vi "ControlProgram6.6_3.vi"() -> ()   [LabVIEW 2016]
uses:
  <vilib>/Utility/miscctls.llb/LVPoint32TypeDef.ctl
  <vilib>/Platform/TimedLoop/XDataNode/timing_clust.ctl
  <vilib>/Platform/TimedLoop/XDataNode/nitl_modes.ctl
  <vilib>/Platform/TimedLoop/XDataNode/wakeup.ctl
  <vilib>/Instr/_visa.llb/Select Event Type.ctl
  <vilib>/vision/Avi1.llb/AviRefnum.ctl
  <vilib>/Utility/error.llb/DialogType.ctl
  <vilib>/DAQmx/write.llb/DAQmx Write (Analog 1D DBL NChan 1Samp).vi
  <vilib>/DAQmx/read.llb/DAQmx Read (Analog 2D DBL NChan NSamp).vi
  <vilib>/Analysis/baseanly.llb/Mean (DBL).vi
  <vilib>/DAQmx/write.llb/DAQmx Write (Digital Bool 1Line 1Point).vi
  <vilib>/DAQmx/create/channels.llb/DAQmx Create Channel (DO-Digital Output).vi
  <vilib>/DAQmx/create/channels.llb/DAQmx Create Channel (AI-Voltage-Basic).vi
  <vilib>/DAQmx/create/channels.llb/DAQmx Create Channel (AO-Voltage-Basic).vi
  <vilib>/DAQmx/configure/timing.llb/DAQmx Timing (Sample Clock).vi
  <vilib>/DAQmx/miscellaneous.llb/DAQmx Fill In Error Info.vi
  <vilib>/Instr/_visa.llb/VISA Configure Serial Port (Instr).vi
  Arnulf--joystick/git(most_up_to_date)/Logitech-joystick/Old Trap/FAST_Global_var.vi
  <vilib>/Utility/inputDevices.llb/mouseAcquire.vi
  <vilib>/Utility/inputDevices.llb/closeMouse.vi
  <vilib>/platform/TimedLoop/XDataNode/XDataNode.xnode
  <vilib>/Platform/TimedLoop/XDataNode/XDNodeRunTimeDep.lvlib
  <resource>/objmgr/daqmx.rc
  <vilib>/Analysis/NI_AALBase.lvlib
panel:
  out "Saving Move":bool
  out "Move time":string
  out "Primary Video Display":T1(plugin-control)
  in  "Save file index":i32
  out "Flush Sample Start Time":u32=2111292881
  out "Sample flush time (s)":dbl=48.0
  in  "Inject Sample":bool
  out "Cal values":T2={"AX alpha"=612.9626061060078, "BX alpha"=549.6584469744151, "AX kappa"=0.3485731373010688, "BX kappa"=0.3853424216291352, "AX offset"=-0.03900484438240665, "BX offset"=-0.11295550662085417, "AY alpha"=582.7562541114835, "BY alpha"=571.1587543790358, "AY kappa"=0.37498408087930674, "BY kappa"=0.36252029651198364, "AY offset"=-0.21125584642206058, "BY offset"=-0.12469077200400738}
  in  "Inject Pump 1":bool
  in  "Inject Pump 2":bool
  in  "Tab Control 2":T3(tab)
  in  "Force FB script":bool
  in  "Got ADig bead":bool
  in  "Move Cap. 2 (ADig Top)":bool
  in  "Dump beads":bool
  in  "Got DNA bead":bool
  in  "Flow on\ncap 2?":bool=TRUE
  in  "Flow on\ncap 1?":bool=TRUE
  in  "Flow on\ndump?":bool=TRUE
  in  "Raster set":i32=1
  in  "Fish After TA?":bool=TRUE
  in  "Delta after tether":dbl=1700.0
  in  "TA Cancel Save?":bool=TRUE
  in  "Min fish\ndelta (nm)":dbl=1425.0 min=0.0 max=5000.0 step=50.0
  in  "Max fish\ndelta (nm)":dbl=1900.0 min=0.0 max=5000.0 step=25.0
  in  "Fish Speed (ms)":i32=5000
  in  "Wait (ms)":i32=1500
  in  "# attempts":dbl=10.0
  in  "Cutoff force (pN)":dbl=4.5
  in  "Raster after\n tether?":bool=TRUE
  out "Tether":bool
  out "Attempt #":i32
  in  "Flow on\nwhile fish?":bool=TRUE
  in  "Flow on\nafter raster?":bool=TRUE
  in  "Offset raster set":i32
  in  "Offset @ Delta (nm)":dbl=1700.0
  in  "Cal @ Delta (nm)":dbl=2500.0
  in  "Cal stage position":i32=3
  out "Cal Final Sampling Rate":dbl=125000.0
  in  "Cal Averaging":i32=1
  in  "Wait before dip (s)":dbl=3.0
  in  "Start dipping after?":bool
  in  "Start trap delta (nm)":dbl=1700.0
  in  "Continous Dip":bool
  out "Dip #":i32
  in  "Dip attempts":dbl=3.0
  in  "Cancel Dip":bool
  out "Return elasped time":i32
  in  "Return duration":dbl=15.0
  in  "Cancel dwell":bool=TRUE
  in  "Pause dwell":bool
  in  "Start/Return position":dbl=3.0
  in  "Dip duration":dbl=15.0
  in  "Dip position":dbl=4.0
  in  "Dip":bool
  out "Dip elasped time":i32
  in  "Stop":bool=TRUE
  in  "?":T4(tab)
  out "FAST X-Y":bool
  out "FAST Z":bool
  in  "Cal time (s)":dbl=5.0
  in  "Save N sets":bool
  in  "N sets":i32=200
  out "Cal sets to save":i32=500
  in  "Reset data stream":bool
  out "Buffer Overflow":bool
  out "Stage moving":bool
  in  "Comment":string
  in  "Raster scan":bool
  out "Saving":bool
  in  "Save cal":bool
  in  "Save Data":bool
  in  "Stop saving":bool
  out "Calibrating":bool
  out "Progress":dbl(slide) scale=0.0..100.0
  in  "Read Cal":bool
  in  "Fish":bool
  in  "Averaging Number":i32=1250
  out "Final Sampling Rate":dbl=100.0
  in  "Trap position (V)":cluster{"X":dbl, "Y":dbl}={"X"=3.9042624789680316, "Y"=0.2}
  in  "Trap delta (nm)":dbl=2500.0 min=0.0 max=5000.0 step=50.0
  in  "Fixed X":dbl=1.1
  in  "Fixed Y":dbl=0.15
  in  "Shutter 1 (B)":bool
  in  "Shutter 2 (A)":bool
  in  "Pulling direction":bool
  out "Raster scanning...":bool
  out "Current file name":path=path "D:/data/160111/160111_006.dat"
  in  "AX alpha":dbl=612.9626061060078 format="%#_3p"
  in  "BX alpha":dbl=549.6584469744151 format="%#_3g"
  in  "AX kappa":dbl=0.3485731373010688 format="%#_3g"
  in  "BX kappa":dbl=0.3853424216291352 format="%#_3g"
  in  "AX offset":dbl=-0.03900484438240665 format="%#_3g"
  in  "BX offset":dbl=-0.11295550662085417 format="%#_3g"
  in  "AY alpha":dbl=582.7562541114835 format="%#_3g"
  in  "BY alpha":dbl=571.1587543790358 format="%#_3g"
  in  "AY kappa":dbl=0.37498408087930674 format="%#_3g"
  in  "BY kappa":dbl=0.36252029651198364 format="%#_3g"
  in  "AY offset":dbl=-0.21125584642206058 format="%#_3g"
  in  "BY offset":dbl=-0.12469077200400738 format="%#_3g"
  out "Buffer status":u8(slide) scale=0.0..100.0
  in  "Target":bool
  in  "Set Current\nPos to (0,0,0)":bool
  in  "dump spot":string="Dump beads spot"
  in  "up flow spot":string="Upper flow spot"
  in  "low flow spot":string="Lower flow spot"
  in  "up cap":string="Upper capillary (ADig beads)"
  in  "bottom cap":string="Lower capillary (DNA beads)"
  in  "Move to Position 5":bool
  in  "Set Position 5":bool
  in  "Saved stage positions":dbl[][](array[numeric])=[[1.0, 0.0, 0.0, 0.0], [2.0, -0.13716, -3.21132, 0.01436], [3.0, 0.45, -0.73974, 0.005], [4.0, 0.45, -2.1978, 0.005], [5.0, 0.45, -2.63158, -0.02256]]
  in  "Set Position 2":bool
  in  "Move to Position 2":bool
  in  "Set Position 1":bool
  in  "Move to Position 1":bool
  in  "Set Position 4":bool
  in  "Move to Position 4":bool
  in  "Set Position 3":bool
  in  "Move to Position 3":bool
  out "Stage error":errorcluster
  in  "Clear Volume":bool
  out "Sample Flush Meter":u8(slide) scale=0.0..100.0
  out "Flushing Sample":bool
  in  "Flush Sample":bool
  in  "Normal \nRate (ul/hr)  3":dbl=100.0
  in  "Normal \nVolume (ul) 3":dbl=250.0
  in  "Normal \nVolume (ul) 2":dbl
  in  "Normal \nRate (ul/hr)":dbl
  in  "Normal \nVolume (ul)":dbl
  in  "Flush\nRate (ul/min)":dbl
  in  "Flush\nVolume (ul)":dbl
  in  "Flush \nRate (ul/min)  2":dbl
  in  "Flush Pump 2":bool
  in  "Flush\nVolume (ul)  2":dbl
  in  "Flush Pump 1":bool
  in  "Normal \nRate (ul/hr)  2":dbl
  in  "Write Wait":i32=1000
  in  "Flush \nRate (ul/min)  3":dbl=100.0
  in  "Flush\nVolume (ul)  3":dbl=80.0
  out "error out":errorcluster
  in  "Use Mouse to Move Trap?":bool
  in  "Pause Mouse/Mirror Connection":bool
  out "Reference Voltage":cluster{dbl, dbl}={0.0, -0.0}
  out "Saved voltage":cluster{dbl, dbl}={5.766666666666665, 1.45}
  out "Real Coordinates":cluster{"Horizontal":i32, "Vertical":i32}={"Horizontal"=897, "Vertical"=-1271}
  out "CoordinatesMousePressed":T5
  in  "Force Feedback 2":bool
  in  "Offset 2":cluster{"Off Y":dbl, "Off X":dbl}={"Off Y"=1.5, "Off X"=0.17}
  in  "Setpoint voltage 2":cluster{"SP Y":dbl, "SP X":dbl}={"SP Y"=0.6, "SP X"=0.0}
  out "Sum error":dbl(knob) scale=-0.2..0.2
  out "Trap sep":waveform(dbl)[](graph)=[{"t0"=timestamp(4.489999999999949 s since 1904-01-01), "dt"=0.002, "Y"=[-1157.7639781743756, -1157.678951177374, -1157.7582331070425, -1157.7490409992681, -1157.8995617642552], "attributes"=variant("NI_ChannelName"=variant(string "T2 X"))}, {"t0"=timestamp(4.489999999999949 s since 1904-01-01), "dt"=0.002, "Y"=[-909.0775466981794, -909.1316439023619, -909.1322956759037, -909.1570630705896, -909.1264297140281], "attributes"=variant("NI_ChannelName"=variant(string "T2 Y"))}]
  in  "Set reading to\nsetpoint 1":bool
  in  "Offset Y (nm)":dbl format="%0.2f"
  in  "Offset X (nm)":dbl format="%0.2f"
  in  "Remove offsets":bool
  in  "Force Feedback 1":bool
  out "Feedback Output \nVoltage 2":cluster{dbl, dbl} {"?" format="%#_4g"; "?" format="%#_4g"}
  in  "Offset 1":cluster{"Off Y":dbl, "Off X":dbl}={"Off Y"=1.5, "Off X"=0.17}
  in  "Setpoint voltage 1":cluster{"SP Y":dbl, "SP X":dbl}={"SP Y"=0.6, "SP X"=0.0}
  in  "Feedback const":T6={"Ki_B_Y"=0.5, "Ki_B_X"=0.0, "Kp Y"=1.0, "Kp X"=0.0}
  out "Mean Trap Pos X 2 (nm)":dbl=-1157.769953044463 format="%0.2f"
  out "Mean Trp Pos Y 2 (nm)":dbl=-909.1249958122125 format="%0.2f"
  out "T2 X RMS (A)":dbl=0.7168002469275427 format="%0.2f"
  out "T2 Y RMS (A)":dbl=0.25997187037503383 format="%0.2f"
  in  "Set reading to\nsetpoint 2":bool
  in  "Scan range (nm)":dbl=425.0
  in  "Scan speed (nm/s)":dbl=100.0 min=0.0 max=100.0
  in  "Step size (nm)":dbl=1.0
  in  "Save scans":bool=TRUE
  in  "# scans":i32=1
  in  "Load param":bool
  in  "Scan Parameters":T7(array[cluster])
  in  "Trap delta\nafter (nm)":dbl=1550.0
  in  "Stop raster":bool
  out "Scan range (V)":dbl=0.47672462142456534
  out "Scan steps (mirror)":u64=425
  out "Scan increment (V)":dbl=0.0011217049915872126
  out "Time per step (ms)":dbl=10.0
  out "Total raster time (s)":dbl=8.5
  out "N sets to be saved":dbl=850.0
  in  "Zoom Factor":sgl=7.0
  in  "Center Point":cluster{"X":i32, "Y":i32}={"X"=335, "Y"=271}
  in  "Intensity Upper":dbl=88.0
  in  "Intensity Lower":dbl=66.0
  out "Window Size":cluster{"Height":i32, "Width":i32}
  in  "Image Index":dbl=1.0 min=1.0
  in  "Save Image":bool
  in  "Averaging":bool
  in  "Reset Averaging":bool
  in  "Save Video":bool
  in  "New Video File":bool
  in  "Video Index":dbl=1.0 min=1.0 step=1.0
  in  "Video Capture Rate (Hz)":dbl=30.0
  in  "Initial Window Size":cluster{"Width":i32, "Height":i32}={"Width"=884, "Height"=619}
  in  "Initial Window Position":cluster{"X Position":i32, "Y Position":i32}={"X Position"=796, "Y Position"=4}
  out "Window Position":cluster{"X Position":i32, "Y Position":i32}={"X Position"=40, "Y Position"=40}
  out "Path Out":path
  in  "Target coordinates":cluster{"X1":dbl, "Y1":dbl, "X2":dbl, "Y2":dbl}={"X1"=328.0, "Y1"=274.0, "X2"=368.0, "Y2"=314.0}
  in  "# Samples/channel (in)":i32=40000 format="%.2f"
  out "Buffer size\n(Samples/channel)":u32=511
  out "DAQ rate\n(Samples/s)":dbl=125000.0 format="%#_6p"
  out "# Samples/channel":i32=1250
  out "# Samples/channel/s":dbl=100.0
  out "AvailSampPerChan":u32=9
  out "Data update period (s/set)":dbl=0.01 format="%#_6p"
  out "AvailSampPerChan 2":u32=110
  in  "PC samp per channel":i32=1000
  in  "Sampling Rate":dbl=125000.0 format="%0.0p"
  in  "DAQ Rate2":dbl=1000000.0 format="%#_6p"
  out "Data period (s)":dbl=8e-06 format="%#_6p"
  in  "Save user params":bool
  in  "User":string(combo)
  in  "Load user params":bool
  in  "Tether break\nforce (pN)":dbl=1.0
  in  "Path":path=path "E:/Data"
  out "Mirror task":refnum<k21>
  in  "Conv X (nm/V)":dbl=891.5
  in  "Conv Y (nm/V)":dbl=505.7
  in  "Min value Y":dbl format="%.1g"
  in  "Max value Y":dbl=10.0 format="%.1f"
  in  "Min value X":dbl format="%0.1f"
  in  "Max value X":dbl=10.0 format="%.1f"
  in  "HWP1":string="Half waveplate 1: differential trap power"
  in  "HWP0":string="Half waveplate 0: total trap power"
  in  "Move 1":bool
  in  "\"Degrees\" 1":dbl
  in  "Move 0":bool
  in  "\"Degrees\" 0":dbl
  in  "Y command":enum16{"Fish", "Dump", "Got ADig", "Got DNA"}(ring)
  in  "B command":enum16{"Got DNA", "Got ADig", "Dump", "Fish"}(ring)
  in  "A command":enum16{"Got ADig", "Dump", "Fish", "Got DNA"}(ring)
  in  "X command":enum16{"Dump", "Fish", "Got ADig", "Got DNA"}(ring)
  out "Logitech":bool
  out "START":bool
  out "BACK":bool
  out "Right stick button":bool
  out "Left Y":i8(slide) scale=-128.0..127.0
  out "Left X":i8(slide) scale=-128.0..127.0
  out "Right Y":i8(slide) scale=-128.0..127.0
  out "Right X":i8(slide) scale=-128.0..127.0
  out "X":bool
  out "Y":bool
  out "A":bool
  out "B":bool
  out "RB":bool
  out "LB":bool
  out "R":bool
  out "L":bool
  out "D":bool
  out "U":bool
  out "Left stick button":bool
  out "FAST Z":bool
  out "FAST X-Y":bool
  in  "XY Speed Definitions":T8={"Slow X velocity input"="0.05", "Slow Y velocity input"="0.05", "Fast1 X velocity input"="0.1", "Fast1 Y velocity input"="0.1", "Fast2 X velocity input"="0.2", "Fast2 Y velocity input"="0.2"}
  in  "Z Speed Definitions":cluster{"Slow Z":string, "Fast Z":string}={"Slow Z"="0.025", "Fast Z"="0.05"}
  in  "Z Wait time":string="120"
  in  "X-Y Wait time":string="125"
  in  "USB port":refnum<visa-resource-name>="USB0::0x046D::0xC21D::CC66247B::RAW"
  out "Deflection":T5
  in  "Sampling Rate":dbl=125000.0 format="%0.2f"
  in  "Averaging Number":i32=12500
  in  "DAQ Rate":dbl=1000000.0
  out "Final Sampling Rate":dbl
  in  "Tab Control":T9(tab)
  in  "Downsamp\nfact":dbl=250.0
  out "Bead sep":waveform(dbl)[](graph)=[{"t0"=timestamp(4.489999999999949 s since 1904-01-01), "dt"=0.002, "Y"=[8093.963535945606, 8103.1617772716045, 8385.72390184118, 8245.733099167523, 8154.925676756515], "attributes"=variant("NI_ChannelName"=variant(string "T2"))}, {"t0"=timestamp(4.489999999999949 s since 1904-01-01), "dt"=0.002, "Y"=[1717.924930434114, 1628.723007842151, 1787.6888378897193, 1598.475730715916, 1776.2517588078954], "attributes"=variant("NI_ChannelName"=variant(string "T1"))}]
  out "Force (pN)":waveform(dbl)[](graph)=[{"t0"=timestamp(4.489999999999949 s since 1904-01-01), "dt"=0.002, "Y"=[2821.5994183803123, 2824.8226375853515, 2923.3663028678166, 2874.5254578927593, 2842.869034836209], "attributes"=variant("NI_ChannelName"=variant(string "T2"))}, {"t0"=timestamp(4.489999999999949 s since 1904-01-01), "dt"=0.002, "Y"=[623.5850847499229, 591.0680427774053, 648.761979867749, 579.944408346982, 644.7436619059413], "attributes"=variant("NI_ChannelName"=variant(string "T1"))}]
  out "Mean force (pN)":dbl=1737.5286029210451 format="%0.2f"
  out "Force noise (pN)":dbl=26.83032703631318 format="%0.2f"
  out "Mean Bead Sep\n(nm)":dbl=4949.257225667222 format="%0.2f"
  out "Bead Sep Noise\n(A)":dbl=757.8078481959694 format="%0.2f"
  out "PSD 2":cluster{dbl[], dbl[]}(graph)
  out "PSD 1":cluster{dbl[], dbl[]}(graph)
  out "PSD 1 Sum":dbl(slide) scale=0.0..10.0
  out "PSD 2 Sum":dbl(slide) scale=0.0..10.0
  in  "Start":bool
  out "All signals 2":waveform(dbl)[](graph)=[{"t0"=timestamp(4.489999999999949 s since 1904-01-01), "dt"=0.002, "Y"=[0.0010396217068286443, 0.0010666908927528754, 0.001103298744846499, 0.0010651440823993424, 0.0010656596859401936], "attributes"=variant("NI_ChannelName"=variant(string "A y"))}, {"t0"=timestamp(4.489999999999949 s since 1904-01-01), "dt"=0.002, "Y"=[0.02000680227246931, 0.020097032918054827, 0.02003412926844257, 0.020136734401221615, 0.020087494249822452], "attributes"=variant("NI_ChannelName"=variant(string "A x"))}, {"t0"=timestamp(4.489999999999949 s since 1904-01-01), "dt"=0.002, "Y"=[-0.0014958587831537804, -0.0015046240440107857, -0.0014930229638311983, -0.001533240041751485, -0.0015262793936602433], "attributes"=variant("NI_ChannelName"=variant(string "B y"))}, {"t0"=timestamp(4.489999999999949 s since 1904-01-01), "dt"=0.002, "Y"=[0.0002901198559372817, 0.0002731049385577592, 0.00026511308349727467, 0.0002517073909711183, 0.0002916666665966012], "attributes"=variant("NI_ChannelName"=variant(string "B x"))}, {"t0"=timestamp(4.489999999999949 s since 1904-01-01), "dt"=0.002, "Y"=[-0.001511556786147372, -0.0015167122027053212, -0.0014612914746018214, -0.0014935128282145193, -0.0015064013696263116], "attributes"=variant("NI_ChannelName"=variant(string "A sum"))}, {"t0"=timestamp(4.489999999999949 s since 1904-01-01), "dt"=0.002, "Y"=[-0.0005242945138364382, -0.0005565158674093218, -0.000501095139248956, -0.0005771375336978897, -0.0005165613890095197], "attributes"=variant("NI_ChannelName"=variant(string "B sum"))}, {"t0"=timestamp(4.489999999999949 s since 1904-01-01), "dt"=0.002, "Y"=[0.0013303666019343777, 0.0014257418088905328, 0.0013368108726387405, 0.0013471217058124534, 0.0011782818123890176], "attributes"=variant("NI_ChannelName"=variant(string "Trap x"))}, {"t0"=timestamp(4.489999999999949 s since 1904-01-01), "dt"=0.002, "Y"=[0.0023382505474007294, 0.002231275652833831, 0.002229986798687363, 0.0021810103409340116, 0.002241586486003531], "attributes"=variant("NI_ChannelName"=variant(string "Trap y"))}]
  out "All signals":waveform(dbl)[](graph)=[{"t0"=timestamp(4.489999999999949 s since 1904-01-01), "dt"=0.002, "Y"=[0.0010396217068286443, 0.0010666908927528754, 0.001103298744846499, 0.0010651440823993424, 0.0010656596859401936], "attributes"=variant("NI_ChannelName"=variant(string "A y"))}, {"t0"=timestamp(4.489999999999949 s since 1904-01-01), "dt"=0.002, "Y"=[0.02000680227246931, 0.020097032918054827, 0.02003412926844257, 0.020136734401221615, 0.020087494249822452], "attributes"=variant("NI_ChannelName"=variant(string "A x"))}, {"t0"=timestamp(4.489999999999949 s since 1904-01-01), "dt"=0.002, "Y"=[-0.0014958587831537804, -0.0015046240440107857, -0.0014930229638311983, -0.001533240041751485, -0.0015262793936602433], "attributes"=variant("NI_ChannelName"=variant(string "B y"))}, {"t0"=timestamp(4.489999999999949 s since 1904-01-01), "dt"=0.002, "Y"=[0.0002901198559372817, 0.0002731049385577592, 0.00026511308349727467, 0.0002517073909711183, 0.0002916666665966012], "attributes"=variant("NI_ChannelName"=variant(string "B x"))}, {"t0"=timestamp(4.489999999999949 s since 1904-01-01), "dt"=0.002, "Y"=[-0.001511556786147372, -0.0015167122027053212, -0.0014612914746018214, -0.0014935128282145193, -0.0015064013696263116], "attributes"=variant("NI_ChannelName"=variant(string "A sum"))}, {"t0"=timestamp(4.489999999999949 s since 1904-01-01), "dt"=0.002, "Y"=[-0.0005242945138364382, -0.0005565158674093218, -0.000501095139248956, -0.0005771375336978897, -0.0005165613890095197], "attributes"=variant("NI_ChannelName"=variant(string "B sum"))}, {"t0"=timestamp(4.489999999999949 s since 1904-01-01), "dt"=0.002, "Y"=[0.0013303666019343777, 0.0014257418088905328, 0.0013368108726387405, 0.0013471217058124534, 0.0011782818123890176], "attributes"=variant("NI_ChannelName"=variant(string "Trap x"))}, {"t0"=timestamp(4.489999999999949 s since 1904-01-01), "dt"=0.002, "Y"=[0.0023382505474007294, 0.002231275652833831, 0.002229986798687363, 0.0021810103409340116, 0.002241586486003531], "attributes"=variant("NI_ChannelName"=variant(string "Trap y"))}]
  out "Chart Freq (Hz)":dbl=500.0
  # "Bead Calibration"
  # "Y"
  # "X"
  # "Pump #1 Controls"
  # "Pump #2 Controls"
  # "Sample Pump Controls"
  # "Retract the pumps manually. Change it back to INFUSE when you're done. Suck it up, don't whine."
  # "Shutter 1 (B)"
  # "Move to Lower Cap"
  # "Inject Sample"
  # "Move to Upper Cap"
  # "Shutter 2 (A)"
  # "Select the Joystick input:"
  # "Overflow happens when >40 commands\nsent in 5 seconds. Then 4 consecutive beeps."
  # "Try increasing wait time to reduce 'following error threshold exceeded' occurances."
  # "Left stick controls Z axis.\nRight on stick: neg Z-dir\nUp on stick: neg Z-dir"
  # "Toggles FAST Z"
  # "Toggles FAST X-Y"
  # "The default Newport max velocity is 0.4"
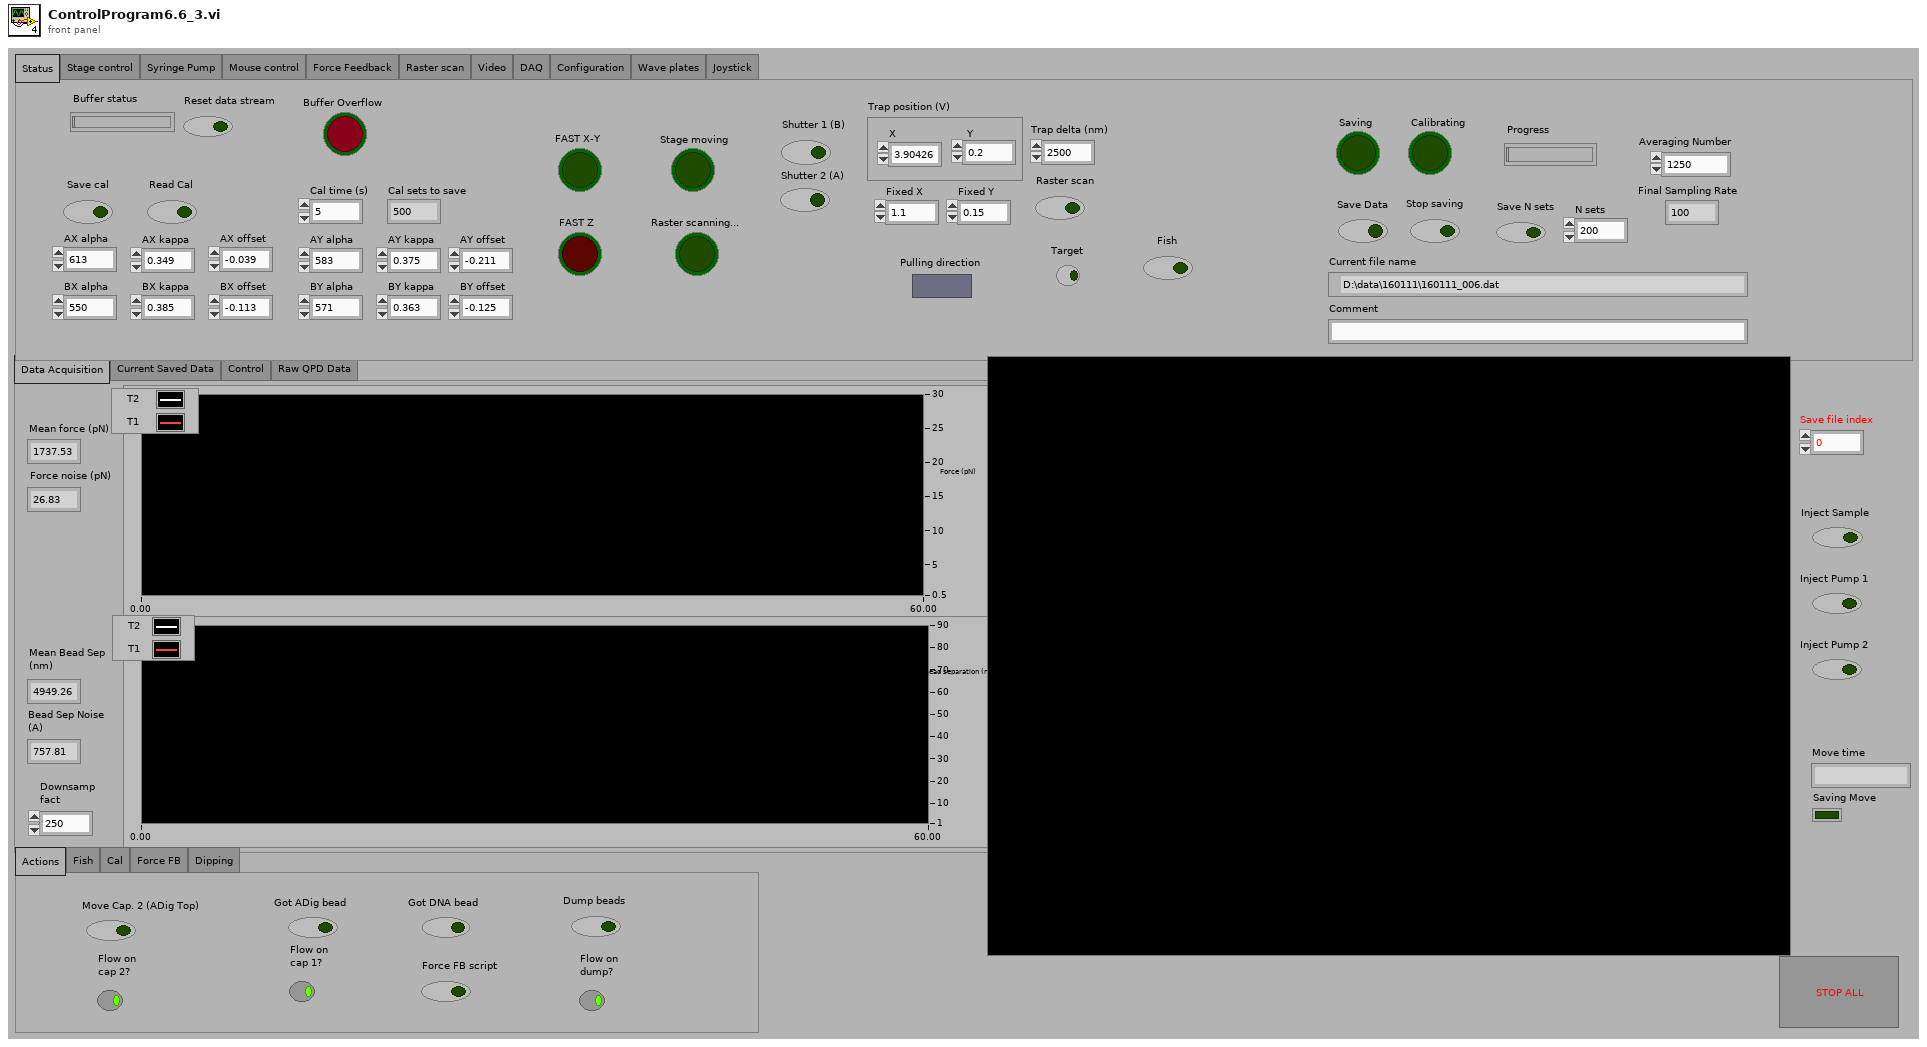
[diagram p1: front panel]
types:
  T1 = typedef "IMAQ Image.ctl" = refnum<image>
  T2 = cluster{"AX alpha":dbl, "BX alpha":dbl, "AX kappa":dbl, "BX kappa":dbl, "AX offset":dbl, "BX offset":dbl, "AY alpha":dbl, "BY alpha":dbl, "AY kappa":dbl, "BY kappa":dbl, "AY offset":dbl, "BY offset":dbl}
  T3 = enum32{"Actions", "Fish", "Cal", "Force FB", "Dipping"}
  T4 = enum32{"Status", "Stage control", "Syringe Pump", "Mouse control", "Force Feedback", "Raster scan", "Video", "DAQ", "Configuration", "Wave plates", "Joystick"}
  T5 = typedef "LVPoint32TypeDef.ctl" = cluster{"Horizontal":i32, "Vertical":i32}
  T6 = cluster{"Ki_B_Y":dbl, "Ki_B_X":dbl, "Kp Y":dbl, "Kp X":dbl}
  T7 = cluster{"Label":string, "Scan range 1":dbl, "Step size 1":dbl, "Scan speed 1":i32, "# scans 2":i32}[]
  T8 = cluster{"Slow X velocity input":string, "Slow Y velocity input":string, "Fast1 X velocity input":string, "Fast1 Y velocity input":string, "Fast2 X velocity input":string, "Fast2 Y velocity input":string}
  T9 = enum32{"Data Acquisition", "Current Saved Data", "Control", "Raw QPD Data"}
  T10 = typedef "Select Event Type.ctl" = u32
  T11 = enum32{"setting", "request", "request control", "info", "statistics", "system settings", "I/O sub system", "HRT control", "camera descriptions", "device specific data", "event sub system settings", "event sub system results", "image memory manager"}
  T12 = typedef "AviRefnum.ctl" = refnum<k1>
  T13 = typedef "XDNodeRunTimeDep.lvlib/timing_clust.ctl" = cluster{"Expected End [f-1]":u64, "Actual End [f-1]":u64, "Finished Late? [f-1]":bool, "Expected End [i-1]":u64, "Actual End [i-1]":u64, "Finished Late? [i-1]":bool, "Expected Start [i]":u64, "Actual Start [i]":u64, "Expected Start [f]":u64, "Actual Start [f]":u64, "Source Name":string, "Structure Name":string, "Period":i64, "Deadline":i64, "Offset":i64, "Start":i64, "Priority":i32, "Timeout":i32, "Mode":T14, "Wakeup Reason":T15, "Error":errorcluster, "Source Type":string, "Secondary Source Type":string, "Global End Time":u64, "Global Start Time":u64, "Frame Duration":u64, "Iteration Duration":u64, "Assigned CPU":i32, "I/O Scan Engine Mode":u32}
  T14 = typedef "XDNodeRunTimeDep.lvlib/nitl_modes.ctl" = enum32{"No Change", "Process missed periods, maintain original phase", "Discard missed periods, maintain original phase", "Process missed periods, ignore original phase", "Discard missed periods, ignore original phase"}
  T15 = typedef "XDNodeRunTimeDep.lvlib/wakeup.ctl" = enum32{"Normal", "Aborted", "Asynchronous wakeup", "Timing source error", "Timed loop error", "Timeout"}
  T16 = typedef "Image Type" = u32
  T17 = typedef "imagedata.ctl" = cluster{"image type":i32, "image depth":i32, "image":u8[], "mask":u8[], "colors":u32[], "Rectangle":cluster{"left":i16, "top":i16, "right":i16, "bottom":i16}}
  T18 = enum16{"open", "replace", "create", "open or create", "replace or create", "replace or create with confirmation"}
  T19 = enum16{"big-endian, network order", "native, host order", "little-endian"}
  T20 = cluster{string, string, string, string, string, string, string, string}
  T21 = cluster{"LB":bool, "RB":bool, "BACK":bool, "Logitech":bool, "START":bool}
  T22 = cluster{"Right X":i8, "Right Y":i8, "Left X":i8, "Left Y":i8}
  T23 = enum32{"Status", "Stage control", "Syringe Pump", "Mouse control", "Force Feedback", "Raster scan", "Video", "DAQ", "Configuration", "Wave plates"}
  T24 = typedef "DialogType.ctl" = u16
  T25 = cluster{"button 1":bool, "button 2":bool, "button 3":bool, "button 4":bool}
  T26 = cluster{"[0]":dbl, "[1]":dbl, "[2]":dbl, "[3]":dbl, "[4]":dbl, "[5]":dbl, "[6]":dbl, "[7]":dbl, "[8]":dbl, "[9]":dbl, "[10]":dbl, "[11]":dbl}
  T27 = cluster{"Label":string, "Scan range 1":dbl, "Step size 1":dbl, "Scan speed 1":i32, "# scans 2":i32}
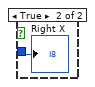
[diagram p5: hidden frame]
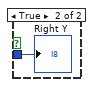
[diagram p6: hidden frame]
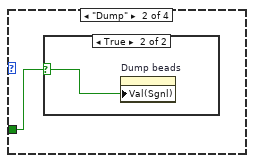
[diagram p10: hidden frame]
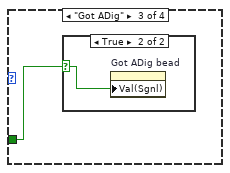
[diagram p12: hidden frame]
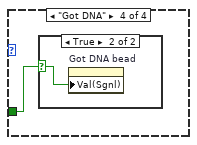
[diagram p14: hidden frame]
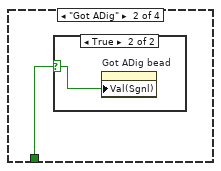
[diagram p17: hidden frame]
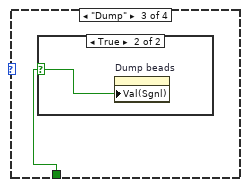
[diagram p19: hidden frame]
diagram:
  w10 = T10 1073684535 items=["Service Request"=1073684491, "Trigger"=3221168138, "Clear"=1073684493, "VXI Signal"=1073684512, "VXI/VME Interrupt"=3221168161, "VXI/VME Sysfail"=1073684509, "VXI/VME Sysreset"=1073684510, "GPIB CIC"=1073684498, "GPIB Talk"=1073684499, "GPIB Listen"=1073684500, "PXI Interrupt"=1073684514, "Serial Break"=1073684515, "Serial TermChar"=1073684516, "Serial CTS"=1073684521, "Serial DSR"=1073684522, "Serial DCD"=1073684524, "Serial RI"=1073684526, "Serial Character"=1073684533, "USB Interrupt"=1073684535, "All Enabled"=1073709055] ("Event Type")
  w49 = 10.0 ("Minimum Value")
  w50 = -10.0 ("Minimum Value")
  w52 = -2.0 ("Minimum Value")
  w53 = 2.0 ("Maximum Value")
  w78 = 10123 items=["Finite Samples"=10178, "Continuous Samples"=10123] ("sample mode")
  w98 = tag "Dev1/port2/line1"  # Shutter 2
  w101 = tag "Dev1/port1/line4"  # Shutter 1
  # "Open the RAW resource"
  # "Enable USB Interrupt Event"
  # "Create channels for movable mirror"
  # "Create channels for detectors"
  n1 = call-poly <vilib>:"DAQmx Create Virtual Channel.vi"("maximum value"=w53, "minimum value"=w52, "physical channels"=tag "Dev1/ai0" ("Physical Channel")) -> ("task out"=w54:refnum<k21>, "error out"=w77:errorcluster)  [unwired: 11 in]
  n2 = call-poly <vilib>:"DAQmx Create Virtual Channel.vi"("task in"=w54, "maximum value"=w53, "minimum value"=w52, "physical channels"=tag "Dev1/ai1", "error in"=w77) -> ("task out"=w75:refnum<k21>, "error out"=w74:errorcluster)  [unwired: 9 in]
  n3 = call-poly <vilib>:"DAQmx Create Virtual Channel.vi"("task in"=w75, "maximum value"=w53, "minimum value"=w52, "physical channels"=tag "Dev1/ai2", "error in"=w74) -> ("task out"=w66:refnum<k21>, "error out"=w65:errorcluster)  [unwired: 9 in]
  n4 = call-poly <vilib>:"DAQmx Create Virtual Channel.vi"("task in"=w66, "maximum value"=w53, "minimum value"=w52, "physical channels"=tag "Dev1/ai3" ("Physical Channel"), "error in"=w65) -> ("task out"=w51:refnum<k21>, "error out"=w71:errorcluster)  [unwired: 9 in]
  n5 = call-poly <vilib>:"DAQmx Create Virtual Channel.vi"("task in"=w51, "maximum value"=w49, "minimum value"=w50, "physical channels"=tag "Dev1/ai4", "error in"=w71) -> ("task out"=w69:refnum<k21>, "error out"=w68:errorcluster)  [unwired: 9 in]
  n6 = call-poly <vilib>:"DAQmx Create Virtual Channel.vi"("task in"=w69, "maximum value"=w49, "minimum value"=w50, "physical channels"=tag "Dev1/ai5", "error in"=w68) -> ("task out"=w64:refnum<k21>, "error out"=w63:errorcluster)  [unwired: 9 in]
  n7 = call-poly <vilib>:"DAQmx Create Virtual Channel.vi"("task in"=w64, "maximum value"=w49, "minimum value"=w50, "physical channels"=tag "Dev1/ai6", "error in"=w63) -> ("task out"=w58:refnum<k21>, "error out"=w56:errorcluster)  [unwired: 9 in]
  n8 = call-poly <vilib>:"DAQmx Create Virtual Channel.vi"("task in"=w58, "maximum value"=w49, "minimum value"=w50, "physical channels"=tag "Dev1/ai7", "error in"=w56) -> ("task out"=w57:refnum<k21>, "error out"=w55:errorcluster)  [unwired: 9 in]
  n9 = call-poly <vilib>:"DAQmx Timing.vi"("task/channels in"=w57, "sample mode"=w78, "samples per channel"="PC samp per channel", "rate"="Sampling Rate", "error in"=w55) -> ("task out"=w61:refnum<k21>, "error out"=w60:errorcluster)  [unwired: 9 in]
  n10 = call-poly <vilib>:"DAQmx Create Virtual Channel.vi"("maximum value"="Max value Y", "minimum value"="Min value Y", "physical channels"=tag "Dev1/ao1" ("Trap X Axis")) -> ("task out"=w46:refnum<k21>, "error out"=w48:errorcluster)  [unwired: 11 in]
  n11 = property class="DAQmx Timing"(reference=w61, error in=w60, "More:AI Convert:Rate"="DAQ Rate2") -> (reference out=w19:refnum<k21>, error out=w18:errorcluster, "SampClk.Rate"=→"DAQ rate\n(Samples/s)":dbl)
  n12 = call-poly <vilib>:"DAQmx Create Virtual Channel.vi"("task in"=w46, "maximum value"="Max value X", "minimum value"="Min value X", "physical channels"=tag "Dev1/ao0" ("Trap Y Axis"), "error in"=w48) -> ("task out"=w37:refnum<k21>, "error out"=w36:errorcluster)  [unwired: 9 in]
  "Mirror task" <- w37
  n13 = property class="DAQmx Buffer"(reference=w19, error in=w18) -> (reference out=w16:refnum<k21>, error out=w15:errorcluster, "Input.OnbrdBufSize"=→"Buffer size\n(Samples/channel)":u32)
  n14 = call <vilib>:"DAQmx Start Task.vi"("task/channels in"=w16, "error in"=w15) -> ("task out"=w38:refnum<k21>)  [unwired: 12 in, 1 out]
  n15 = flat-sequence "Video" {
    tunnel: [w114] -> w13
    tunnel: w13 -> [w155]
    frame #0 {
      n16 = while {
        stop <- w107 continue-if-true
        n17 = call "Close Video Capture.vi"() -> ("error code OUT"=w109:i32)
        n18 = Equal?(x=w109, y=0) -> (x = y?=w107:bool)
      }
      n19 = local write "Stop"(FALSE ("Stop All")) -> ()
    }
    frame #1 {
      n20 = call "DMR_Init.vi"() -> ()  [unwired: 3 out]
    }
    frame #2 {
      # "Setting the destination format to Mono8 makes sure that the image can be displayed in the intensity plot."
      n21 = call "DMR_GetDevice.vi"("search string IN"="DE514724602") -> ("device handle OUT"=w132:i32)  [unwired: 4 in, 2 out]
      n22 = call "DMR_OpenDevice.vi"("device handle IN"=w132) -> ("driver handle OUT"=w115:i32)  [unwired: 4 out]
      n23 = call "DMR_FindList.vi"("flags IN"=u32 0 ("flags"), "list name IN"="" ("String"), "list type IN"=T11."camera descriptions", "driver handle IN"=w115) -> ("list handle OUT"=w118:i32)  [unwired: 2 out]
      n24 = call "DMR_FindList.vi"("flags IN"=u32 0 ("flags"), "list name IN"="Base", "list type IN"=T11."setting", "driver handle IN"=w115) -> ("list handle OUT"=w116:i32)  [unwired: 2 out]
      n25 = call "OBJ_GetHandle.vi"("object name IN"="VideoStandard", "list handle IN"=w118) -> ("object handle OUT"=w112:i32)  [unwired: 3 out]
      n26 = call "OBJ_GetHandle.vi"("object name IN"="PixelFormat", "list handle IN"=w116) -> ("object handle OUT"=w126:i32)  [unwired: 3 out]
      n27 = call "OBJ_SetS.vi"("value index IN"=0, "value IN"="NTSC M", "object handle IN"=w112) -> ()  [unwired: 2 out]
      n28 = call "OBJ_SetS.vi"("value index IN"=0, "value IN"="Mono8" ("value"), "object handle IN"=w126) -> ()  [unwired: 2 out]
      n29 = call "OBJ_GetHandle.vi"("object name IN"="VideoChannel", "list handle IN"=w116) -> ("object handle OUT"=w122:i32)  [unwired: 3 out]
      n30 = while {
        tunnel: [w137] -> w114
        tunnel: w115 -> [w134]
        stop <- w135 continue-if-true
        n31 = call "DMR_ImageRequestSingle.vi"("request control IN"=0, "driver handle IN"=w134) -> ("error code OUT"=w136:i32, "driver handle OUT"=w137:i32)  [unwired: 2 out]
        n32 = Equal To 0?(x=w136) -> (x = 0?=w135:bool)
      }
      n33 = call "OBJ_SetI.vi"("value index IN"=0, "value IN"=0 ("Video channel"), "object handle IN"=w122) -> ()  [unwired: 2 out]
    }
    frame #3 {
      w143 = T16 0 items=["Grayscale (U8)", "Grayscale (I16)", "Grayscale (SGL)", "Complex (CSG)", "RGB (U32)", "HSL (U32)", "RGB (U64)"] ("Image Type")
      w151 = T16 0 items=["Grayscale (U8)", "Grayscale (I16)", "Grayscale (SGL)", "Complex (CSG)", "RGB (U32)", "HSL (U32)", "RGB (U64)"] ("Image Type")
      n34 = for "Create Greyscale map" {
        N: 256 -> [_]
        tunnel: [w157] -> w140 mode=indexing
        workers-P: _ -> [_]
        i -> [w160]
        n35 = To Unsigned Byte Integer(number=w160) -> (unsigned 8bit integer=w156:u8)
        n36 = Join Numbers(hi=w156, lo=w156) -> ((hi.lo)=w159:u16)
        n37 = Join Numbers(hi=w156, lo=w156) -> ((hi.lo)=w158:u16)
        n38 = Join Numbers(hi=w159, lo=w158) -> ((hi.lo)=w157:u32)
      }
      n39 = call "IMAQ Create"("Image Name"="Scaled video", "Image Type"=w143) -> ("New Image"=w142:T1)  [unwired: 2 in, 2 out]
      n40 = call "IMAQ Create"("Image Name"="Main video", "Image Type"=w151) -> ("New Image"=w152:T1)  [unwired: 2 in, 2 out]
      n41 = node-c288(0 ("Processor")) -> (w150:T13)  [unwired: 3 out]
      n42 = Initialize Array(u32 0 ("Window Number (0...15)"), 480 ("dimension size"), 640 ("dimension size")) -> (w145:u32[][])
      n43 = timed-loop {
        tunnel: w155 -> [w177]
        tunnel: [w176] -> w154
        tunnel: w152 -> [w175]
        timing: w150 -> [_]
        timing-out: [_] -> w149
        tunnel: w145 -> [w164]
        tunnel: w142 -> [w162]
        tunnel: w140 -> [w161]
        stop <- w163 stop-if-true
        # "This block performs the \nactual image capture."
        n44 = node-c288() -> ()  [unwired: 2 out]
        n45 = local read "Stop"() -> (w163:bool)
        n46 = Reciprocal(x="Video Capture Rate (Hz)") -> (1/x=w167:dbl)
        n47 = Multiply(x=w167, y=1000.0) -> (x*y=w165:dbl)
        n48 = call "DMR_ImageRequestWaitFor.vi"("queue number IN"=0, "timeout(ms) IN"=500, "driver handle IN"=w177) -> ("error code OUT"=w181:i32, "request number OUT"=w178:i32, "driver handle OUT"=w179:i32)
        n49 = feedback #1(T12 refnum ("Avi Refnum")) -> (w169:T12)
        n50 = case shown="True" "New Video File" {
          tunnel: [T12 refnum ("Avi Refnum") w198] -> w171
          tunnel: [FALSE TRUE] -> w172
          tunnel: w169 -> [_ w194]
          frame False {
          }
          frame True {
            n51 = call "Create new save file.vi"("Ext"=".avi" ("string"), "Index In"="Video Index") -> ("Path Out"=w190:path, "Index Out"=w191:dbl)  [unwired: 1 in]
            "Path Out" <- w190
            n52 = Not Equal?(x=w194, y=T12 refnum ("Avi Refnum")) -> (x != y?=w195:bool)
            n53 = Increment(x=w191) -> (x+1=w200:dbl)
            n54 = case shown="True" w195 {
              tunnel: w194 -> [_ w201]
              frame False {
              }
              frame True {
                n55 = call "IMAQ AVI Close"("Avi Refnum"=w201) -> ()  [unwired: 1 in, 10 out]
              }
            }
            n56 = local write "Video Index"(w200) -> ()
            n57 = call "IMAQ AVI Create"("Frames Per Second"=u32 30, "AVI Path"=w190) -> ("Avi Refnum"=w198:T12)  [unwired: 5 in, 4 out]
          }
        }
        n58 = Equal To 0?(x=w181) -> (x = 0?=w180:bool)
        n59 = Select(t=w171, s=w172, f=w169) -> (s? t:f=w170:T12)
        n60 = feedback-in #1(w170) -> ()
        n61 = case shown="True" w180 {
          tunnel: w179 -> [w202 w229]
          tunnel: w178 -> [_ w228]
          tunnel: [w202 w225] -> w176
          tunnel: w175 -> [_ w206]
          tunnel: w164 -> [_ w213]
          tunnel: w170 -> [_ w211]
          tunnel: w162 -> [_ w207]
          tunnel: w161 -> [_ w208]
          frame False {
          }
          frame True {
            w219 = u32 0 ("X-offset IN")
            n62 = call "DMR_GetImageRequestBufferData.vi"("driver handle IN"=w229, "request number IN"=w228) -> ("width OUT"=w218:i32, "height OUT"=w217:i32, "driver handle OUT"=w224:i32, "request number OUT"=w223:i32, "bytes per pixel OUT"=w220:i32)  [unwired: 13 out]
            n63 = call "DMR_GetImageRequestBufferImageData.vi"("driver handle IN"=w224, "request number IN"=w223, "bytes per pixel IN"=w220, "X-offset IN"=w219, "Y-offset IN"=w219, "height IN"=w217, "width IN"=w218) -> ("driver handle OUT"=w222:u32, "request number OUT"=w221:u32, "image OUT"=w214:u32[][])  [unwired: 10 out]
            n64 = call "DMR_ImageRequestUnlock.vi"("request number IN"=w221, "driver handle IN"=w222) -> ("driver handle OUT"=w227:i32)  [unwired: 1 in, 2 out]
            n65 = case shown="False" "Averaging" {
              tunnel: w214 -> [w270 w275]
              tunnel: [w270 w274] -> w210
              tunnel: w213 -> [_ w272]
              frame False {
              }
              frame True {
                (unwired) 1
                w280 = 1
                n66 = feedback #2(w272) -> (w271:u32[][])
                n67 = Add(x=w275, y=w271) -> (x+y=w276:u32[][])
                n68 = Select(t=w272, s="Reset Averaging", f=w276) -> (s? t:f=w278:u32[][])
                n69 = feedback-in #2(w278) -> ()
                n70 = feedback #3(w280) -> (w273:i32)
                n71 = Divide(x=w276, y=w273) -> (x/y=w277:dbl[][])
                n72 = Increment(x=w273) -> (x+1=w281:i32)
                n73 = To Unsigned Long Integer(number=w277) -> (unsigned 32bit integer=w274:u32[][])
                n74 = Select(t=w280, s="Reset Averaging", f=w281) -> (s? t:f=w279:i32)
                n75 = feedback-in #3(w279) -> ()
              }
            }
            n76 = call "DMR_ImageRequestSingle.vi"("request control IN"=0, "driver handle IN"=w227) -> ("driver handle OUT"=w225:i32)  [unwired: 3 out]
            n77 = disable-structure shown="Disabled" {
              disable-tunnel: w210 -> [w247 _]
              disable-tunnel: w207 -> [w246 _]
              frame Disabled {
                n78 = To Double Precision Float(number=w247) -> (double precision float=w245:dbl[][])
                n79 = In Range and Coerce(upper limit="Intensity Upper", x=w245, lower limit="Intensity Lower") -> (coerced(x)=w244:dbl[][])  [unwired: 1 out]
                n80 = Subtract(x="Intensity Upper", y="Intensity Lower") -> (x-y=w241:dbl)
                n81 = Subtract(x=w244, y="Intensity Lower") -> (x-y=w242:dbl[][])
                n82 = Divide(x=w242, y=w241) -> (x/y=w243:dbl[][])
                n83 = Multiply(x=255.0, y=w243) -> (x*y=w239:dbl[][])
                n84 = To Unsigned Byte Integer(number=w239) -> (unsigned 8bit integer=w248:u8[][])
                n85 = call "IMAQ ArrayToImage"("Image Pixels (U8)"=w248, "Image"=w246) -> ("Image Out"=w235:T1)  [unwired: 4 in, 5 out]
                n86 = First Call?() -> (First Call?: T/F=w236:bool)
                n87 = case shown="True" w236 {
                  tunnel: w235 -> [w249 w260]
                  frame False {
                    n88 = flat-sequence {
                      tunnel: w249 -> [w255]
                      frame #0 {
                        w252 = FALSE ("Get/Set Status? (Set)")
                        w251 = 0 ("Window Number (0...15)")
                        n89 = call "IMAQ WindSize"("Get/Set Status? (Set)"=w252, "Window Number"=w251) -> ("Width & Height out"=→"Window Size":cluster{"Width":i32, "Height":i32})  [unwired: 4 in, 2 out]
                        n90 = call "IMAQ WindMove"("Window Number (0...15)"=w251, "Get/Set Status? (Set)"=w252) -> ("Coordinates (screen)"=→"Window Position":cluster{"X Position":i32, "Y Position":i32})  [unwired: 3 in, 1 out]
                        n91 = call "IMAQ WindDraw"("Resize to Image Size? (Y)"=FALSE, "Window Number (0...15)"=w251, "Image"=w255) -> ()  [unwired: 7 in, 2 out]
                      }
                      frame #1 {
                        n92 = call "IMAQ WindZoom 2"("Center Point"="Center Point", "Zoom to Fit? (False)"=FALSE, "Zoom Factor"="Zoom Factor") -> ()  [unwired: 5 in, 4 out]
                      }
                    }
                  }
                  frame True {
                    n93 = flat-sequence {
                      tunnel: w260 -> [w263]
                      tunnel: [w261] -> w259
                      tunnel: w259 -> [w265]
                      frame #0 {
                        w262 = TRUE ("Resize to Image Size? (Y)")
                        w261 = 0 ("Window Number (0...15)")
                        n94 = call "IMAQ WindNonTearing"("Window Number"=w261, "NonTearing? (True)"=w262) -> ()  [unwired: 8 in, 2 out]
                        n95 = call "IMAQ WindDraw"("Resize to Image Size? (Y)"=w262, "Window Number (0...15)"=w261, "Image"=w263) -> ()  [unwired: 7 in, 2 out]
                      }
                      frame #1 {
                        n96 = call "IMAQ WindSize"("Scrollbars? (N)"=FALSE, "Width & Height"="Initial Window Size", "Window Number"=w265) -> ()  [unwired: 3 in, 3 out]
                        n97 = call "IMAQ WindMove"("Window Number (0...15)"=w265, "Coordinates (screen)"="Initial Window Position") -> ()  [unwired: 3 in, 2 out]
                      }
                    }
                  }
                }
              }
              frame Enabled {
              }
            }
            n98 = To Unsigned Byte Integer(number=w210) -> (unsigned 8bit integer=w209:u8[][])
            n99 = call "IMAQ ArrayToImage"("Image Pixels (U8)"=w209, "Image"=w206) -> ("Image Out"=w204:T1)  [unwired: 4 in, 5 out]
            n100 = case shown="True" "Save Video" {
              tunnel: w211 -> [_ w269]
              tunnel: w204 -> [_ w268]
              frame False {
              }
              frame True {
                n101 = call "IMAQ AVI Write Frame"("Image"=w268, "Avi Refnum"=w269) -> ()  [unwired: 2 in, 8 out]
              }
            }
            n102 = case shown="False" "Save Image" {
              tunnel: w209 -> [_ w284]
              tunnel: w208 -> [_ w283]
              frame False {
              }
              frame True {
                n103 = call <vilib>:"Flatten Pixmap.vi"("colors"=w283, "8-bit pixmap"=w284) -> ("image data"=w290:T17)  [unwired: 4 in, 5 out]
                n104 = call "Create new save file.vi"("Insert"="video_frame_" ("string"), "Ext"=".bmp" ("string"), "Index In"="Image Index") -> ("Path Out"=w286:path, "Index Out"=w291:dbl)
                n105 = Increment(x=w291) -> (x+1=w285:dbl)
                n106 = local write "Image Index"(w285) -> ()
                n107 = call <vilib>:"Write BMP File.vi"("image data"=w290, "path to BMP file"=w286) -> ()  [unwired: 1 in, 9 out]
              }
            }
            n108 = case shown="False" "Target" {
              tunnel: w204 -> [w230 w234]
              tunnel: [w230 w232] -> w203
              frame False {
              }
              frame True {
                n109 = local read "Target coordinates"() -> (w231:cluster{"X1":dbl, "Y1":dbl, "X2":dbl, "Y2":dbl})
                n110 = call "IMAQ Overlay Oval"("Color"=u32 16711680, "Bounding Rectangle"=w231, "Image"=w234) -> ("Image Out"=w232:T1)  [unwired: 7 in, 1 out]
              }
            }
            "Primary Video Display" <- w203
          }
        }
        n111 = node-c288(w165) -> ()  [unwired: 1 out]
      }
      n112 = node-c288(w149) -> ()  [unwired: 1 out]
      n113 = call "DMR_CloseDevice2.vi"("driver handle IN"=w154) -> ()  [unwired: 3 in, 2 out]
    }
    frame #4 {
      n114 = call "DMR_Close.vi"() -> ()  [unwired: 1 out]
    }
  }
  n115 = while {
    tunnel: [w360] -> w84
    tunnel: [w534] -> w85
    tunnel: [w358] -> w83
    tunnel: [w643] -> w80
    tunnel: w38 -> [w345]
    tunnel: w37 -> [w639]
    tunnel: w36 -> [w644]
    stop <- w643 stop-if-true
    w397 = "NI_ChannelName" ("name")
    w301 = "NI_ChannelName" ("name")
    w462 = -1
    # "Negate these value to make Force feedback work in X. 6-14-18 A.T."
    # "BX - AX"
    # "BY - AY"
    # "Scan # counter"
    # "DAQ loop iteration\ncounter (for timing)"
    # "Step counter"
    # "Force feedback"
    # "Raster scan"
    # "Rewire everything"
    # "Invert these because changed\nfrom PSD to QPD"
    # "Trap Y"
    # "Trap X"
    # "Convert to\npN"
    # "Convert to\nnm"
    # "Subtract\noffset"
    # "Normalize by\nsum"
    # "B sum"
    # "BX"
    # "BY"
    # "AX"
    # "AY"
    # "A sum"
    # "Close files when done saving"
    n116 = disable-structure shown="Disabled" {
      frame Disabled {
        n117 = property class="DAQmx Read"() -> ("AvailSampPerChan"=→"AvailSampPerChan 2":u32)  [unwired: 2 in, 2 out]
      }
      frame Enabled {
      }
    }
    n118 = local read "Averaging Number"() -> (w368:i32)
    n119 = local read "Averaging Number"() -> (w370:i32)
    "# Samples/channel" <- w370
    n120 = local read "Sampling Rate"() -> (w642:dbl)
    n121 = call-poly <vilib>:"DAQmx Read.vi"("task/channels in"=w345, "number of samples per channel"=w368, "timeout"=10.0) -> ("task out"=w344:refnum<k21>, "data"=w369:dbl[][], "error out"=w463:errorcluster)  [unwired: 10 in]
    n122 = Unbundle By Name(w463) -> ("status"=w582:bool)
    n123 = Divide(x=w642, y="Cal Averaging") -> (x/y=→"Cal Final Sampling Rate":dbl)
    n124 = Divide(x=w642, y=w370) -> (x/y=→"Final Sampling Rate" →"# Samples/channel/s":dbl)
    n125 = Index Array(array=w369, index (row)=4) -> (element=w459:dbl[])  [unwired: 1 in]
    n126 = disable-structure shown="Disabled" {
      frame Disabled {
        n127 = local read "Buffer size\n(Samples/channel)"() -> (w661:u32)
        n128 = property class="DAQmx Read"() -> ("AvailSampPerChan"=w662:u32)  [unwired: 2 in, 2 out]
        "AvailSampPerChan" <- w662
        n129 = Divide(x=w662, y=w661) -> (x/y=→"Buffer status":dbl)
      }
      frame Enabled {
      }
    }
    n130 = Index Array(array=w369, index (row)=5) -> (element=w458:dbl[])  [unwired: 1 in]
    n131 = Index Array(array=w369, index (row)=0) -> (element=w320:dbl[])  [unwired: 1 in]
    n132 = Index Array(array=w369, index (row)=3) -> (element=w319:dbl[])  [unwired: 1 in]
    n133 = Index Array(array=w369, index (row)=1) -> (element=w318:dbl[])  [unwired: 1 in]
    n134 = Index Array(array=w369, index (row)=2) -> (element=w321:dbl[])  [unwired: 1 in]
    n135 = Index Array(array=w369, index (row)=6) -> (element=w317:dbl[])  [unwired: 1 in]
    n136 = Index Array(array=w369, index (row)=7) -> (element=w316:dbl[])  [unwired: 1 in]
    n137 = case shown="True" w582 {
      frame False {
      }
      frame True {
        n138 = call <vilib>:"Beep.vi"() -> ()  [unwired: 12 in]
        "Buffer Overflow" <- TRUE
      }
    }
    n139 = Divide(x=w321, y=w317) -> (x/y=w315:dbl[])
    n140 = Divide(x=w320, y=w317) -> (x/y=w314:dbl[])
    n141 = Divide(x=w319, y=w316) -> (x/y=w313:dbl[])
    n142 = Divide(x=w318, y=w316) -> (x/y=w312:dbl[])
    n143 = local read "Cal values"() -> (w574:T2)
    n144 = Build Array(w315, w314, w313, w312) -> (w311:dbl[][])
    n145 = Unbundle(w574) -> ("AX alpha"=w562:dbl, "BX alpha"=w558:dbl, "AX kappa"=w554:dbl, "BX kappa"=w550:dbl, "AX offset"=w568:dbl, "BX offset"=w566:dbl, "AY alpha"=w565:dbl, "BY alpha"=w560:dbl, "AY kappa"=w556:dbl, "BY kappa"=w552:dbl, "AY offset"=w572:dbl, "BY offset"=w570:dbl)
    n146 = Multiply(x=w318, y=w462) -> (x*y=w460:dbl[])
    n147 = Multiply(x=w320, y=w462) -> (x*y=w461:dbl[])
    n148 = local write "AX alpha"(w562) -> ()
    n149 = local write "BY offset"(w570) -> ()
    n150 = Build Array(w461, w321, w460, w319, w317, w316, w459, w458) -> (w394:dbl[][])
    n151 = local write "BX alpha"(w558) -> ()
    n152 = case shown="True" "Reset data stream" {
      selector: "Reset data stream" -> [_ w809]
      tunnel: w344 -> [w801 w807]
      tunnel: [w801 w805] -> w534
      tunnel: w463 -> [w800 w804]
      tunnel: [w800 w802] -> _
      frame False {
      }
      frame True {
        n153 = Not(x=w809) -> (.not. x?=w808:bool)
        n154 = call <vilib>:"DAQmx Stop Task.vi"("task/channels in"=w807, "error in"=w804) -> ("task out"=w806:refnum<k21>, "error out"=w803:errorcluster)  [unwired: 12 in]
        n155 = local write "Reset data stream"(w808) -> ()
        n156 = local write "Buffer Overflow"(w808) -> ()
        n157 = call <vilib>:"DAQmx Start Task.vi"("task/channels in"=w806, "error in"=w803) -> ("task out"=w805:refnum<k21>, "error out"=w802:errorcluster)  [unwired: 12 in]
      }
    }
    n158 = call-poly <vilib>:"Mean.vi"("X"=w458) -> ("mean"=w588:dbl)  [unwired: 1 out]
    n159 = local write "AY offset"(w572) -> ()
    n160 = call-poly <vilib>:"Mean.vi"("X"=w459) -> ("mean"=w589:dbl)  [unwired: 1 out]
    n161 = call-poly <vilib>:"Mean.vi"("X"=w321) -> ("mean"=w595:dbl)  [unwired: 1 out]
    n162 = call-poly <vilib>:"Mean.vi"("X"=w319) -> ("mean"=w593:dbl)  [unwired: 1 out]
    n163 = call-poly <vilib>:"Mean.vi"("X"=w317) -> ("mean"=w592:dbl)  [unwired: 1 out]
    n164 = call-poly <vilib>:"Mean.vi"("X"=w316) -> ("mean"=w591:dbl)  [unwired: 1 out]
    n165 = local read "Averaging Number"() -> (w367:i32)
    n166 = local write "BY kappa"(w552) -> ()
    n167 = local write "AX kappa"(w554) -> ()
    n168 = call-poly <vilib>:"Mean.vi"("X"=w460) -> ("mean"=w594:dbl)  [unwired: 1 out]
    n169 = local write "AY kappa"(w556) -> ()
    n170 = call-poly <vilib>:"Mean.vi"("X"=w461) -> ("mean"=w596:dbl)  [unwired: 1 out]
    n171 = local read "DAQ rate\n(Samples/s)"() -> (w373:dbl)
    n172 = Build Array(w589, w588) -> (w587:dbl[])
    n173 = local write "BX kappa"(w550) -> ()
    n174 = local write "BY alpha"(w560) -> ()
    n175 = local write "AX offset"(w568) -> ()
    n176 = local write "BX offset"(w566) -> ()
    n177 = local write "AY alpha"(w565) -> ()
    n178 = Build Array(w596, w595, w594, w593, w592, w591) -> (w585:dbl[])
    n179 = local read "Total raster time (s)"() -> (w341:dbl)
    n180 = Divide(x=w367, y=w373) -> (x/y=w337:dbl)
    "Data update period (s/set)" <- w337
    n181 = Reciprocal(x=w373) -> (1/x=w374:dbl)
    "Data period (s)" <- w374
    n182 = Divide(x=w341, y=w337) -> (x/y=w340:dbl)
    n183 = Divide(x="Cal time (s)", y=w337) -> (x/y=w336:dbl)
    n184 = Divide(x=w596, y=w592) -> (x/y=w626:dbl)
    n185 = Divide(x=w595, y=w592) -> (x/y=w332:dbl)
    n186 = Round Toward -Infinity(1:w340) -> (0:w339:dbl)
    n187 = Divide(x=w594, y=w591) -> (x/y=w633:dbl)
    n188 = Divide(x=w593, y=w591) -> (x/y=w334:dbl)
    n189 = Round Toward -Infinity(1:w336) -> (0:→"Cal sets to save":dbl)
    n190 = local write "N sets to be saved"(w339) -> ()
    n191 = Build Array("Force Feedback 1", "Force Feedback 2") -> (w297:bool[])
    n192 = Boolean Array To Number(Boolean array=w297) -> (number=w296:u32)
    n193 = Negate(x=w332) -> (-x=w331:dbl)
    n194 = Negate(x=w334) -> (-x=w333:dbl)
    n195 = Subtract(x=w626, y="AY offset") -> (x-y=w608:dbl)
    n196 = Subtract(x=w332, y="AX offset") -> (x-y=w609:dbl)
    n197 = Subtract(x=w633, y="BY offset") -> (x-y=w607:dbl)
    n198 = Subtract(x=w334, y="BX offset") -> (x-y=w610:dbl)
    n199 = Subtract(x=w633, y=w626) -> (x-y=w624:dbl)
    n200 = Subtract(x=w333, y=w331) -> (x-y=w625:dbl)
    n201 = feedback #4(0.0) -> (w533:dbl)
    n202 = Multiply(x="Downsamp\nfact", y=w374) -> (x*y=w309:dbl)
    n203 = Multiply(x=w608, y="AY alpha") -> (x*y=w542:dbl)
    n204 = Multiply(x=w609, y="AX alpha") -> (x*y=w540:dbl)
    n205 = Multiply(x=w610, y="BX alpha") -> (x*y=w541:dbl)
    n206 = Multiply(x=w607, y="BY alpha") -> (x*y=w543:dbl)
    n207 = Add(x=w337, y=w533) -> (x+y=w531:dbl)
    n208 = feedback-in #4(w531) -> ()
    n209 = Square(x=w542) -> (x^2=w618:dbl)
    n210 = Square(x=w540) -> (x^2=w619:dbl)
    n211 = Square(x=w543) -> (x^2=w620:dbl)
    n212 = Square(x=w541) -> (x^2=w621:dbl)
    n213 = Bundle(w624, w625) -> (w328:cluster{dbl, dbl})  [unwired: 1 in]
    n214 = case shown="True" "Set reading to\nsetpoint 1" {
      tunnel: w328 -> [_ w798]
      frame False {
      }
      frame True {
        n215 = property on="Setpoint voltage 1" class="Clust (strict)"("Val(Sgnl)"=w798) -> ()  [unwired: 2 in, 2 out]
        n216 = local read "Trap position (V)"() -> (w797:cluster{"X":dbl, "Y":dbl})
        n217 = local write "Set reading to\nsetpoint 1"(FALSE ("Set reading to\nsetpoint")) -> ()
        n218 = Unbundle(w797) -> ("X"=w796:dbl, "Y"=w795:dbl)
        n219 = Bundle("Y"=w795, "X"=w796) -> (w794:cluster{"Y":dbl, "X":dbl})  [unwired: 1 in]
        n220 = property on="Offset 1" class="Clust (strict)"("Val(Sgnl)"=w794) -> ()  [unwired: 2 in, 2 out]
      }
    }
    n221 = Reciprocal(x=w309) -> (1/x=→"Chart Freq (Hz)":dbl)
    n222 = To Time Stamp(1:w531) -> (0:w308:timestamp)
    n223 = Add(x=w618, y=w619) -> (x+y=w622:dbl)
    n224 = Add(x=w620, y=w621) -> (x+y=w632:dbl)
    n225 = Multiply(x=w540, y="AX kappa") -> (x*y=w536:dbl)
    n226 = Bundle("A y", "A x", "B y", "B x", "A sum", "B sum", "Trap x", "Trap y") -> (w522:T20)  [unwired: 1 in]
    n227 = Multiply(x=w541, y="BX kappa") -> (x*y=w537:dbl)
    n228 = Square Root(x=w622) -> (sqrt(x)=w636:dbl)
    n229 = Square Root(x=w632) -> (sqrt(x)=w635:dbl)
    n230 = Multiply(x=w542, y="AY kappa") -> (x*y=w538:dbl)
    n231 = Multiply(x=w543, y="BY kappa") -> (x*y=w539:dbl)
    n232 = Subtract(x=w588, y="Fixed Y") -> (x-y=w623:dbl)
    n233 = Subtract(x=w589, y="Fixed X") -> (x-y=w627:dbl)
    n234 = Cluster To Array(cluster=w522) -> (array=w521:string[])
    n235 = for {
      tunnel: w394 -> [w787] mode=indexing
      tunnel: w309 -> [w786]
      tunnel: "Downsamp\nfact" -> [w792]
      tunnel: [w790] -> w327 mode=indexing
      tunnel: w308 -> [w793]
      tunnel: w521 -> [w789] mode=indexing
      tunnel: w301 -> [w788]
      n236 = call "Downsample 1D array.vi"("Ave N"=w792, "Arrray In"=w787) -> ("Array Out"=w785:dbl[])  [unwired: 9 in]
      n237 = Bundle By Name("Y"=w785, "dt"=w786, "t0"=w793) -> (w791:waveform(dbl))  [unwired: 1 in]
      n238 = Set Waveform Attribute(5:w789, 6:w788, 7:w791) -> (3:w790:waveform(dbl))  [unwired: 1 in, 2 out]
    }
    "All signals" <- w327
    n239 = Square(x=w538) -> (x^2=w611:dbl)
    n240 = Square(x=w536) -> (x^2=w612:dbl)
    n241 = Square(x=w539) -> (x^2=w613:dbl)
    n242 = Square(x=w537) -> (x^2=w614:dbl)
    n243 = Add(x=w611, y=w612) -> (x+y=w615:dbl)
    n244 = Add(x=w613, y=w614) -> (x+y=w616:dbl)
    n245 = Multiply(x=w623, y="Conv Y (nm/V)") -> (x*y=w545:dbl)
    n246 = Multiply(x=w627, y="Conv X (nm/V)") -> (x*y=w546:dbl)
    n247 = feedback #5() -> (w583:cluster{"B_Y":dbl, "B_X":dbl})  [unwired: 1 in]
    n248 = case shown="2" w296 {
      tunnel: [w1139 w1156 w1166] -> w361
      tunnel: [w1138 w1155 w1167] -> w359
      tunnel: w328 -> [_ w1154 w1169]
      tunnel: [cluster{"B_Y":dbl, "B_X":dbl} {"B_Y"=0.0, "B_X"=0.0} ("Sum error past") w1146 w1164] -> w584
      tunnel: w583 -> [_ w1153 w1165]
      tunnel: w639 -> [w1139 w1149 w1157]
      tunnel: w644 -> [w1138 w1148 w1168]
      frame 0, Default {
        # "Force feedback"
      }
      frame 1 {
        n249 = local write "Force Feedback 2"(FALSE) -> ()
        n250 = call "ForceFeedback2.vi"("PSD/Mirror Voltages"=w1154, "Sum error"=w1153, "task/channels in"=w1149, "error in"=w1148, "Desired voltage"="Setpoint voltage 1", "Feedback const"="Feedback const", "offset"="Offset 1") -> ("task out"=w1156:refnum<k21>, "Sum error past"=w1146:cluster{"B_Y":dbl, "B_X":dbl}, "Output Voltage"=→"Feedback Output \nVoltage 2":cluster{dbl, dbl}, "error out"=w1155:errorcluster)  [unwired: 8 in, 1 out]
        n251 = local read "Pulling direction"() -> (w1145:bool)
        n252 = Unbundle(w1146) -> ("B_Y"=w1143:dbl, "B_X"=w1142:dbl)
        n253 = Select(t=w1143, s=w1145, f=w1142) -> (s? t:f=→"Sum error":dbl)
      }
      frame 2 {
        n254 = local write "Force Feedback 1"(FALSE) -> ()
        n255 = local read "Feedback const"() -> (w1158:T6)
        n256 = call "ForceFeedback2.vi"("PSD/Mirror Voltages"=w1169, "Sum error"=w1165, "task/channels in"=w1157, "error in"=w1168, "Desired voltage"="Setpoint voltage 2", "Feedback const"=w1158, "offset"="Offset 2") -> ("task out"=w1166:refnum<k21>, "Sum error past"=w1164:cluster{"B_Y":dbl, "B_X":dbl}, "Output Voltage"=w1159:cluster{dbl, dbl}, "error out"=w1167:errorcluster)  [unwired: 8 in, 1 out]
        n257 = local read "Pulling direction"() -> (w1160:bool)
        n258 = property on="Feedback Output \nVoltage 2" class="Clust (strict)"("Val(Sgnl)"=w1159) -> ()  [unwired: 2 in, 2 out]
        n259 = Unbundle(w1164) -> ("B_Y"=w1163:dbl, "B_X"=w1162:dbl)
        n260 = Select(t=w1163, s=w1160, f=w1162) -> (s? t:f=w1161:dbl)
        n261 = local write "Sum error"(w1161) -> ()
      }
    }
    n262 = feedback-in #5(w584) -> ()
    n263 = Square Root(x=w615) -> (sqrt(x)=w544:dbl)
    n264 = Square Root(x=w616) -> (sqrt(x)=w637:dbl)
    n265 = Add(x=w544, y=w637) -> (x+y=w617:dbl)
    n266 = case shown="True" "Set reading to\nsetpoint 2" {
      tunnel: w328 -> [_ w656]
      frame False {
      }
      frame True {
        n267 = local read "Trap position (V)"() -> (w659:cluster{"X":dbl, "Y":dbl})
        n268 = property on="Setpoint voltage 2" class="Clust (strict)"("Val(Sgnl)"=w656) -> ()  [unwired: 2 in, 2 out]
        n269 = local write "Set reading to\nsetpoint 2"(FALSE) -> ()
        n270 = Unbundle(w659) -> ("X"=w658:dbl, "Y"=w657:dbl)
        n271 = Bundle("Y"=w657, "X"=w658) -> (w655:cluster{"Y":dbl, "X":dbl})  [unwired: 1 in]
        n272 = property on="Offset 2" class="Clust (strict)"("Val(Sgnl)"=w655) -> ()  [unwired: 2 in, 2 out]
      }
    }
    n273 = Build Array(w626, w332, w633, w334, w592, w591, w544, w637, w636, w635, w546, w545) -> ()  [unwired: 1 out]
    n274 = Divide(x=w617, y=2.0) -> (x/y=w581:dbl)
    n275 = Bundle("AX/Asum", "AY/Asum", "BX/Bsum", "BY/Bsum") -> (w303:cluster{string, string, string, string})  [unwired: 1 in]
    n276 = Index Array(array=w327, index=6) -> (element=w399:waveform(dbl))
    n277 = Index Array(array=w327, index=7) -> (element=w401:waveform(dbl))
    n278 = Cluster To Array(cluster=w303) -> (array=w302:string[])
    n279 = for {
      tunnel: w311 -> [w654] mode=indexing
      tunnel: "Downsamp\nfact" -> [w653]
      tunnel: w309 -> [w652]
      tunnel: w308 -> [w650]
      tunnel: w302 -> [w648] mode=indexing
      tunnel: w301 -> [w647]
      tunnel: [w646] -> w300 mode=indexing
      n280 = call "Downsample 1D array.vi"("Ave N"=w653, "Arrray In"=w654) -> ("Array Out"=w651:dbl[])  [unwired: 9 in]
      n281 = Bundle By Name("Y"=w651, "dt"=w652, "t0"=w650) -> (w649:waveform(dbl))  [unwired: 1 in]
      n282 = Set Waveform Attribute(5:w648, 6:w647, 7:w649) -> (3:w646:waveform(dbl))  [unwired: 1 in, 2 out]
    }
    "All signals 2" <- w300
    n283 = local read "Fixed X"() -> (w448:dbl)
    n284 = local read "Fixed Y"() -> (w450:dbl)
    n285 = Unbundle By Name(w399) -> ("Y"=w452:dbl[])
    n286 = Unbundle By Name(w401) -> ("Y"=w451:dbl[])
    n287 = Index Array(array=w327, index=0) -> (element=w406:waveform(dbl))
    n288 = Index Array(array=w327, index=1) -> (element=w518:waveform(dbl))
    n289 = Index Array(array=w327, index=4) -> (element=w512:waveform(dbl))
    n290 = Subtract(x=w452, y=w448) -> (x-y=w449:dbl[])
    n291 = Subtract(x=w451, y=w450) -> (x-y=w446:dbl[])
    n292 = Unbundle By Name(w406) -> ("Y"=w510:dbl[])
    n293 = Unbundle By Name(w518) -> ("Y"=w509:dbl[])
    n294 = Unbundle By Name(w512) -> ("Y"=w508:dbl[])
    n295 = Index Array(array=w327, index=5) -> (element=w511:waveform(dbl))
    n296 = local read "Conv X (nm/V)"() -> (w447:dbl)
    n297 = local read "Conv Y (nm/V)"() -> (w445:dbl)
    n298 = Index Array(array=w327, index=2) -> (element=w322:waveform(dbl))
    n299 = Index Array(array=w327, index=3) -> (element=w515:waveform(dbl))
    n300 = Set Waveform Attribute(5:"T2 X", 6:w397, 7:w399) -> (3:w398:waveform(dbl))  [unwired: 1 in, 2 out]
    n301 = Set Waveform Attribute(5:"T2 Y", 6:w397, 7:w401) -> (3:w400:waveform(dbl))  [unwired: 1 in, 2 out]
    n302 = Unbundle By Name(w511) -> ("Y"=w505:dbl[])
    n303 = Unbundle By Name(w322) -> ("Y"=w507:dbl[])
    n304 = Unbundle By Name(w515) -> ("Y"=w506:dbl[])
    n305 = Divide(x=w510, y=w508) -> (x/y=w326:dbl[])
    n306 = Divide(x=w509, y=w508) -> (x/y=w325:dbl[])
    n307 = local read "AY offset"() -> (w496:dbl)
    n308 = local read "AX offset"() -> (w494:dbl)
    n309 = Multiply(x=w449, y=w447) -> (x*y=w391:dbl[])
    n310 = Multiply(x=w446, y=w445) -> (x*y=w393:dbl[])
    n311 = Divide(x=w506, y=w505) -> (x/y=w323:dbl[])
    n312 = Subtract(x=w325, y=w494) -> (x-y=w497:dbl[])
    n313 = local read "BX offset"() -> (w504:dbl)
    n314 = Subtract(x=w326, y=w496) -> (x-y=w498:dbl[])
    n315 = Divide(x=w507, y=w505) -> (x/y=w324:dbl[])
    n316 = local read "AY alpha"() -> (w495:dbl)
    n317 = local read "AX alpha"() -> (w493:dbl)
    n318 = call-poly <vilib>:"Mean.vi"("X"=w393) -> ("mean"=w428:dbl)  [unwired: 1 out]
    "Mean Trp Pos Y 2 (nm)" <- w428
    n319 = Subtract(x=w324, y=w326) -> (x-y=w418:dbl[])
    n320 = Subtract(x=w323, y=w325) -> (x-y=w417:dbl[])
    n321 = local read "BY offset"() -> (w501:dbl)
    n322 = Subtract(x=w391, y="Offset X (nm)") -> (x-y=w390:dbl[])
    n323 = Subtract(x=w393, y="Offset Y (nm)") -> (x-y=w392:dbl[])
    n324 = Subtract(x=w324, y=w501) -> (x-y=w503:dbl[])
    n325 = Subtract(x=w323, y=w504) -> (x-y=w502:dbl[])
    n326 = Subtract(x=w428, y=w393) -> (x-y=w427:dbl[])
    n327 = call-poly <vilib>:"Mean.vi"("X"=w391) -> ("mean"=w432:dbl)  [unwired: 1 out]
    "Mean Trap Pos X 2 (nm)" <- w432
    n328 = Build Array(w418, w417) -> (w415:dbl[][])
    n329 = Index Array(array=w415, index (row)=0) -> (element=w413:dbl[])  [unwired: 1 in]
    n330 = Index Array(array=w415, index (row)=1) -> (element=w412:dbl[])  [unwired: 1 in]
    n331 = call-poly <vilib>:"Mean.vi"("X"=w413) -> ("mean"=w411:dbl)  [unwired: 1 out]
    n332 = call-poly <vilib>:"Mean.vi"("X"=w412) -> ("mean"=w410:dbl)  [unwired: 1 out]
    n333 = Bundle("mean"=w411, "mean"=w410) -> ()  [unwired: 1 in, 1 out]
    n334 = local read "BX alpha"() -> (w499:dbl)
    n335 = Multiply(x=w498, y=w495) -> (x*y=w486:dbl[])
    n336 = Multiply(x=w497, y=w493) -> (x*y=w485:dbl[])
    n337 = Square(x=w427) -> (x^2=w426:dbl[])
    n338 = Subtract(x=w432, y=w391) -> (x-y=w431:dbl[])
    n339 = Bundle By Name(cluster=w400, "Y"=w392) -> (w443:waveform(dbl))
    n340 = Bundle By Name(cluster=w398, "Y"=w390) -> (w444:waveform(dbl))
    n341 = local read "BY alpha"() -> (w500:dbl)
    n342 = local read "Raster scanning..."() -> (w343:bool)
    n343 = local read "Saving"() -> (w547:bool)
    n344 = local read "Tether"() -> (w548:bool)
    n345 = Square(x=w431) -> (x^2=w430:dbl[])
    n346 = call-poly <vilib>:"Mean.vi"("X"=w426) -> ("mean"=w425:dbl)  [unwired: 1 out]
    n347 = Square(x=w486) -> (x^2=w492:dbl[])
    n348 = Multiply(x=w503, y=w500) -> (x*y=w484:dbl[])
    n349 = Square(x=w485) -> (x^2=w491:dbl[])
    n350 = Multiply(x=w502, y=w499) -> (x*y=w483:dbl[])
    n351 = Less?(x=w581, y="Tether break\nforce (pN)") -> (x < y?=w579:bool)
    n352 = call-poly <vilib>:"Mean.vi"("X"=w430) -> ("mean"=w429:dbl)  [unwired: 1 out]
    n353 = Build Array(w444, w443) -> (w362:waveform(dbl)[])
    "Trap sep" <- w362
    n354 = Square Root(x=w425) -> (sqrt(x)=w424:dbl)
    n355 = Square(x=w484) -> (x^2=w490:dbl[])
    n356 = Square(x=w483) -> (x^2=w489:dbl[])
    n357 = Add(x=w492, y=w491) -> (x+y=w488:dbl[])
    n358 = Square Root(x=w429) -> (sqrt(x)=w422:dbl)
    n359 = Compound Arithmetic op=AND(w547, w548, w579) -> (w578:bool)
    n360 = Multiply(x=w424, y=10) -> (x*y=→"T2 Y RMS (A)":dbl)
    n361 = Square Root(x=w488) -> (sqrt(x)=w386:dbl[])
    n362 = Add(x=w490, y=w489) -> (x+y=w487:dbl[])
    n363 = Set Waveform Attribute(5:"T2", 6:"NI_ChannelName" ("name"), 7:w406) -> (3:w405:waveform(dbl))  [unwired: 1 in, 2 out]
    n364 = Set Waveform Attribute(5:"T1", 6:"NI_ChannelName" ("name"), 7:w322) -> (3:w403:waveform(dbl))  [unwired: 1 in, 2 out]
    n365 = case shown="True" w578 {
      selector: w578 -> [_ w816]
      tunnel: w343 -> [w810 w812]
      tunnel: [w810 w812] -> w342
      frame False {
      }
      frame True {
        n366 = call <vilib>:"Beep.vi"() -> ()  [unwired: 12 in]
        n367 = Not(x=w816) -> (.not. x?=w811:bool)
        n368 = And(x=w812, y="Fish After TA?") -> (x .and. y?=w814:bool)
        n369 = local write "Force Feedback 1"(w811) -> ()
        n370 = local write "Tether"(w811) -> ()
        n371 = case shown="True" w814 {
          selector: w814 -> [_ w817]
          frame False {
          }
          frame True {
            n372 = property on="Fish" class="Bool (strict)"("Val(Sgnl)"=w817) -> ()  [unwired: 2 in, 2 out]
          }
        }
        n373 = local write "Force Feedback 2"(w811) -> ()
        n374 = property on="Stop saving" class="Bool (strict)"("Val(Sgnl)"="TA Cancel Save?") -> ()  [unwired: 2 in, 2 out]
      }
    }
    n375 = Square Root(x=w487) -> (sqrt(x)=w385:dbl[])
    n376 = Multiply(x=w422, y=10) -> (x*y=→"T2 X RMS (A)":dbl)
    n377 = Bundle By Name(cluster=w405, "Y"=w386) -> (w409:waveform(dbl))
    n378 = Bundle By Name(cluster=w403, "Y"=w385) -> (w465:waveform(dbl))
    n379 = Add(x=w386, y=w385) -> (x+y=w384:dbl[])
    n380 = case shown="True" "Remove offsets" {
      selector: "Remove offsets" -> [_ w783]
      frame False {
      }
      frame True {
        n381 = local read "Mean Trp Pos Y 2 (nm)"() -> (w781:dbl)
        n382 = Not(x=w783) -> (.not. x?=w784:bool)
        n383 = local read "Mean Trap Pos X 2 (nm)"() -> (w782:dbl)
        n384 = local write "Remove offsets"(w784) -> ()
        n385 = local write "Offset Y (nm)"(w781) -> ()
        n386 = local write "Offset X (nm)"(w782) -> ()
      }
    }
    n387 = Build Array(w409, w465) -> (→"Bead sep":waveform(dbl)[])
    n388 = local read "AY kappa"() -> (w482:dbl)
    n389 = local read "AX kappa"() -> (w481:dbl)
    n390 = Divide(x=w384, y=2) -> (x/y=w382:dbl[])
    n391 = local read "BX kappa"() -> (w479:dbl)
    n392 = local read "BY kappa"() -> (w480:dbl)
    n393 = call-poly <vilib>:"Mean.vi"("X"=w382) -> ("mean"=w381:dbl)  [unwired: 1 out]
    "Mean Bead Sep\n(nm)" <- w381
    n394 = local read "Calibrating"() -> (w638:bool)
    n395 = Multiply(x=w486, y=w482) -> (x*y=w475:dbl[])
    n396 = Multiply(x=w485, y=w481) -> (x*y=w476:dbl[])
    n397 = Square(x=w475) -> (x^2=w474:dbl[])
    n398 = Square(x=w476) -> (x^2=w473:dbl[])
    n399 = Subtract(x=w382, y=w381) -> (x-y=w380:dbl[])
    n400 = Multiply(x=w484, y=w480) -> (x*y=w477:dbl[])
    n401 = Multiply(x=w483, y=w479) -> (x*y=w478:dbl[])
    n402 = Or(x=w342, y="Raster scan") -> (x .or. y?=w357:bool)
    n403 = Add(x=w474, y=w473) -> (x+y=w470:dbl[])
    n404 = Square(x=w380) -> (x^2=w379:dbl[])
    n405 = Square Root(x=w470) -> (sqrt(x)=w442:dbl[])
    n406 = Square(x=w477) -> (x^2=w472:dbl[])
    n407 = Square(x=w478) -> (x^2=w471:dbl[])
    n408 = call-poly <vilib>:"Mean.vi"("X"=w379) -> ("mean"=w378:dbl)  [unwired: 1 out]
    n409 = Add(x=w472, y=w471) -> (x+y=w469:dbl[])
    n410 = Bundle By Name(cluster=w405, "Y"=w442) -> (w468:waveform(dbl))
    n411 = local read "Saving"() -> (w577:bool)
    n412 = Or(x=w638, y=w577) -> ()  [unwired: 1 out]
    n413 = Square Root(x=w378) -> (sqrt(x)=w377:dbl)
    n414 = Square Root(x=w469) -> (sqrt(x)=w441:dbl[])
    n415 = Multiply(x=10, y=w377) -> (x*y=→"Bead Sep Noise\n(A)":dbl)
    n416 = Bundle By Name(cluster=w403, "Y"=w441) -> (w467:waveform(dbl))
    n417 = Add(x=w442, y=w441) -> (x+y=w440:dbl[])
    n418 = Build Array(w468, w467) -> (→"Force (pN)":waveform(dbl)[])
    n419 = Divide(x=w440, y=2) -> (x/y=w437:dbl[])
    n420 = call-poly <vilib>:"Mean.vi"("X"=w437) -> ("mean"=w438:dbl)  [unwired: 1 out]
    "Mean force (pN)" <- w438
    n421 = Subtract(x=w438, y=w437) -> (x-y=w436:dbl[])
    n422 = Square(x=w436) -> (x^2=w435:dbl[])
    n423 = call-poly <vilib>:"Mean.vi"("X"=w435) -> ("mean"=w434:dbl)  [unwired: 1 out]
    n424 = flat-sequence {
      tunnel: w638 -> [w860]
      tunnel: w577 -> [_]
      tunnel: w638 -> [_]
      tunnel: w577 -> [_]
      tunnel: w394 -> [w847]
      tunnel: [w847] -> w598
      tunnel: w463 -> [w846]
      tunnel: [w846] -> w597
      tunnel: w585 -> [w845]
      tunnel: [w845] -> w590
      tunnel: w587 -> [w844]
      tunnel: [w844] -> w586
      tunnel: [w841] -> w576
      tunnel: [w838] -> w575
      tunnel: [w835] -> w457
      tunnel: [w834] -> w456
      tunnel: [w831] -> w455
      tunnel: w364 -> [w828]
      tunnel: ["Save Data"] -> w363
      tunnel: [w821] -> w330
      tunnel: w598 -> [w1036]
      tunnel: w597 -> [w1035]
      tunnel: w590 -> [_]
      tunnel: w586 -> [_]
      tunnel: w576 -> [w1034]
      tunnel: w575 -> [w1033]
      tunnel: w457 -> [w1032]
      tunnel: w456 -> [w1031]
      tunnel: w455 -> [w1030]
      tunnel: w363 -> [w1029]
      tunnel: w362 -> [w1028]
      tunnel: w330 -> [w1026]
      frame #0 {
        w827 = 0.0
        # "1: old trap\n0: fleezers"
        # "Create files if saving data"
        n425 = local read "Save N sets"() -> (w830:bool)
        n426 = local read "Fixed X"() -> (w826:dbl)
        n427 = local read "Trap position (V)"() -> (w855:cluster{"X":dbl, "Y":dbl})
        n428 = local read "Fixed Y"() -> (w825:dbl)
        n429 = local read "Sampling Rate"() -> (w858:dbl)
        n430 = Or(x=w830, y="Save Data") -> (x .or. y?=w829:bool)
        n431 = Build Array(w829, "Save cal", w828) -> (w849:bool[])
        n432 = Compound Arithmetic op=OR("Save Data", "Save cal", w828) -> (w851:bool)
        n433 = Boolean Array To Number(Boolean array=w849) -> (number=w848:u32)
        n434 = Unbundle(w855) -> ("X"=w824:dbl, "Y"=w823:dbl)
        n435 = Build Array(w824, w823, w826, w825, w827, w827) -> (w854:dbl[])
        n436 = feedback #6(refnum<k0> refnum) -> (w820:refnum<file>)
        n437 = feedback #7(0) -> (w852:i32)
        n438 = feedback #8(refnum<k0> refnum) -> (w842:refnum<file>)
        n439 = feedback #9() -> (w836:dbl)  [unwired: 1 in]
        n440 = feedback #10(FALSE) -> (w832:bool)
        n441 = feedback #11(refnum<k0> refnum) -> (w839:refnum<file>)
        n442 = case shown="True" w851 {
          tunnel: w860 -> [_ _]
          tunnel: 9 -> [_ w906]
          tunnel: w858 -> [_ w905]
          tunnel: 6 -> [_ w904]
          tunnel: 5 -> [_ w903]
          tunnel: w854 -> [_ w902]
          tunnel: [w866 1] -> w835
          tunnel: w852 -> [w867 _]
          tunnel: w848 -> [_ w878]
          tunnel: [w865 w877] -> w841
          tunnel: w842 -> [w865 _]
          tunnel: [w864 w876] -> w838
          tunnel: w839 -> [w864 _]
          tunnel: 1.0 -> [_ w875]
          tunnel: [w863 w874] -> w834
          tunnel: w836 -> [w863 _]
          tunnel: [w862 w873] -> w831
          tunnel: w832 -> [w862 _]
          tunnel: [w861 w868] -> w821
          tunnel: w820 -> [w861 _]
          frame False {
            n443 = Increment(x=w867) -> (x+1=w866:i32)
          }
          frame True {
            w879 = FALSE ("Save Data")
            w884 = FALSE
            w885 = T19."big-endian, network order" ("byte order (0:big-endian, network order)")
            n444 = local write "Save cal"(w879) -> ()
            n445 = local write "Save Data"(w879) -> ()
            n446 = case shown="4" w878 {
              tunnel: w906 -> [w975 w993 w1024]
              tunnel: w905 -> [w954 w992 w1000]
              tunnel: w904 -> [w974 w990 w1020]
              tunnel: w903 -> [w973 w989 w1019]
              tunnel: w902 -> [w972 w986 w1016]
              tunnel: [w971 w985 w1005] -> w899
              tunnel: [w952 w976 w995] -> w873
              tunnel: ["Averaging Number" 200 w1003] -> _
              tunnel: w875 -> [w959 w978 w1002]
              tunnel: [w955 w977 w996] -> w874
              tunnel: [w952 w976 w994] -> w870
              frame 1, Default {
                w952 = TRUE
                w960 = 0.0
                # "Save N number/length of data. e.g. N =200 \nwill give only 200 long data points"
                # "Time trace"
                n447 = Boolean To (0,1)(Boolean=w952) -> (0, 1=w965:i16)
                n448 = local read "Averaging Number"() -> (w970:i32)
                n449 = Increment(x=w965) -> (x+1=w964:i16)
                n450 = Divide(x=w954, y=w970) -> (x/y=w969:dbl)
                n451 = To Double Precision Float(number=w964) -> (double precision float=w963:dbl)
                n452 = Reciprocal(x=w969) -> (1/x=w968:dbl)
                n453 = Reciprocal(x=w954) -> (1/x=w953:dbl)
                n454 = Build Array(w975, w953, w968, w974, w973, 0 ("f")) -> (w967:dbl[])
                n455 = Select(t="N sets", s="Save N sets", f=2147483647) -> (s? t:f=w955:i32)
                n456 = Build Array(w963, w959, w960, w960, w960) -> (w966:dbl[])
                n457 = Build Array (concatenate)(w967, w972, w966) -> (w971:dbl[])
              }
              frame 2 {
                w976 = FALSE
                w981 = 0.0
                # "Calibration file"
                n458 = Reciprocal(x=w992) -> (1/x=w991:dbl)
                n459 = Boolean To (0,1)(Boolean=w976) -> (0, 1=w984:i16)
                n460 = To Double Precision Float(number=w984) -> (double precision float=w983:dbl)
                n461 = Build Array(w993, w991, w991, w990, w989, 1) -> (w987:dbl[])
                n462 = Build Array(w983, w978, w981, w981, w981) -> (w982:dbl[])
                n463 = Build Array (concatenate)(w987, w986, w982) -> (w985:dbl[])
                n464 = local read "Cal sets to save"() -> (w977:i32)
                "Calibrating" <- TRUE ("Calibrating")
              }
              frame 4 {
                w1012 = 0.0
                w995 = TRUE
                # "Not using ncycles"
                # "FX curve"
                n465 = local read "Averaging Number"() -> (w1023:i32)
                n466 = Boolean To (0,1)(Boolean=w995) -> (0, 1=w1015:i16)
                n467 = Increment(x=w1015) -> (x+1=w1014:i16)
                n468 = local write "Raster scan"(FALSE ("Raster scan")) -> ()
                n469 = To Double Precision Float(number=w1014) -> (double precision float=w1013:dbl)
                n470 = Divide(x=w1000, y=w1023) -> (x/y=w1022:dbl)
                n471 = Reciprocal(x=w1022) -> (1/x=w1021:dbl)
                n472 = Build Array(w1013, w1002, w1012, w1012, w1012) -> (w1011:dbl[])
                n473 = Reciprocal(x=w1000) -> (1/x=w999:dbl)
                n474 = Build Array(w1024, w999, w1021, w1020, w1019, 2) -> (w1017:dbl[])
                n475 = local read "Scan range (V)"() -> (w997:dbl)
                n476 = local read "Pulling direction"() -> (w1009:bool)
                n477 = local read "N sets to be saved"() -> (w996:dbl)
                n478 = local read "Scan steps (mirror)"() -> (w998:u64)
                n479 = Not(x=w995) -> (.not. x?=w994:bool)
                n480 = local read "# scans"() -> (w1007:i32)
                n481 = Not(x=w1009) -> (.not. x?=w1008:bool)
                n482 = local read "Averaging Number"() -> (w1003:i32)
                n483 = Boolean To (0,1)(Boolean=w1008) -> (0, 1=w1010:i16)
                n484 = Build Array(w1010, w997, w998, 0, w1007) -> (w1006:dbl[])
                n485 = Build Array (concatenate)(w1017, w1016, w1011, w1006) -> (w1005:dbl[])
              }
            }
            n486 = call "CreateSaveFile.vi"("Index In"="Save file index", "Ext"=".dat", "Insert"="", "Directory"="Path") -> ("Index Out"=w872:i32, "Path Out"=w869:path)  [unwired: 6 in]
            "Current file name" <- w869
            n487 = case shown="True" w870 {
              tunnel: w869 -> [_ w912]
              tunnel: [refnum<k0> refnum w908] -> w868
              frame False {
              }
              frame True {
                # "SY 190201 \nAdding functionality to get time points of start and stop moves. \nWehn timetrace save data starts save time point"
                n488 = Path To String(path=w912) -> (string=w916:string)
                n489 = Get Date/Time In Seconds() -> (seconds since 1Jan1904=w926:timestamp)
                n490 = String Length(string=w916) -> (length=w913:i32)
                n491 = Subtract(x=w913, y=4) -> (x-y=w915:i32)
                n492 = Format Date/Time String(time format string (%c)="%H:%M:%S%3u", seconds (now)=w926, UTC format=TRUE) -> (date/time string=w909:string)
                n493 = String Subset(string=w916, length (rest)=w915) -> (substring=w917:string)  [unwired: 1 in]
                n494 = Concatenate Strings(w917, "_stagetime.txt" ("string")) -> (w919:string)
                n495 = String To Path(string=w919) -> (path=w920:path)
                n496 = Open/Create/Replace File(file path (use dialog)=w920, operation (0:open)=T18."create", access (0:read/write)=enum16{"read/write", "read-only", "write-only"}."write-only") -> (refnum out=w924:refnum<file>, error out=w923:errorcluster)  [unwired: 3 in, 1 out]
                n497 = Deny Access(4:w923, 7:w924) -> (3:w925:refnum<file>)  [unwired: 1 in, 1 out]
                n498 = Concatenate Strings(w909, "\r\n") -> (w910:string)
                n499 = Write to Text File(file (use dialog)=w925, text=w910) -> (refnum out=w908:refnum<file>)  [unwired: 2 in, 2 out]
                n500 = local write "Move time"(w909) -> ()
              }
            }
            n501 = Open/Create/Replace File(file path (use dialog)=w869, operation (0:open)=T18."create", access (0:read/write)=enum16{"read/write", "read-only", "write-only"}."write-only") -> (refnum out=w892:refnum<file>, error out=w893:errorcluster)  [unwired: 3 in, 1 out]
            n502 = local write "Save file index"(w872) -> ()
            n503 = Array Size(array=w899) -> (size(s)=w901:i32)
            n504 = case shown="True" w873 {
              tunnel: w869 -> [_ w951]
              tunnel: [refnum<k0> refnum w930] -> w876
              frame False {
              }
              frame True {
                w937 = 0.0
                n505 = Path To String(path=w951) -> (string=w947:string)
                n506 = Build Array(w937, w937, w937, w937, w937, w937, w937, w937) -> (w934:dbl[])
                n507 = String Length(string=w947) -> (length=w950:i32)
                n508 = Array Size(array=w934) -> (size(s)=w936:i32)
                n509 = Subtract(x=w950, y=4) -> (x-y=w948:i32)
                n510 = To Double Precision Float(number=w936) -> (double precision float=w935:dbl)
                n511 = String Subset(string=w947, length (rest)=w948) -> (substring=w946:string)  [unwired: 1 in]
                n512 = Build Array (concatenate)(w935, w934) -> (w933:dbl[])
                n513 = Concatenate Strings(w946, "_pos.dat" ("string")) -> (w944:string)
                n514 = String To Path(string=w944) -> (path=w943:path)
                n515 = Open/Create/Replace File(file path (use dialog)=w943, operation (0:open)=T18."create", access (0:read/write)=enum16{"read/write", "read-only", "write-only"}."write-only") -> (refnum out=w939:refnum<file>, error out=w940:errorcluster)  [unwired: 3 in, 1 out]
                n516 = Deny Access(4:w940, 7:w939) -> (3:w938:refnum<file>)  [unwired: 1 in, 1 out]
                n517 = Write to Binary File(file (use dialog)=w938, data=w933, 5:FALSE ("prepend array or string size? (T)"), 9:T19."big-endian, network order" ("byte order (0:big-endian, network order)")) -> (refnum out=w930:refnum<file>)  [unwired: 2 in, 2 out]
              }
            }
            n518 = Deny Access(4:w893, 7:w892) -> (0:w883:errorcluster, 3:w891:refnum<file>)  [unwired: 1 in]
            n519 = String Length(string="Comment") -> (length=w898:i32)
            n520 = To Double Precision Float(number=w901) -> (double precision float=w900:dbl)
            n521 = To Double Precision Float(number=w898) -> (double precision float=w897:dbl)
            n522 = Build Array (concatenate)(w900, w899, w897) -> (w888:dbl[])
            n523 = Write to Binary File(file (use dialog)=w891, data=w888, error in=w883, 5:w884, 9:w885) -> (refnum out=w887:refnum<file>, error out=w882:errorcluster)  [unwired: 1 in, 1 out]
            n524 = Write to Binary File(file (use dialog)=w887, data="Comment", error in=w882, 5:w884, 9:w885) -> (refnum out=w877:refnum<file>)  [unwired: 1 in, 2 out]
            "Saving" <- TRUE
          }
        }
        n525 = feedback-in #6(w821) -> ()
        n526 = feedback-in #7(w835) -> ()
        n527 = feedback-in #8(w841) -> ()
        n528 = feedback-in #9(w834) -> ()
        n529 = feedback-in #10(w831) -> ()
        n530 = feedback-in #11(w838) -> ()
      }
      frame #1 {
        n531 = local read "Raster scan"() -> (w1025:bool)
        n532 = local read "Saving"() -> (w1027:bool)
        n533 = case shown="True" w1027 {
          tunnel: w1036 -> [_ w1058]
          tunnel: w1035 -> [_ w1057]
          tunnel: w1034 -> [_ w1056]
          tunnel: w1033 -> [_ w1055]
          tunnel: w1032 -> [_ w1046]
          tunnel: w1031 -> [_ w1047]
          tunnel: w1030 -> [_ w1050]
          tunnel: w1029 -> [_ w1042]
          tunnel: w1028 -> [_ w1041]
          tunnel: w1026 -> [_ w1039]
          tunnel: w1025 -> [_ w1037]
          frame False {
            (unwired) FALSE ("Calibrating")
          }
          frame True {
            n534 = local read "Calibrating"() -> (w1038:bool)
            n535 = local read "Stop"() -> (w1053:bool)
            n536 = Less Or Equal?(x=w1046, y=w1047) -> (x <= y?=w1054:bool)
            n537 = Divide(x=w1046, y=w1047) -> (x/y=w1045:dbl)
            n538 = Or(x=w1053, y="Stop saving") -> (x .or. y?=w1040:bool)
            n539 = Multiply(x=100.0, y=w1045) -> (x*y=w1044:dbl)
            n540 = Not(x=w1040) -> (.not. x?=w1052:bool)
            n541 = And(x=w1054, y=w1052) -> (x .and. y?=w1051:bool)
            n542 = case shown="False" w1051 {
              selector: w1051 -> [w1064 _]
              tunnel: w1056 -> [w1070 w1088]
              tunnel: w1057 -> [_ w1087]
              tunnel: w1058 -> [_ w1086]
              tunnel: w1055 -> [w1069 w1085]
              tunnel: w1050 -> [w1065 _]
              tunnel: [0.0 ("Progress") w1084] -> w1049
              tunnel: w1044 -> [_ w1084]
              tunnel: w1042 -> [_ _]
              tunnel: w1041 -> [_ w1083]
              tunnel: w1039 -> [w1067 w1082]
              tunnel: w1038 -> [w1063 _]
              tunnel: w1037 -> [w1059 _]
              frame False {
                w1066 = FALSE
                n543 = Close File(refnum=w1070) -> ()  [unwired: 1 in, 2 out]
                n544 = case shown="True" w1065 {
                  tunnel: w1069 -> [_ w1077]
                  frame False {
                  }
                  frame True {
                    n545 = Close File(refnum=w1077) -> ()  [unwired: 1 in, 2 out]
                  }
                }
                n546 = Not(x=w1064) -> (.not. x?=w1062:bool)
                n547 = Not(x=w1063) -> (.not. x?=w1061:bool)
                n548 = call <vilib>:"Beep.vi"() -> ()  [unwired: 12 in]
                n549 = Compound Arithmetic op=AND(w1062, w1061, w1059) -> (w1060:bool)
                n550 = case shown="True" w1060 {
                  tunnel: w1067 -> [_ w1072]
                  frame False {
                  }
                  frame True {
                    n551 = Get Date/Time In Seconds() -> (seconds since 1Jan1904=w1076:timestamp)
                    n552 = Format Date/Time String(time format string (%c)="%H:%M:%S%3u", seconds (now)=w1076, UTC format=TRUE) -> (date/time string=w1071:string)
                    n553 = Write to Text File(file (use dialog)=w1072, text=w1071) -> (refnum out=w1073:refnum<file>)  [unwired: 2 in, 2 out]
                    n554 = Close File(refnum=w1073) -> ()  [unwired: 1 in, 2 out]
                    n555 = local write "Move time"(w1071) -> ()
                  }
                }
                n556 = local write "Saving"(w1066) -> ()
                n557 = local write "Stop saving"(w1066) -> ()
                n558 = local write "Saving Move"(w1066) -> ()
                n559 = local write "Calibrating"(w1066) -> ()
              }
              frame True {
                n560 = local read "Calibrating"() -> (w1081:bool)
                n561 = Not(x=w1081) -> (.not. x?=w1079:bool)
                n562 = And(x=w1079, y=TRUE) -> (x .and. y?=w1078:bool)
                n563 = local write "Saving Move"(w1078) -> ()
                n564 = case shown="True" w1081 {
                  tunnel: w1088 -> [w1117 w1137]
                  tunnel: w1087 -> [_ w1136]
                  tunnel: w1086 -> [w1104 w1130]
                  tunnel: w1085 -> [w1103 _]
                  tunnel: w1083 -> [w1095 _]
                  tunnel: w1082 -> [w1090 _]
                  frame False {
                    n565 = event shown="[0] \"Move time\": Value Change" {
                      selector: _ -> [_ _]
                      dyn-events: _ -> [_ _]
                      timeout: 1 -> [_ _]
                      tunnel: w1090 -> [w1121 _]
                      event "Move time": Value Change {
                        n566 = event-data() -> ("NewVal"=w1120:string)  [unwired: 1 in, 5 out]
                        n567 = Concatenate Strings(w1120, "\r\n") -> (w1118:string)
                        n568 = Write to Text File(file (use dialog)=w1121, text=w1118) -> ()  [unwired: 2 in, 3 out]
                      }
                      event Timeout {
                        n569 = event-data() -> ()  [unwired: 1 in, 3 out]
                      }
                    }
                    n570 = local read "Averaging Number"() -> (w1111:i32)
                    n571 = Array Subset(array=w1104, index (row)=0 ("index"), length (row)=6 ("length")) -> (w1100:dbl[][])  [unwired: 2 in]
                    n572 = Array Subset(array=w1104, index (row)=6 ("index"), length (row)=2 ("length")) -> (w1099:dbl[][])  [unwired: 2 in]
                    n573 = Array Size(array=w1099) -> (size(s)=w1110:i32[])
                    n574 = Array Size(array=w1100) -> (size(s)=w1107:i32[])
                    n575 = Index Array(array=w1095, index=0) -> (element=w1092:waveform(dbl))
                    n576 = Index Array(array=w1095, index=1) -> (element=w1091:waveform(dbl))
                    n577 = for {
                      tunnel: w1100 -> [w1125] mode=indexing
                      tunnel: w1111 -> [w1127]
                      tunnel: [w1126] -> w1098 mode=indexing
                      n578 = call "Downsample 1D array.vi"("Ave N"=w1127, "Arrray In"=w1125) -> ("Array Out"=w1126:dbl[])  [unwired: 9 in]
                    }
                    n579 = Unbundle By Name(w1092) -> ()  [unwired: 1 out]
                    n580 = Unbundle By Name(w1091) -> ()  [unwired: 1 out]
                    n581 = Multiply Array Elements(1:w1107) -> (0:w1106:i32)
                    n582 = for {
                      tunnel: w1099 -> [w1124] mode=indexing
                      tunnel: w1111 -> [w1123]
                      tunnel: [w1122] -> w1102 mode=indexing
                      n583 = call "Downsample 1D array.vi"("Ave N"=w1123, "Arrray In"=w1124) -> ("Array Out"=w1122:dbl[])  [unwired: 9 in]
                    }
                    n584 = Multiply Array Elements(1:w1110) -> (0:w1109:i32)
                    n585 = Divide(x=w1106, y=w1111) -> (x/y=w1112:dbl)
                    n586 = Divide(x=w1109, y=w1111) -> (x/y=w1108:dbl)
                    n587 = Transpose 2D Array(2D array=w1098) -> (transposed array=w1097:dbl[][])
                    n588 = Transpose 2D Array(2D array=w1102) -> (transposed array=w1096:dbl[][])
                    n589 = Reshape Array(w1097, w1112) -> (w1101:dbl[])
                    n590 = Reshape Array(w1096, w1108) -> (w1105:dbl[])
                    n591 = call <vilib>:"Write File+ [SGL].vi"("1D array"=w1105, "refnum"=w1103) -> ()  [unwired: 7 in, 3 out]
                    n592 = call <vilib>:"Write File+ [SGL].vi"("1D array"=w1101, "refnum"=w1117) -> ()  [unwired: 7 in, 3 out]
                  }
                  frame True {
                    n593 = Array Subset(array=w1130, index (row)=0 ("index"), length (row)=6 ("length")) -> (w1128:dbl[][])  [unwired: 2 in]
                    n594 = Transpose 2D Array(2D array=w1128) -> (transposed array=w1134:dbl[][])
                    n595 = Array Size(array=w1128) -> (size(s)=w1129:i32[])
                    n596 = Multiply Array Elements(1:w1129) -> (0:w1135:i32)
                    n597 = Reshape Array(w1134, w1135) -> (w1133:dbl[])
                    n598 = call <vilib>:"Write File+ [SGL].vi"("1D array"=w1133, "error in (no error)"=w1136, "refnum"=w1137) -> ()  [unwired: 6 in, 3 out]
                  }
                }
              }
            }
            "Progress" <- w1049
          }
        }
      }
    }
    n599 = Square Root(x=w434) -> (sqrt(x)=→"Force noise (pN)":dbl)
    n600 = local read "Flushing Sample"() -> (w366:bool)
    n601 = case shown="True" w366 {
      frame False {
      }
      frame True {
        n602 = local read "Flush Sample Start Time"() -> (w777:u32)
        n603 = local read "Sample flush time (s)"() -> (w770:dbl)
        n604 = Tick Count (ms)() -> (millisecond timer value=w778:u32)
        n605 = Subtract(x=w778, y=w777) -> (x-y=w768:u32)
        n606 = Multiply(x=u32 1000, y=w770) -> (x*y=w769:dbl)
        n607 = Divide(x=w768, y=w769) -> (x/y=w773:dbl)
        n608 = Greater?(x=w768, y=w769) -> (0:w776:bool)
        n609 = Not(x=w776) -> (.not. x?=w775:bool)
        n610 = Boolean To (0,1)(Boolean=w775) -> (0, 1=w774:i16)
        n611 = Compound Arithmetic op=MULTIPLY(w774, w773, 100.0 ("value")) -> (→"Sample Flush Meter":dbl)
        n612 = case shown="True" w776 {
          frame False {
          }
          frame True {
            w780 = FALSE ("Inject Sample")
            n613 = property on="Clear Volume" class="Bool (strict)"("Val(Sgnl)"=TRUE ("Value (Signaling)")) -> ()  [unwired: 2 in, 2 out]
            n614 = local write "Inject Sample"(w780) -> ()
            n615 = local write "Flushing Sample"(w780) -> ()
          }
        }
      }
    }
    n616 = feedback #12(0) -> (w350:i32)
    n617 = feedback #13(0) -> (w347:i32)
    n618 = feedback #14(0) -> (w352:i32)
    n619 = case shown="True" w357 {
      tunnel: w361 -> [w670 w727]
      tunnel: [w670 w711] -> w360
      tunnel: w359 -> [w669 w726]
      tunnel: [w669 w710] -> w358
      tunnel: "Raster scan" -> [w668 w704]
      tunnel: [w668 w703] -> w355
      tunnel: [0 w702] -> w353
      tunnel: w352 -> [_ w696]
      tunnel: w350 -> [_ w684]
      tunnel: [0 w687] -> w349
      tunnel: w347 -> [_ w693]
      tunnel: [0 w692] -> w346
      frame False {
      }
      frame True {
        # "Reset step counter"
        # "Current position"
        # "Initial values"
        n620 = local read "Conv Y (nm/V)"() -> (w679:dbl)
        n621 = local read "Conv X (nm/V)"() -> (w680:dbl)
        n622 = local read "Trap delta (nm)"() -> (w678:dbl)
        n623 = disable-structure shown="Disabled" {
          frame Disabled {
            n624 = local write "Raster scan"(FALSE ("Raster scan")) -> ()
            n625 = property on="Reset data stream" class="Bool (strict)"("Val(Sgnl)"=TRUE) -> ()  [unwired: 2 in, 2 out]
          }
          frame Enabled {
          }
        }
        n626 = local read "Data update period (s/set)"() -> (w701:dbl)
        n627 = local read "Time per step (ms)"() -> (w698:dbl)
        n628 = Select(t=w679, s="Pulling direction", f=w680) -> (s? t:f=w677:dbl)
        n629 = Divide(x=w678, y=w677) -> (x/y=w676:dbl)
        n630 = local read "Fixed X"() -> (w720:dbl)
        n631 = local read "Fixed Y"() -> (w721:dbl)
        n632 = local read "Fixed X"() -> (w682:dbl)
        n633 = local read "Fixed Y"() -> (w681:dbl)
        n634 = local read "Trap position (V)"() -> (w683:cluster{"X":dbl, "Y":dbl})
        n635 = Select(t=w681, s="Pulling direction", f=w682) -> (s? t:f=w675:dbl)
        n636 = local read "Scan steps (mirror)"() -> (w709:u64)
        n637 = Unbundle(w683) -> ("X"=w673:dbl, "Y"=w674:dbl)
        n638 = Multiply(x=w701, y=1000.0) -> (x*y=w699:dbl)
        n639 = local read "Stop raster"() -> (w716:bool)
        n640 = local read "Stop saving"() -> (w717:bool)
        n641 = Select(t=w720, s="Pulling direction", f=w721) -> (s? t:f=w728:dbl)
        n642 = Add(x=w676, y=w675) -> ()  [unwired: 1 out]
        n643 = Divide(x=w698, y=w699) -> (x/y=w697:dbl)
        n644 = Quotient & Remainder(x=w696, y=w697) -> (x-y*floor(x/y)=w695:dbl)  [unwired: 1 out]
        n645 = Not(x=w716) -> (.not. x?=w715:bool)
        n646 = Select(t=w674, s="Pulling direction", f=w673) -> (s? t:f=w671:dbl)
        n647 = Not(x=w717) -> (.not. x?=w714:bool)
        n648 = Multiply(x=u64 2, y=w709) -> (x*y=w705:u64)
        n649 = Equal To 0?(x=w695) -> (x = 0?=w694:bool)
        n650 = Less?(x=w684, y=w705) -> (x < y?=w706:bool)
        n651 = Compound Arithmetic op=AND(w706, w715, w714, w694) -> (w707:bool)
        n652 = Not(x=w706) -> (.not. x?=w690:bool)
        n653 = feedback #15() -> (w712:dbl)  [unwired: 1 in]
        n654 = case shown="True" w707 {
          tunnel: w728 -> [_ w763]
          tunnel: w671 -> [_ w745]
          tunnel: w727 -> [w740 w762]
          tunnel: w726 -> [w739 w761]
          tunnel: [w740 w760] -> w711
          tunnel: [w739 w759] -> w710
          tunnel: [w736 w748] -> w713
          tunnel: w684 -> [w737 w743]
          tunnel: w712 -> [w736 w742]
          tunnel: w704 -> [w738 w747]
          tunnel: [w738 w747] -> w703
          tunnel: [w737 w746] -> w688
          frame False {
          }
          frame True {
            # "Go forward or backward?"
            n655 = local read "Scan increment (V)"() -> (w741:dbl)
            n656 = local read "Scan steps (mirror)"() -> (w752:u64)
            n657 = Multiply(x=w741, y=w743) -> (x*y=w744:dbl)
            n658 = Less?(x=w743, y=w752) -> (x < y?=w751:bool)
            n659 = Add(x=w745, y=w744) -> (x+y=w754:dbl)
            n660 = Subtract(x=w742, y=w741) -> (x-y=w753:dbl)
            n661 = Select(t=w754, s=w751, f=w753) -> (s? t:f=w748:dbl)
            n662 = local read "Pulling direction"() -> (w750:bool)
            n663 = Build Array(w748, w763) -> (w757:dbl[])
            n664 = Build Array(w763, w748) -> (w756:dbl[])
            n665 = Select(t=w757, s=w750, f=w756) -> (s? t:f=w755:dbl[])
            n666 = call-poly <vilib>:"DAQmx Write.vi"("task/channels in"=w762, "auto start"=TRUE, "data"=w755, "error in"=w761) -> ("task out"=w760:refnum<k21>, "error out"=w759:errorcluster)  [unwired: 9 in, 1 out]
            n667 = Increment(x=w743) -> (x+1=w746:i32)
            "Raster scanning..." <- TRUE ("Raster scanning...")
          }
        }
        n668 = feedback-in #15(w713) -> ()
        n669 = case shown="True" w690 {
          tunnel: w693 -> [w733 w735]
          tunnel: [w733 w734] -> w692
          frame False {
          }
          frame True {
            n670 = Increment(x=w735) -> (x+1=w734:i32)
          }
        }
        n671 = local read "# scans"() -> (w691:i32)
        n672 = local read "Stop saving"() -> (w719:bool)
        n673 = Greater Or Equal?(x=w692, y=w691) -> (x >= y?=w685:bool)
        n674 = Not(x=w685) -> (.not. x?=w686:bool)
        n675 = And(x=w690, y=w686) -> (x .and. y?=w689:bool)
        n676 = Compound Arithmetic op=OR(w685, "Stop raster", w719) -> (w722:bool)
        n677 = case shown="True" w722 {
          frame False {
          }
          frame True {
            n678 = flat-sequence {
              frame #0 {
                n679 = Wait (ms)(milliseconds to wait=u32 300) -> ()  [unwired: 1 out]
              }
              frame #1 {
                n680 = property on="Trap delta (nm)" class="DigNum (strict)"("Val(Sgnl)"="Trap delta\nafter (nm)") -> ()  [unwired: 2 in, 2 out]
              }
            }
          }
        }
        n681 = And(x="Flow on\nafter raster?", y=w722) -> (x .and. y?=w723:bool)
        n682 = case shown="True" w723 {
          frame False {
          }
          frame True {
            n683 = property on="Inject Sample" class="Bool (strict)"("Val(Sgnl)"=TRUE ("Value (Signaling)")) -> ()  [unwired: 2 in, 2 out]
          }
        }
        n684 = case shown="True" w689 {
          tunnel: w688 -> [w731 _]
          tunnel: [w731 0] -> w687
          frame False {
          }
          frame True {
          }
        }
        n685 = Not(x=w722) -> (.not. x?=w725:bool)
        n686 = local write "Raster scanning..."(w725) -> ()
        n687 = Increment(x=w696) -> (x+1=w702:i32)
      }
    }
    n688 = And(x="Save scans", y=w355) -> (x .and. y?=w364:bool)
    n689 = feedback-in #12(w349) -> ()
    n690 = feedback-in #13(w346) -> ()
    n691 = feedback-in #14(w353) -> ()
    n692 = local read "Stop"() -> (w643:bool)
  }
  n693 = local write "Progress"(u8 0 ("Progress")) -> ()
  n694 = local write "Calibrating"(FALSE ("Calibrating")) -> ()
  n695 = VISA Open(VISA resource name="USB port") -> (VISA resource name=w12:refnum<visa-resource-name>, error out=w11:errorcluster)  [unwired: 1 in, 3 out]
  n696 = VISA Enable Event(8:w11, 10:w10, 11:w12) -> (0:w7:errorcluster, 3:w8:refnum<visa-resource-name>)  [unwired: 1 out]
  n697 = call-poly "VISA Configure Serial Port"("VISA resource name"=refnum<visa-resource-name> "COM5", "baud rate (9600)"=u32 19200) -> ("VISA resource name out"=w2:refnum<visa-resource-name>, "error out"=w28:errorcluster)  [unwired: 12 in]
  n698 = while {
    tunnel: w2 -> [w1219]
    shift-right: [w1215] -> w4
    shift-left: w8 -> [w1218]
    shift-right: [w1216] -> w3
    shift-left: w7 -> [w1217]
    stop <- w1214 stop-if-true
    n699 = global read "FAST_Global_var.vi" "FAST L"() -> (→"FAST Z" →"FAST Z":bool)
    n700 = global read "FAST_Global_var.vi" "FAST R"() -> (→"FAST X-Y" →"FAST X-Y":bool)
    n701 = call "LogitechSubVi.vi"("USB port"=w1218, "VISA resource name in 2 (for the Newport)"=w1219, "error in (no error)"=w1217, "X-Y Wait time"="X-Y Wait time", "Z Wait time"="Z Wait time", "XY Speed Definitions"="XY Speed Definitions", "Z Speed Definitions"="Z Speed Definitions") -> ("Right stick button"=→"Right stick button":bool, "Left stick button"=→"Left stick button":bool, "USB port out"=w1215:refnum<visa-resource-name>, "error out"=w1216:errorcluster, "A B X Y"=w1208:cluster{"A":bool, "B":bool, "X":bool, "Y":bool}, "LB RB"=w1207:T21, "U D L R"=w1213:cluster{"U":bool, "D":bool, "L":bool, "R":bool}, "Sticks"=w1206:T22)  [unwired: 5 in]
    n702 = Unbundle By Name(w1207) -> ("LB"=w1201:bool, "RB"=w1200:bool, "BACK"=w1174:bool, "Logitech"=w1173:bool, "START"=w1175:bool)
    "RB" <- w1200
    "LB" <- w1201
    "BACK" <- w1174
    "START" <- w1175
    "Logitech" <- w1173
    n703 = case shown="True" w1175 {
      selector: w1175 -> [_ w1223]
      frame False {
      }
      frame True {
        n704 = property on="Move to Position 2" class="Bool (strict)"("Val(Sgnl)"=w1223) -> ()  [unwired: 2 in, 2 out]
      }
    }
    n705 = case shown="True" w1173 {
      frame False {
      }
      frame True {
        n706 = local read "Inject Sample"() -> (w1220:bool)
        n707 = Not(x=w1220) -> (.not. x?=w1221:bool)
        n708 = property on="Inject Sample" class="Bool (strict)"("Val(Sgnl)"=w1221) -> ()  [unwired: 2 in, 2 out]
      }
    }
    n709 = case shown="True" w1201 {
      frame False {
      }
      frame True {
        n710 = local read "Shutter 1 (B)"() -> (w1267:bool)
        n711 = Not(x=w1267) -> (.not. x?=w1266:bool)
        n712 = property on="Shutter 1 (B)" class="Bool (strict)"("Val(Sgnl)"=w1266) -> ()  [unwired: 2 in, 2 out]
      }
    }
    n713 = case shown="True" w1174 {
      selector: w1174 -> [_ w1222]
      frame False {
      }
      frame True {
        n714 = property on="Move to Position 1" class="Bool (strict)"("Val(Sgnl)"=w1222) -> ()  [unwired: 2 in, 2 out]
      }
    }
    n715 = Unbundle By Name(w1213) -> ("U"=→"U":bool, "D"=→"D":bool, "L"=→"L":bool, "R"=→"R":bool)
    n716 = Unbundle By Name(w1208) -> ("A"=w1196:bool, "B"=w1194:bool, "X"=w1199:bool, "Y"=w1192:bool)
    "A" <- w1196
    "B" <- w1194
    "X" <- w1199
    "Y" <- w1192
    n717 = case shown="\"Got ADig\", Default" "A command" {
      tunnel: w1196 -> [w1246 w1248 w1250 w1253]
      frame "Got ADig", Default {
        n718 = case shown="True" w1246 {
          selector: w1246 -> [_ w1247]
          frame False {
          }
          frame True {
            n719 = property on="Got ADig bead" class="Bool (strict)"("Val(Sgnl)"=w1247) -> ()  [unwired: 2 in, 2 out]
          }
        }
      }
      frame "Dump" {
        n720 = case shown="True" w1248 {
          selector: w1248 -> [_ w1249]
          frame False {
          }
          frame True {
            n721 = property on="Dump beads" class="Bool (strict)"("Val(Sgnl)"=w1249) -> ()  [unwired: 2 in, 2 out]
          }
        }
      }
      frame "Fish" {
        n722 = case shown="True" w1250 {
          frame False {
          }
          frame True {
            n723 = local read "Fish"() -> (w1251:bool)
            n724 = Not(x=w1251) -> (.not. x?=w1252:bool)
            n725 = property on="Fish" class="Bool (strict)"("Val(Sgnl)"=w1252) -> ()  [unwired: 2 in, 2 out]
          }
        }
      }
      frame "Got DNA" {
        n726 = case shown="True" w1253 {
          selector: w1253 -> [_ w1254]
          frame False {
          }
          frame True {
            n727 = property on="Got DNA bead" class="Bool (strict)"("Val(Sgnl)"=w1254) -> ()  [unwired: 2 in, 2 out]
          }
        }
      }
    }
    n728 = case shown="True" w1200 {
      frame False {
      }
      frame True {
        n729 = local read "Shutter 2 (A)"() -> (w1265:bool)
        n730 = Not(x=w1265) -> (.not. x?=w1264:bool)
        n731 = property on="Shutter 2 (A)" class="Bool (strict)"("Val(Sgnl)"=w1264) -> ()  [unwired: 2 in, 2 out]
      }
    }
    n732 = Unbundle By Name(w1206) -> ("Right X"=w1178:i8, "Right Y"=w1180:i8, "Left X"=w1182:i8, "Left Y"=w1187:i8)
    n733 = Not Equal?(x=w1187, y=i8 0) -> (x != y?=w1188:bool)
    n734 = case shown="True" w1188 {
      tunnel: w1187 -> [_ w1227]
      frame False {
      }
      frame True {
        "Left Y" <- w1227
      }
    }
    n735 = case shown="\"Got DNA\", Default" "B command" {
      tunnel: w1194 -> [w1237 w1239 w1241 w1243]
      frame "Got DNA", Default {
        n736 = case shown="True" w1237 {
          selector: w1237 -> [_ w1238]
          frame False {
          }
          frame True {
            n737 = property on="Got DNA bead" class="Bool (strict)"("Val(Sgnl)"=w1238) -> ()  [unwired: 2 in, 2 out]
          }
        }
      }
      frame "Got ADig" {
        n738 = case shown="True" w1239 {
          selector: w1239 -> [_ w1240]
          frame False {
          }
          frame True {
            n739 = property on="Got ADig bead" class="Bool (strict)"("Val(Sgnl)"=w1240) -> ()  [unwired: 2 in, 2 out]
          }
        }
      }
      frame "Dump" {
        n740 = case shown="True" w1241 {
          selector: w1241 -> [_ w1242]
          frame False {
          }
          frame True {
            n741 = property on="Dump beads" class="Bool (strict)"("Val(Sgnl)"=w1242) -> ()  [unwired: 2 in, 2 out]
          }
        }
      }
      frame "Fish" {
        n742 = case shown="True" w1243 {
          frame False {
          }
          frame True {
            n743 = local read "Fish"() -> (w1244:bool)
            n744 = Not(x=w1244) -> (.not. x?=w1245:bool)
            n745 = property on="Fish" class="Bool (strict)"("Val(Sgnl)"=w1245) -> ()  [unwired: 2 in, 2 out]
          }
        }
      }
    }
    n746 = Not Equal?(x=w1178, y=i8 0) -> (x != y?=w1179:bool)
    n747 = Not Equal?(x=w1180, y=i8 0) -> (x != y?=w1181:bool)
    n748 = Not Equal?(x=w1182, y=i8 0) -> (x != y?=w1183:bool)
    n749 = case shown="True" w1183 {
      tunnel: w1182 -> [_ w1226]
      frame False {
      }
      frame True {
        "Left X" <- w1226
      }
    }
    n750 = case shown="False" w1179 {
      tunnel: w1178 -> [_ w1224]
      frame False {
      }
      frame True {
        "Right X" <- w1224
      }
    }
    n751 = case shown="False" w1181 {
      tunnel: w1180 -> [_ w1225]
      frame False {
      }
      frame True {
        "Right Y" <- w1225
      }
    }
    n752 = case shown="\"Dump\", Default" "X command" {
      tunnel: w1199 -> [w1255 w1257 w1260 w1262]
      frame "Dump", Default {
        n753 = case shown="True" w1255 {
          selector: w1255 -> [_ w1256]
          frame False {
          }
          frame True {
            n754 = property on="Dump beads" class="Bool (strict)"("Val(Sgnl)"=w1256) -> ()  [unwired: 2 in, 2 out]
          }
        }
      }
      frame "Fish" {
        n755 = case shown="True" w1257 {
          frame False {
          }
          frame True {
            n756 = local read "Fish"() -> (w1259:bool)
            n757 = Not(x=w1259) -> (.not. x?=w1258:bool)
            n758 = property on="Fish" class="Bool (strict)"("Val(Sgnl)"=w1258) -> ()  [unwired: 2 in, 2 out]
          }
        }
      }
      frame "Got ADig" {
        n759 = case shown="True" w1260 {
          selector: w1260 -> [_ w1261]
          frame False {
          }
          frame True {
            n760 = property on="Got ADig bead" class="Bool (strict)"("Val(Sgnl)"=w1261) -> ()  [unwired: 2 in, 2 out]
          }
        }
      }
      frame "Got DNA" {
        n761 = case shown="True" w1262 {
          selector: w1262 -> [_ w1263]
          frame False {
          }
          frame True {
            n762 = property on="Got DNA bead" class="Bool (strict)"("Val(Sgnl)"=w1263) -> ()  [unwired: 2 in, 2 out]
          }
        }
      }
    }
    n763 = case shown="\"Fish\", Default" "Y command" {
      tunnel: w1192 -> [w1228 w1231 w1233 w1235]
      frame "Fish", Default {
        n764 = case shown="True" w1228 {
          frame False {
          }
          frame True {
            n765 = local read "Fish"() -> (w1229:bool)
            n766 = Not(x=w1229) -> (.not. x?=w1230:bool)
            n767 = property on="Fish" class="Bool (strict)"("Val(Sgnl)"=w1230) -> ()  [unwired: 2 in, 2 out]
          }
        }
      }
      frame "Dump" {
        n768 = case shown="True" w1231 {
          selector: w1231 -> [_ w1232]
          frame False {
          }
          frame True {
            n769 = property on="Dump beads" class="Bool (strict)"("Val(Sgnl)"=w1232) -> ()  [unwired: 2 in, 2 out]
          }
        }
      }
      frame "Got ADig" {
        n770 = case shown="True" w1233 {
          selector: w1233 -> [_ w1234]
          frame False {
          }
          frame True {
            n771 = property on="Got ADig bead" class="Bool (strict)"("Val(Sgnl)"=w1234) -> ()  [unwired: 2 in, 2 out]
          }
        }
      }
      frame "Got DNA" {
        n772 = case shown="True" w1235 {
          selector: w1235 -> [_ w1236]
          frame False {
          }
          frame True {
            n773 = property on="Got DNA bead" class="Bool (strict)"("Val(Sgnl)"=w1236) -> ()  [unwired: 2 in, 2 out]
          }
        }
      }
    }
    n774 = local read "Stop"() -> (w1214:bool)
  }
  n775 = VISA Close(VISA resource name=w4, error in (no error)=w3) -> (error out=w5:errorcluster)
  n776 = call <vilib>:"Simple Error Handler.vi"("error in (no error)"=w5) -> ()  [unwired: 1 in, 8 out]
  n777 = node-c288(i64 100 ("Period"), 2 ("Processor")) -> (w30:T13)  [unwired: 2 in]
  n778 = timed-loop {
    timing: w30 -> [_]
    timing-out: [_] -> w29
    tunnel: w2 -> [w1268]
    tunnel: w28 -> [w1270]
    tunnel: [w1268] -> w27
    stop <- w1269 stop-if-true
    n779 = node-c288() -> ()  [unwired: 1 in, 1 out]
    n780 = event shown="[8] \"Continous Dip\": Value Change" {
      selector: _ -> [_ _ _ _ _ _ _ _ _ _ _ _ _ _ _]
      dyn-events: _ -> [_ _ _ _ _ _ _ _ _ _ _ _ _ _ _]
      timeout: _ -> [_ _ _ _ _ _ _ _ _ _ _ _ _ _ _]
      tunnel: w1268 -> [w1277 w1328 w1348 w1366 w1383 w1403 w1442 w1455 w1511 _ _ _ _ _ _]
      tunnel: w1270 -> [w1276 w1327 w1347 w1365 w1382 w1402 w1441 w1454 w1509 _ _ _ _ _ _]
      tunnel: [_ _ _ _ _ _ _ _ _ _ _ _ _ _ w1671] -> w1269
      event "Got DNA bead": Value Change {
        n781 = event-data() -> ()  [unwired: 1 in, 5 out]
        n782 = flat-sequence {
          tunnel: w1277 -> [w1282]
          tunnel: w1276 -> [w1280]
          tunnel: ["Cal @ Delta (nm)"] -> w1272
          tunnel: [w1296] -> w1275
          tunnel: w1272 -> [w1295]
          tunnel: w1275 -> [w1317]
          tunnel: [w1317] -> w1274
          tunnel: w1274 -> [w1319]
          tunnel: [w1319] -> w1273
          tunnel: w1273 -> [w1321]
          frame #0 {
            n783 = local read "Saved stage positions"() -> (w1283:dbl[][])
            n784 = disable-structure shown="Disabled" {
              frame Disabled {
                n785 = property on="Inject Pump 2" class="Bool (strict)"("Val(Sgnl)"=FALSE ("Inject Pump 2")) -> ()  [unwired: 2 in, 2 out]
              }
              frame Enabled {
              }
            }
            n786 = property on="Inject Sample" class="Bool (strict)"("Val(Sgnl)"=TRUE ("Value (Signaling)")) -> ()  [unwired: 2 in, 2 out]
            n787 = local write "Stage moving"(TRUE ("Stage moving")) -> ()
            n788 = property on="Trap delta (nm)" class="DigNum (strict)"("Val(Sgnl)"="Cal @ Delta (nm)") -> ()  [unwired: 2 in, 2 out]
            n789 = call "move to saved stage position.vi"("error in"=w1280, "Stage VISA resource name in"=w1282, "Position"="Cal stage position", "Saved Stage Positions"=w1283) -> ()  [unwired: 2 out]
          }
          frame #1 {
            n790 = local write "Stage moving"(FALSE ("Stage moving")) -> ()
            n791 = property on="Inject Sample" class="Bool (strict)"("Val(Sgnl)"=FALSE ("Value (Signaling)")) -> ()  [unwired: 2 in, 2 out]
            n792 = call <vilib>:"Beep.vi"() -> ()  [unwired: 12 in]
          }
          frame #2 {
            # "increased from 1000 to 5000 v6.4. \nMar.7,2018."
            n793 = Wait (ms)(milliseconds to wait=u32 5000) -> ()  [unwired: 1 out]
          }
          frame #3 {
            n794 = property on="Save cal" class="Bool (strict)"("Val(Sgnl)"=TRUE ("Value (Signaling)")) -> ()  [unwired: 2 in, 2 out]
          }
          frame #4 {
            n795 = Wait (ms)(milliseconds to wait=u32 2000) -> ()  [unwired: 1 out]
          }
          frame #5 {
            n796 = while {
              stop <- w1292 stop-if-true
              n797 = local read "Saving"() -> (w1293:bool)
              n798 = Not(x=w1293) -> (.not. x?=w1292:bool)
              n799 = Wait (ms)(milliseconds to wait=u32 100) -> ()  [unwired: 1 out]
            }
          }
          frame #6 {
            n800 = Wait (ms)(milliseconds to wait=u32 2000) -> ()  [unwired: 1 out]
          }
          frame #7 {
            n801 = stacked-sequence {
              tunnel: [_ _ _ _ _ _ w1311 _] -> w1296
              tunnel: w1295 -> [_ _ _ _ _ _ _ w1316]
              frame #0 {
                n802 = property on="Trap delta (nm)" class="DigNum (strict)"("Val(Sgnl)"="Offset @ Delta (nm)") -> ()  [unwired: 2 in, 2 out]
                n803 = Replace Array Subset(array=i32[] [0], new element="Offset raster set", index=0) -> (w1300:i32[])
                n804 = property on="Scan Parameters" class="Arr (strict)"("Index Values"=w1300) -> ()  [unwired: 2 in, 2 out]
              }
              frame #1 {
                n805 = Wait (ms)(milliseconds to wait=u32 200) -> ()  [unwired: 1 out]
              }
              frame #2 {
                n806 = property on="Load param" class="Bool (strict)"("Val(Sgnl)"=TRUE ("Load param")) -> ()  [unwired: 2 in, 2 out]
              }
              frame #3 {
                n807 = Wait (ms)(milliseconds to wait=u32 200) -> ()  [unwired: 1 out]
              }
              frame #4 {
                # "Only continue if there is no buffer\noverflow error"
                n808 = local read "Buffer Overflow"() -> (w1306:bool)
                n809 = Not(x=w1306) -> (.not. x?=w1305:bool)
                n810 = case shown="True" w1305 {
                  frame False {
                  }
                  frame True {
                    n811 = property on="Raster scan" class="Bool (strict)"("Val(Sgnl)"=TRUE ("Value (Signaling)")) -> ()  [unwired: 2 in, 2 out]
                  }
                }
              }
              frame #5 {
                n812 = local read "Buffer Overflow"() -> (w1309:bool)
                n813 = Not(x=w1309) -> (.not. x?=w1308:bool)
                n814 = case shown="True" w1308 {
                  frame False {
                  }
                  frame True {
                    n815 = Wait (ms)(milliseconds to wait=u32 2000) -> ()  [unwired: 1 out]
                  }
                }
              }
              frame #6 {
                n816 = local read "Buffer Overflow"() -> (w1312:bool)
                n817 = Not(x=w1312) -> (.not. x?=w1311:bool)
                n818 = case shown="True" w1311 {
                  frame False {
                  }
                  frame True {
                    n819 = while {
                      stop <- w1314 stop-if-true
                      n820 = local read "Saving"() -> (w1315:bool)
                      n821 = Not(x=w1315) -> (.not. x?=w1314:bool)
                      n822 = Wait (ms)(milliseconds to wait=u32 100) -> ()  [unwired: 1 out]
                    }
                  }
                }
              }
              frame #7 {
                n823 = property on="Trap delta (nm)" class="DigNum (strict)"("Val(Sgnl)"=w1316) -> ()  [unwired: 2 in, 2 out]
              }
            }
          }
          frame #8 {
            n824 = case shown="True" w1317 {
              frame False {
              }
              frame True {
                n825 = property on="Read Cal" class="Bool (strict)"("Val(Sgnl)"=TRUE ("Value (Signaling)")) -> ()  [unwired: 2 in, 2 out]
              }
            }
          }
          frame #9 {
            n826 = case shown="True" w1319 {
              frame False {
              }
              frame True {
                n827 = Wait (ms)(milliseconds to wait=u32 1000) -> ()  [unwired: 1 out]
              }
            }
          }
          frame #10 {
            n828 = case shown="True" w1321 {
              frame False {
              }
              frame True {
                n829 = property on="Fish" class="Bool (strict)"("Val(Sgnl)"=TRUE ("Value (Signaling)")) -> ()  [unwired: 2 in, 2 out]
                n830 = case shown="True" "Flow on\nwhile fish?" {
                  frame False {
                  }
                  frame True {
                    n831 = property on="Inject Sample" class="Bool (strict)"("Val(Sgnl)"=TRUE ("Value (Signaling)")) -> ()  [unwired: 2 in, 2 out]
                  }
                }
              }
            }
          }
        }
        n832 = local write "Got DNA bead"(FALSE) -> ()
      }
      event "Dump beads": Value Change {
        n833 = event-data() -> ()  [unwired: 1 in, 5 out]
        n834 = flat-sequence {
          tunnel: w1327 -> [w1331]
          tunnel: w1328 -> [w1332]
          tunnel: [w1332] -> w1326
          tunnel: [w1331] -> w1325
          tunnel: w1326 -> [w1335]
          tunnel: w1325 -> [w1334]
          frame #0 {
            w1329 = FALSE ("Fish")
            n835 = local read "Saving"() -> (w1330:bool)
            n836 = local write "Force Feedback 2"(w1329) -> ()
            n837 = local write "Pause dwell"(w1329) -> ()
            n838 = local write "Force Feedback 1"(w1329) -> ()
            n839 = local write "Dump beads"(w1329) -> ()
            n840 = property on="Stop saving" class="Bool (strict)"("Val(Sgnl)"=w1330) -> ()  [unwired: 2 in, 2 out]
            n841 = local write "Fish"(w1329) -> ()
          }
          frame #1 {
            n842 = local read "Saved stage positions"() -> (w1337:dbl[][])
            n843 = case shown="True" "Flow on\ndump?" {
              frame False {
              }
              frame True {
                n844 = property on="Inject Sample" class="Bool (strict)"("Val(Sgnl)"=TRUE ("Value (Signaling)")) -> ()  [unwired: 2 in, 2 out]
              }
            }
            n845 = local write "Stage moving"(TRUE ("Stage moving")) -> ()
            n846 = call "move to saved stage position.vi"("error in"=w1334, "Stage VISA resource name in"=w1335, "Position"=5, "Saved Stage Positions"=w1337) -> ()  [unwired: 2 out]
          }
          frame #2 {
            n847 = local read "Shutter 1 (B)"() -> (w1342:bool)
            n848 = local read "Shutter 2 (A)"() -> (w1341:bool)
            n849 = call <vilib>:"Beep.vi"() -> ()  [unwired: 12 in]
            n850 = case shown="True" w1342 {
              frame False {
              }
              frame True {
                n851 = property on="Shutter 1 (B)" class="Bool (strict)"("Val(Sgnl)"=FALSE ("Value (Signaling)")) -> ()  [unwired: 2 in, 2 out]
              }
            }
            n852 = case shown="True" w1341 {
              frame False {
              }
              frame True {
                n853 = property on="Shutter 2 (A)" class="Bool (strict)"("Val(Sgnl)"=FALSE) -> ()  [unwired: 2 in, 2 out]
              }
            }
            n854 = local write "Stage moving"(FALSE ("Stage moving")) -> ()
            n855 = local write "Tether"(FALSE ("Tether")) -> ()
          }
          frame #3 {
            n856 = property on="Move Cap. 2 (ADig Top)" class="Bool (strict)"("Val(Sgnl)"=TRUE ("Value (Signaling)")) -> ()  [unwired: 2 in, 2 out]
          }
        }
      }
      event "Move Cap. 2 (ADig Top)": Value Change {
        n857 = event-data() -> ()  [unwired: 1 in, 5 out]
        n858 = flat-sequence {
          tunnel: w1348 -> [w1352]
          tunnel: w1347 -> [w1351]
          frame #0 {
            n859 = local read "Saved stage positions"() -> (w1350:dbl[][])
            n860 = case shown="True" "Flow on\ncap 2?" {
              frame False {
              }
              frame True {
                n861 = property on="Inject Sample" class="Bool (strict)"("Val(Sgnl)"=TRUE ("Value (Signaling)")) -> ()  [unwired: 2 in, 2 out]
              }
            }
            n862 = local write "Move Cap. 2 (ADig Top)"(FALSE ("Move Cap. 2 (ADig Top)")) -> ()
            n863 = local write "Stage moving"(TRUE ("Stage moving")) -> ()
            n864 = call "move to saved stage position.vi"("error in"=w1351, "Stage VISA resource name in"=w1352, "Position"=2, "Saved Stage Positions"=w1350) -> ()  [unwired: 2 out]
          }
          frame #1 {
            # "Make sure you don't reverse\nwhich is ON and OFF"
            n865 = local read "Cal @ Delta (nm)"() -> (w1360:dbl)
            n866 = local write "Stage moving"(FALSE ("Stage moving")) -> ()
            n867 = call <vilib>:"Beep.vi"() -> ()  [unwired: 12 in]
            n868 = property on="Trap delta (nm)" class="DigNum (strict)"("Val(Sgnl)"=w1360) -> ()  [unwired: 2 in, 2 out]
            n869 = property class="TabCtl (strict)"("Val(Sgnl)"=T4."Status" ("Value (Signaling)")) -> ()  [unwired: 2 in, 2 out]
            n870 = disable-structure shown="Disabled" {
              frame Disabled {
                n871 = property on="Inject Pump 1" class="Bool (strict)"("Val(Sgnl)"=TRUE ("Inject Pump 2")) -> ()  [unwired: 2 in, 2 out]
              }
              frame Enabled {
              }
            }
            n872 = local read "Shutter 2 (A)"() -> (w1359:bool)
            n873 = case shown="False" w1359 {
              frame False {
                n874 = property on="Shutter 2 (A)" class="Bool (strict)"("Val(Sgnl)"=TRUE ("Value (Signaling)")) -> ()  [unwired: 2 in, 2 out]
              }
              frame True {
              }
            }
            n875 = property on="Inject Sample" class="Bool (strict)"("Val(Sgnl)"=FALSE ("Value (Signaling)")) -> ()  [unwired: 2 in, 2 out]
          }
        }
      }
      event "Got ADig bead": Value Change {
        n876 = event-data() -> ()  [unwired: 1 in, 5 out]
        n877 = flat-sequence {
          tunnel: w1366 -> [w1370]
          tunnel: w1365 -> [w1369]
          frame #0 {
            n878 = local read "Saved stage positions"() -> (w1372:dbl[][])
            n879 = property on="Inject Pump 1" class="Bool (strict)"("Val(Sgnl)"=FALSE ("Inject Pump 2")) -> ()  [unwired: 2 in, 2 out]
            n880 = case shown="True" "Flow on\ncap 1?" {
              frame False {
              }
              frame True {
                n881 = property on="Inject Sample" class="Bool (strict)"("Val(Sgnl)"=TRUE ("Value (Signaling)")) -> ()  [unwired: 2 in, 2 out]
              }
            }
            n882 = local write "Stage moving"(TRUE ("Stage moving")) -> ()
            n883 = call "move to saved stage position.vi"("error in"=w1369, "Stage VISA resource name in"=w1370, "Position"=1, "Saved Stage Positions"=w1372) -> ()  [unwired: 2 out]
          }
          frame #1 {
            n884 = local read "Shutter 1 (B)"() -> (w1376:bool)
            n885 = disable-structure shown="Disabled" {
              frame Disabled {
                n886 = property on="Inject Pump 2" class="Bool (strict)"("Val(Sgnl)"=TRUE ("Inject Pump 2")) -> ()  [unwired: 2 in, 2 out]
              }
              frame Enabled {
              }
            }
            n887 = local write "Stage moving"(FALSE ("Stage moving")) -> ()
            n888 = case shown="False" w1376 {
              frame False {
                n889 = property on="Shutter 1 (B)" class="Bool (strict)"("Val(Sgnl)"=TRUE ("Value (Signaling)")) -> ()  [unwired: 2 in, 2 out]
              }
              frame True {
              }
            }
            n890 = property on="Inject Sample" class="Bool (strict)"("Val(Sgnl)"=FALSE ("Value (Signaling)")) -> ()  [unwired: 2 in, 2 out]
            n891 = call <vilib>:"Beep.vi"() -> ()  [unwired: 12 in]
          }
        }
        n892 = local write "Got ADig bead"(FALSE ("Got ADig bead")) -> ()
      }
      event "Set Position 1", "Set Position 2", "Set Position 3", "Set Position 4", "Set Position 5": Value Change {
        n893 = event-data() -> ()  [unwired: 1 in, 5 out]
        n894 = Build Array("Set Position 1", "Set Position 2", "Set Position 3", "Set Position 4", "Set Position 5") -> (w1395:bool[])
        n895 = Boolean Array To Number(Boolean array=w1395) -> (number=w1394:u32)
        n896 = call "Read Stage Position.vi"("error in"=w1382, "VISA resource name in"=w1383) -> ("Current Position"=w1380:cluster{dbl, dbl, dbl}, "error out"=→"Stage error":errorcluster)  [unwired: 1 in, 1 out]
        n897 = Logarithm Base 2(1:w1394) -> (0:w1388:dbl)
        n898 = Cluster To Array(cluster=w1380) -> (array=w1390:dbl[])
        n899 = Increment(x=w1388) -> (x+1=w1391:dbl)
        n900 = Build Array (concatenate)(w1391, w1390) -> (w1389:dbl[])
        n901 = Replace Array Subset(array="Saved stage positions", new element=w1389, index (row)=w1388) -> (w1392:dbl[][])  [unwired: 1 in]
        n902 = local write "Saved stage positions"(w1392) -> ()
      }
      event "Move to Position 2", "Move to Position 4", "Move to Position 3", "Move to Position 5", "Move to Position 1": Value Change {
        w1397 = FALSE
        n903 = event-data() -> ()  [unwired: 1 in, 5 out]
        n904 = Build Array("Move to Position 1", "Move to Position 2", "Move to Position 3", "Move to Position 4", "Move to Position 5") -> (w1406:bool[])
        n905 = Boolean Array To Number(Boolean array=w1406) -> (number=w1405:u32)
        n906 = Logarithm Base 2(1:w1405) -> (0:w1404:dbl)
        n907 = flat-sequence {
          tunnel: w1404 -> [w1415]
          tunnel: w1403 -> [w1414]
          tunnel: w1402 -> [w1413]
          frame #0 {
            # "only change move time when \nsaving move in T and calibrating is F"
            n908 = local read "Saved stage positions"() -> (w1416:dbl[][])
            n909 = property on="Saving Move" class="Bool (strict)"() -> ("Value"=w1409:bool)  [unwired: 2 in, 2 out]
            n910 = property on="Calibrating" class="Bool (strict)"() -> ("Value"=w1410:bool)  [unwired: 2 in, 2 out]
            n911 = Not(x=w1410) -> (.not. x?=w1408:bool)
            n912 = Increment(x=w1415) -> (x+1=w1412:dbl)
            n913 = And(x=w1409, y=w1408) -> (x .and. y?=w1411:bool)
            n914 = case shown="True" w1411 {
              frame False {
              }
              frame True {
                n915 = Get Date/Time In Seconds() -> (seconds since 1Jan1904=w1419:timestamp)
                n916 = Format Date/Time String(time format string (%c)="%H:%M:%S%3u", seconds (now)=w1419, UTC format=TRUE) -> (date/time string=w1418:string)
                n917 = property on="Move time" class="Str"("Val(Sgnl)"=w1418) -> ()  [unwired: 2 in, 2 out]
              }
            }
            n918 = call "move to saved stage position.vi"("error in"=w1413, "Stage VISA resource name in"=w1414, "Position"=w1412, "Saved Stage Positions"=w1416) -> ()  [unwired: 2 out]
            n919 = call <vilib>:"Beep.vi"() -> ()  [unwired: 12 in]
            "Stage moving" <- TRUE ("Stage moving")
          }
          frame #1 {
            n920 = property on="Saving Move" class="Bool (strict)"() -> ("Value"=w1423:bool)  [unwired: 2 in, 2 out]
            n921 = property on="Calibrating" class="Bool (strict)"() -> ("Value"=w1424:bool)  [unwired: 2 in, 2 out]
            n922 = call <vilib>:"Beep.vi"() -> ()  [unwired: 12 in]
            n923 = Not(x=w1424) -> (.not. x?=w1422:bool)
            n924 = local write "Stage moving"(FALSE ("Stage moving")) -> ()
            n925 = And(x=w1423, y=w1422) -> (x .and. y?=w1425:bool)
            n926 = case shown="True" w1425 {
              frame False {
              }
              frame True {
                n927 = Get Date/Time In Seconds() -> (seconds since 1Jan1904=w1428:timestamp)
                n928 = Format Date/Time String(time format string (%c)="%H:%M:%S%3u", seconds (now)=w1428, UTC format=TRUE) -> (date/time string=w1427:string)
                n929 = property on="Move time" class="Str"("Val(Sgnl)"=w1427) -> ()  [unwired: 2 in, 2 out]
              }
            }
          }
        }
        n930 = local write "Move to Position 1"(w1397) -> ()
        n931 = local write "Move to Position 2"(w1397) -> ()
        n932 = local write "Move to Position 3"(w1397) -> ()
        n933 = local write "Move to Position 4"(w1397) -> ()
        n934 = local write "Move to Position 5"(w1397) -> ()
      }
      event "Set Current\nPos to (0,0,0)": Value Change {
        w1432 = ";" ("string")
        # "DH is \"Define Home\" -KW"
        n935 = event-data() -> ()  [unwired: 1 in, 5 out]
        n936 = local write "Set Current\nPos to (0,0,0)"(FALSE ("Set Current\nPos to (0,0,0)")) -> ()
        n937 = call-poly "VISA Configure Serial Port"("VISA resource name"=w1442, "baud rate (9600)"=u32 19200, "error in (no error)"=w1441) -> ("VISA resource name out"=w1436:refnum<visa-resource-name>, "error out"=w1435:errorcluster)  [unwired: 11 in]
        n938 = Concatenate Strings("1DH" ("string"), w1432, "2DH" ("string"), w1432, "3DH" ("string"), "\r") -> (w1434:string)
        n939 = VISA Write(VISA resource name=w1436, write buffer=w1434, error in (no error)=w1435) -> (error out=w1433:errorcluster)  [unwired: 2 out]
        n940 = local write "Stage error"(w1433) -> ()
      }
      event "Dip": Value Change {
        n941 = event-data() -> ()  [unwired: 1 in, 5 out]
        n942 = property on="Calibrating" class="Bool (strict)"() -> ("Value"=w1447:bool)  [unwired: 2 in, 2 out]
        n943 = Not(x=w1447) -> (.not. x?=w1445:bool)
        n944 = property on="Saving Move" class="Bool (strict)"() -> ("Value"=w1446:bool)  [unwired: 2 in, 2 out]
        n945 = And(x=w1446, y=w1445) -> (x .and. y?=w1444:bool)
        n946 = flat-sequence {
          tunnel: w1455 -> [w1458]
          tunnel: w1454 -> [w1457]
          tunnel: [w1459] -> w1452
          tunnel: [w1458] -> w1450
          tunnel: [w1457] -> w1448
          tunnel: w1444 -> [w1456]
          tunnel: [w1472] -> w1453
          tunnel: w1452 -> [w1472]
          tunnel: [w1471] -> w1451
          tunnel: w1450 -> [w1471]
          tunnel: [w1470] -> w1449
          tunnel: w1448 -> [w1470]
          tunnel: w1444 -> [w1466]
          tunnel: w1453 -> [w1497]
          tunnel: w1451 -> [w1496]
          tunnel: w1449 -> [w1495]
          tunnel: w1444 -> [w1491]
          tunnel: w1444 -> [w1502]
          frame #0 {
            n947 = local read "Saved stage positions"() -> (w1459:dbl[][])
            n948 = case shown="True" w1456 {
              frame False {
              }
              frame True {
                n949 = Get Date/Time In Seconds() -> (seconds since 1Jan1904=w1465:timestamp)
                n950 = Format Date/Time String(time format string (%c)="%H:%M:%S%3u", seconds (now)=w1465, UTC format=TRUE) -> (date/time string=w1462:string)
                n951 = property on="Move time" class="Str"("Val(Sgnl)"=w1462) -> ()  [unwired: 2 in, 2 out]
              }
            }
            n952 = local write "Stage moving"(TRUE) -> ()
            n953 = call "move to saved stage position.vi"("error in"=w1457, "Stage VISA resource name in"=w1458, "Position"="Dip position", "Saved Stage Positions"=w1459) -> ()  [unwired: 2 out]
          }
          frame #1 {
            n954 = node-c288() -> (w1469:T13)  [unwired: 4 in]
            n955 = case shown="True" w1466 {
              frame False {
              }
              frame True {
                n956 = Get Date/Time In Seconds() -> (seconds since 1Jan1904=w1476:timestamp)
                n957 = Format Date/Time String(time format string (%c)="%H:%M:%S%3u", seconds (now)=w1476, UTC format=TRUE) -> (date/time string=w1473:string)
                n958 = property on="Move time" class="Str"("Val(Sgnl)"=w1473) -> ()  [unwired: 2 in, 2 out]
              }
            }
            n959 = timed-loop {
              timing: w1469 -> [_]
              timing-out: [_] -> w1468
              i -> [w1486]
              stop <- w1477 stop-if-true
              n960 = node-c288() -> ()  [unwired: 1 in, 1 out]
              n961 = Greater Or Equal?(x=w1486, y="Dip duration") -> (x >= y?=w1482:bool)
              n962 = local read "Dump beads"() -> (w1479:bool)
              n963 = Or(x=w1482, y="Cancel dwell") -> (x .or. y?=w1480:bool)
              n964 = Not(x="Pause dwell") -> (.not. x?=w1483:bool)
              n965 = node-c288() -> ()  [unwired: 1 in, 1 out]
              n966 = And(x=w1483, y=w1480) -> (x .and. y?=w1478:bool)
              n967 = Or(x=w1478, y=w1479) -> (x .or. y?=w1477:bool)
              "Dip elasped time" <- w1486
            }
            n968 = local write "Stage moving"(FALSE ("Stage moving")) -> ()
            n969 = node-c288(w1468) -> ()  [unwired: 1 out]
          }
          frame #2 {
            n970 = case shown="True" w1491 {
              frame False {
              }
              frame True {
                n971 = Get Date/Time In Seconds() -> (seconds since 1Jan1904=w1501:timestamp)
                n972 = Format Date/Time String(time format string (%c)="%H:%M:%S%3u", seconds (now)=w1501, UTC format=TRUE) -> (date/time string=w1498:string)
                n973 = property on="Move time" class="Str"("Val(Sgnl)"=w1498) -> ()  [unwired: 2 in, 2 out]
              }
            }
            n974 = local write "Cancel dwell"(FALSE ("Cancel dwell")) -> ()
            n975 = local write "Stage moving"(TRUE) -> ()
            n976 = call "move to saved stage position.vi"("error in"=w1495, "Stage VISA resource name in"=w1496, "Position"="Start/Return position", "Saved Stage Positions"=w1497) -> ()  [unwired: 2 out]
          }
          frame #3 {
            n977 = case shown="True" w1502 {
              frame False {
              }
              frame True {
                n978 = Get Date/Time In Seconds() -> (seconds since 1Jan1904=w1507:timestamp)
                n979 = Format Date/Time String(time format string (%c)="%H:%M:%S%3u", seconds (now)=w1507, UTC format=TRUE) -> (date/time string=w1504:string)
                n980 = property on="Move time" class="Str"("Val(Sgnl)"=w1504) -> ()  [unwired: 2 in, 2 out]
              }
            }
            n981 = local write "Stage moving"(FALSE ("Stage moving")) -> ()
          }
          frame #4 {
            n982 = local write "Dip"(FALSE ("Dip")) -> ()
          }
        }
      }
      event "Continous Dip": Value Change {
        n983 = event-data() -> ()  [unwired: 1 in, 6 out]
        n984 = local read "Saved stage positions"() -> (w1512:dbl[][])
        n985 = local read "Calibrating"() -> (w1515:bool)
        n986 = local read "Saving Move"() -> (w1514:bool)
        n987 = Not(x=w1515) -> (.not. x?=w1513:bool)
        n988 = And(x=w1514, y=w1513) -> (x .and. y?=w1510:bool)
        n989 = flat-sequence {
          tunnel: w1512 -> [w1519]
          tunnel: w1511 -> [w1518]
          tunnel: w1510 -> [w1517]
          tunnel: w1509 -> [w1516]
          frame #0 {
            n990 = while {
              tunnel: w1519 -> [w1534]
              tunnel: w1518 -> [w1531]
              tunnel: w1517 -> [w1528]
              tunnel: w1517 -> [w1527]
              tunnel: w1516 -> [w1526]
              tunnel: w1516 -> [w1525]
              i -> [w1535]
              stop <- w1524 stop-if-true
              n991 = flat-sequence {
                tunnel: w1534 -> [w1541]
                tunnel: [w1541] -> w1532
                tunnel: w1531 -> [w1540]
                tunnel: [w1540] -> w1529
                tunnel: w1528 -> [w1538]
                tunnel: w1526 -> [w1537]
                tunnel: [w1549] -> w1533
                tunnel: w1532 -> [w1549]
                tunnel: [w1548] -> w1530
                tunnel: w1529 -> [w1548]
                tunnel: w1527 -> [w1547]
                tunnel: w1533 -> [w1576]
                tunnel: w1530 -> [w1575]
                tunnel: w1527 -> [w1573]
                tunnel: w1525 -> [w1572]
                tunnel: w1527 -> [w1582]
                frame #0 {
                  n992 = case shown="True" w1538 {
                    frame False {
                    }
                    frame True {
                      n993 = Get Date/Time In Seconds() -> (seconds since 1Jan1904=w1546:timestamp)
                      n994 = Format Date/Time String(time format string (%c)="%H:%M:%S%3u", seconds (now)=w1546, UTC format=TRUE) -> (date/time string=w1543:string)
                      n995 = property on="Move time" class="Str"("Val(Sgnl)"=w1543) -> ()  [unwired: 2 in, 2 out]
                    }
                  }
                  n996 = local read "Dip position"() -> (w1539:dbl)
                  n997 = local write "Stage moving"(TRUE) -> ()
                  n998 = call "move to saved stage position.vi"("error in"=w1537, "Stage VISA resource name in"=w1540, "Position"=w1539, "Saved Stage Positions"=w1541) -> ()  [unwired: 2 out]
                }
                frame #1 {
                  # "IN DIPPING POSITION"
                  n999 = node-c288() -> (w1552:T13)  [unwired: 4 in]
                  n1000 = case shown="True" w1547 {
                    frame False {
                    }
                    frame True {
                      n1001 = Get Date/Time In Seconds() -> (seconds since 1Jan1904=w1556:timestamp)
                      n1002 = Format Date/Time String(time format string (%c)="%H:%M:%S%3u", seconds (now)=w1556, UTC format=TRUE) -> (date/time string=w1553:string)
                      n1003 = property on="Move time" class="Str"("Val(Sgnl)"=w1553) -> ()  [unwired: 2 in, 2 out]
                    }
                  }
                  n1004 = timed-loop {
                    timing: w1552 -> [_]
                    timing-out: [_] -> w1551
                    i -> [w1565]
                    stop <- w1557 stop-if-true
                    n1005 = node-c288() -> ()  [unwired: 1 in, 1 out]
                    n1006 = local read "Dip duration"() -> (w1564:dbl)
                    n1007 = local read "Cancel dwell"() -> (w1563:bool)
                    n1008 = local write "Dip elasped time"(w1565) -> ()
                    n1009 = To Double Precision Float(number=w1565) -> (double precision float=w1566:dbl)
                    n1010 = local read "Pause dwell"() -> (w1567:bool)
                    n1011 = Greater Or Equal?(x=w1566, y=w1564) -> (x >= y?=w1562:bool)
                    n1012 = local read "Dump beads"() -> (w1558:bool)
                    n1013 = Or(x=w1562, y=w1563) -> (x .or. y?=w1561:bool)
                    n1014 = Not(x=w1567) -> (.not. x?=w1560:bool)
                    n1015 = node-c288() -> ()  [unwired: 1 in, 1 out]
                    n1016 = And(x=w1560, y=w1561) -> (x .and. y?=w1559:bool)
                    n1017 = Or(x=w1559, y=w1558) -> (x .or. y?=w1557:bool)
                  }
                  n1018 = local write "Stage moving"(FALSE) -> ()
                  n1019 = node-c288(w1551) -> ()  [unwired: 1 out]
                }
                frame #2 {
                  n1020 = local read "Start/Return position"() -> (w1574:dbl)
                  n1021 = case shown="True" w1573 {
                    frame False {
                    }
                    frame True {
                      n1022 = Get Date/Time In Seconds() -> (seconds since 1Jan1904=w1581:timestamp)
                      n1023 = Format Date/Time String(time format string (%c)="%H:%M:%S%3u", seconds (now)=w1581, UTC format=TRUE) -> (date/time string=w1578:string)
                      n1024 = property on="Move time" class="Str"("Val(Sgnl)"=w1578) -> ()  [unwired: 2 in, 2 out]
                    }
                  }
                  n1025 = local write "Stage moving"(TRUE) -> ()
                  n1026 = call "move to saved stage position.vi"("error in"=w1572, "Stage VISA resource name in"=w1575, "Position"=w1574, "Saved Stage Positions"=w1576) -> ()  [unwired: 2 out]
                }
                frame #3 {
                  # "IN RETURN POSITION"
                  n1027 = node-c288() -> (w1585:T13)  [unwired: 4 in]
                  n1028 = timed-loop {
                    timing: w1585 -> [_]
                    timing-out: [_] -> w1584
                    i -> [w1599]
                    stop <- w1590 stop-if-true
                    n1029 = node-c288() -> ()  [unwired: 1 in, 1 out]
                    n1030 = local read "Return duration"() -> (w1597:dbl)
                    n1031 = local read "Cancel dwell"() -> (w1595:bool)
                    n1032 = local write "Return elasped time"(w1599) -> ()
                    n1033 = To Double Precision Float(number=w1599) -> (double precision float=w1600:dbl)
                    n1034 = local read "Pause dwell"() -> (w1598:bool)
                    n1035 = Greater Or Equal?(x=w1600, y=w1597) -> (x >= y?=w1596:bool)
                    n1036 = local read "Dump beads"() -> (w1591:bool)
                    n1037 = Or(x=w1596, y=w1595) -> (x .or. y?=w1594:bool)
                    n1038 = Not(x=w1598) -> (.not. x?=w1593:bool)
                    n1039 = node-c288() -> ()  [unwired: 1 in, 1 out]
                    n1040 = And(x=w1593, y=w1594) -> (x .and. y?=w1592:bool)
                    n1041 = Or(x=w1592, y=w1591) -> (x .or. y?=w1590:bool)
                  }
                  n1042 = case shown="True" w1582 {
                    frame False {
                    }
                    frame True {
                      n1043 = Get Date/Time In Seconds() -> (seconds since 1Jan1904=w1589:timestamp)
                      n1044 = Format Date/Time String(time format string (%c)="%H:%M:%S%3u", seconds (now)=w1589, UTC format=TRUE) -> (date/time string=w1586:string)
                      n1045 = property on="Move time" class="Str"("Val(Sgnl)"=w1586) -> ()  [unwired: 2 in, 2 out]
                    }
                  }
                  n1046 = local write "Stage moving"(FALSE) -> ()
                  n1047 = node-c288(w1584) -> ()  [unwired: 1 out]
                }
              }
              n1048 = Increment(x=w1535) -> (x+1=w1522:i32)
              "Dip #" <- w1522
              n1049 = To Double Precision Float(number=w1522) -> (double precision float=w1521:dbl)
              n1050 = local read "Cancel Dip"() -> (w1520:bool)
              n1051 = Greater Or Equal?(x=w1521, y="Dip attempts") -> (x >= y?=w1536:bool)
              n1052 = Or(x=w1520, y=w1536) -> (x .or. y?=w1524:bool)
            }
          }
          frame #1 {
            n1053 = local write "Continous Dip"(FALSE) -> ()
          }
        }
      }
      event "Force FB script": Value Change {
        n1054 = event-data() -> ()  [unwired: 1 in, 5 out]
        n1055 = flat-sequence {
          frame #0 {
            n1056 = disable-structure shown="Disabled" {
              frame Disabled {
                n1057 = local read "# Samples/channel"() -> (w1608:i32)
                n1058 = local write "# Samples/channel (in)"(w1608) -> ()
              }
              frame Enabled {
              }
            }
            n1059 = local write "Force FB script"(FALSE ("Force FB script")) -> ()
            n1060 = property on="Trap delta (nm)" class="DigNum (strict)"("Val(Sgnl)"="Start trap delta (nm)") -> ()  [unwired: 2 in, 2 out]
          }
          frame #1 {
            n1061 = Wait (ms)(milliseconds to wait=u32 500) -> ()  [unwired: 1 out]
          }
          frame #2 {
            n1062 = property on="Set reading to\nsetpoint 1" class="Bool (strict)"("Val(Sgnl)"=TRUE ("Value (Signaling)")) -> ()  [unwired: 2 in, 2 out]
          }
          frame #3 {
            n1063 = Wait (ms)(milliseconds to wait=u32 300) -> ()  [unwired: 1 out]
          }
          frame #4 {
            n1064 = local write "Force Feedback 1"(TRUE ("Force Feedback")) -> ()
            n1065 = property on="Tabs" class="TabCtl (strict)"("Val(Sgnl)"=T23."Force Feedback" ("Value (Signaling)")) -> ()  [unwired: 2 in, 2 out]
          }
          frame #5 {
            n1066 = property on="Save Data" class="Bool (strict)"("Val(Sgnl)"=TRUE ("Value (Signaling)")) -> ()  [unwired: 2 in, 2 out]
          }
          frame #6 {
            n1067 = Multiply(x="Wait before dip (s)", y=1000) -> (x*y=w1615:dbl)
            n1068 = Wait (ms)(milliseconds to wait=w1615) -> ()  [unwired: 1 out]
          }
          frame #7 {
            n1069 = case shown="True" "Start dipping after?" {
              selector: "Start dipping after?" -> [_ w1620]
              frame False {
              }
              frame True {
                n1070 = property on="Dip" class="Bool (strict)"("Val(Sgnl)"=w1620) -> ()  [unwired: 2 in, 2 out]
              }
            }
            n1071 = property on="Remove offsets" class="Bool (strict)"("Val(Sgnl)"=TRUE ("Value (Signaling)")) -> ()  [unwired: 2 in, 2 out]
          }
        }
      }
      event "Move 0": Value Change {
        n1072 = event-data() -> ()  [unwired: 1 in, 5 out]
        n1073 = local write "Move 0"(FALSE) -> ()
        n1074 = call "HalfWavePlate.vi"("Degrees"="\"Degrees\" 0", "Motor"=0) -> ()  [unwired: 1 in]
      }
      event "Move 1": Value Change {
        n1075 = event-data() -> ()  [unwired: 1 in, 5 out]
        n1076 = local write "Move 1"(FALSE) -> ()
        n1077 = call "HalfWavePlate.vi"("Degrees"="\"Degrees\" 1", "Motor"=1) -> ()  [unwired: 1 in]
      }
      event "Save user params": Value Change {
        n1078 = event-data() -> ()  [unwired: 1 in, 6 out]
        n1079 = local write "Save user params"(FALSE) -> ()
        n1080 = call "save control values.vi"("User"="User") -> ()  [unwired: 8 in, 1 out]
      }
      event "Load user params": Value Change {
        # "Exceptions. Don't load these parameters."
        n1081 = event-data() -> ()  [unwired: 1 in, 6 out]
        n1082 = local write "Load user params"(FALSE) -> ()
        n1083 = flat-sequence {
          tunnel: [w1653] -> w1644
          tunnel: [w1652] -> w1642
          tunnel: [w1651] -> w1640
          tunnel: [w1650] -> w1638
          tunnel: [w1649] -> w1636
          tunnel: [w1648] -> w1634
          tunnel: [w1647] -> w1632
          tunnel: [w1646] -> w1629
          tunnel: [w1661] -> w1645
          tunnel: w1644 -> [w1661]
          tunnel: [w1660] -> w1643
          tunnel: w1642 -> [w1660]
          tunnel: [w1659] -> w1641
          tunnel: w1640 -> [w1659]
          tunnel: [w1658] -> w1639
          tunnel: w1638 -> [w1658]
          tunnel: [w1657] -> w1637
          tunnel: w1636 -> [w1657]
          tunnel: [w1656] -> w1635
          tunnel: w1634 -> [w1656]
          tunnel: [w1655] -> w1633
          tunnel: w1632 -> [w1655]
          tunnel: [w1654] -> w1630
          tunnel: w1629 -> [w1654]
          tunnel: w1645 -> [w1670]
          tunnel: w1643 -> [w1669]
          tunnel: w1641 -> [w1668]
          tunnel: w1639 -> [w1667]
          tunnel: w1637 -> [w1666]
          tunnel: w1635 -> [w1665]
          tunnel: w1633 -> [w1664]
          tunnel: w1630 -> [w1663]
          frame #0 {
            n1084 = local read "Force Feedback 2"() -> (w1646:bool)
            n1085 = local read "Force Feedback 1"() -> (w1647:bool)
            n1086 = local read "Shutter 1 (B)"() -> (w1653:bool)
            n1087 = local read "Shutter 2 (A)"() -> (w1652:bool)
            n1088 = local read "Inject Sample"() -> (w1650:bool)
            n1089 = local read "Trap delta (nm)"() -> (w1649:dbl)
            n1090 = local read "Save file index"() -> (w1648:i32)
            n1091 = local read "Fish"() -> (w1651:bool)
          }
          frame #1 {
            n1092 = local read "User"() -> (w1662:string)
            n1093 = call "retrieve control values.vi"("User"=w1662) -> ()  [unwired: 10 in, 1 out]
          }
          frame #2 {
            n1094 = local write "Force Feedback 1"(w1664) -> ()
            n1095 = local write "Force Feedback 2"(w1663) -> ()
            n1096 = local write "Trap delta (nm)"(w1666) -> ()
            n1097 = local write "Save file index"(w1665) -> ()
            n1098 = local write "Inject Sample"(w1667) -> ()
            n1099 = local write "Shutter 2 (A)"(w1669) -> ()
            n1100 = local write "Shutter 1 (B)"(w1670) -> ()
            n1101 = local write "Fish"(w1668) -> ()
          }
        }
      }
      event "Stop": Value Change {
        n1102 = event-data() -> ()  [unwired: 1 in, 5 out]
        n1103 = local read "Stop"() -> (w1671:bool)
      }
    }
    n1104 = node-c288() -> ()  [unwired: 1 in, 1 out]
  }
  n1105 = call-poly <vilib>:"DAQmx Create Virtual Channel.vi"("lines"=w98) -> ("task out"=w97:refnum<k21>)  [unwired: 13 in, 1 out]
  n1106 = call-poly <vilib>:"DAQmx Create Virtual Channel.vi"("lines"=w101) -> ("task out"=w100:refnum<k21>)  [unwired: 13 in, 1 out]
  n1107 = node-c288(2 ("Processor")) -> (w82:T13)  [unwired: 3 in]
  n1108 = timed-loop {
    timing: w82 -> [_]
    timing-out: [_] -> w81
    stop <- w1674 stop-if-true
    n1109 = node-c288() -> ()  [unwired: 1 in, 1 out]
    n1110 = case shown="\"Control\"" "Tab Control" {
      frame "Control" {
        n1111 = case shown="True" "Start" {
          frame False {
          }
          frame True {
            w1687 = T24 3 items=["no dialog", "OK message", "continue or stop message", "OK message + warnings", "continue/stop + warnings"] ("type of dialog (OK msg:1)")
            n1112 = call "InitializeAcquireFF.vi"("DAQ Rate"="DAQ Rate", "Averaging Number"="Averaging Number", "Sampling Rate"="Sampling Rate") -> ("error out"=w1681:errorcluster, "task out"=w1680:refnum<k21>, "Final Sampling Rate"=→"Final Sampling Rate":dbl)  [unwired: 4 in, 2 out]
            n1113 = while {
              tunnel: [w1699] -> w1686
              tunnel: [w1698] -> w1679
              tunnel: "Averaging Number" -> [w1697]
              tunnel: w1681 -> [w1696]
              tunnel: w1680 -> [w1694]
              stop <- w1695 continue-if-true
              n1114 = call "Acquire2_QPD.vi"("task/channels in"=w1694, "Save Data?"=FALSE ("Take Data?"), "Averaging Number"=w1697, "error in"=w1696) -> ("PSD 1"=→"PSD 1":cluster{dbl[], dbl[]}, "PSD 1 Sum"=→"PSD 1 Sum":dbl, "PSD 2"=→"PSD 2":cluster{dbl[], dbl[]}, "PSD 2 Sum"=→"PSD 2 Sum":dbl, "task out"=w1699:refnum<k21>, "error out"=w1698:errorcluster)  [unwired: 14 in, 4 out]
              n1115 = local read "Start"() -> (w1695:bool)
            }
            n1116 = call <vilib>:"DAQmx Clear Task.vi"("task in"=w1686, "error in"=w1679) -> ("error out"=w1688:errorcluster)  [unwired: 13 in]
            n1117 = call <vilib>:"Simple Error Handler.vi"("type of dialog (OK msg:1)"=w1687, "error in (no error)"=w1688) -> ()  [unwired: 3 in, 5 out]
          }
        }
      }
      frame "Current Saved Data" {
      }
      frame "Data Acquisition" {
      }
      frame "Raw QPD Data" {
      }
    }
    n1118 = local read "Stop"() -> (w1674:bool)
    n1119 = node-c288() -> ()  [unwired: 1 in, 1 out]
  }
  n1120 = node-c288(2 ("Processor")) -> (w34:T13)  [unwired: 3 in]
  n1121 = timed-loop {
    timing: w34 -> [_]
    timing-out: [_] -> w33
    stop <- w1700 stop-if-true
    n1122 = node-c288() -> ()  [unwired: 1 in, 1 out]
    n1123 = event shown="[0] \"Pause Mouse/Mirror Connection\": Value Change" {
      selector: _ -> [_ _]
      dyn-events: _ -> [_ _]
      timeout: _ -> [_ _]
      tunnel: [w1793 _] -> w1701
      tunnel: [_ w1794] -> w1700
      event "Pause Mouse/Mirror Connection": Value Change {
        n1124 = event-data() -> ("NewVal"=w1793:bool)  [unwired: 1 in]
      }
      event "Stop": Value Change {
        n1125 = event-data() -> ("NewVal"=w1794:bool)  [unwired: 1 in]
      }
    }
    n1126 = case shown="True" w1701 {
      frame False {
      }
      frame True {
        n1127 = call "InitializeMouseControl.vi"() -> ("error out 2"=w1710:errorcluster, "task out"=w1711:refnum<k21>, "error out"=w1713:errorcluster, "device ID"=w1712:refnum<k1>)  [unwired: 8 in]
        n1128 = while {
          tunnel: w1713 -> [w1725]
          tunnel: w1712 -> [w1724]
          tunnel: w1711 -> [w1723]
          tunnel: w1710 -> [w1722]
          tunnel: [w1721] -> w1708
          tunnel: [w1720] -> w1707
          tunnel: [w1719] -> w1704
          tunnel: [w1718] -> w1705
          stop <- w1717 stop-if-true
          n1129 = case shown="True" "Use Mouse to Move Trap?" {
            tunnel: w1724 -> [w1732 w1755]
            tunnel: w1725 -> [w1731 w1754]
            tunnel: w1723 -> [w1730 w1753]
            tunnel: w1722 -> [w1729 w1752]
            tunnel: [w1732 w1751] -> w1719
            tunnel: [w1731 w1750] -> w1718
            tunnel: [w1730 w1749] -> w1721
            tunnel: [w1729 w1748] -> w1720
            frame False {
              (unwired) FALSE ("button 1")
            }
            frame True {
              w1743 = 0.0 ("y")
              w1745 = 10
              n1130 = local read "Deflection"() -> (w1756:T5)
              n1131 = call-poly <vilib>:"Acquire Input Data.vi"("device ID"=w1755, "error in (no error)"=w1754) -> ("device ID"=w1751:refnum<k1>, "button info"=w1769:T25, "error out"=w1750:errorcluster)  [unwired: 14 in, 1 out]
              n1132 = Unbundle By Name(w1756) -> ("Horizontal"=w1758:i32, "Vertical"=w1757:i32)
              n1133 = local read "Saved voltage"() -> (w1734:cluster{dbl, dbl})
              n1134 = Divide(x=w1758, y=30) -> (x/y=w1761:dbl)
              n1135 = Divide(x=w1757, y=-20) -> (x/y=w1762:dbl)
              n1136 = Unbundle By Name(w1769) -> ("button 1"=w1747:bool, "button 2"=w1763:bool)
              n1137 = Bundle(w1761, w1762) -> (w1739:cluster{dbl, dbl})  [unwired: 1 in]
              n1138 = local write "Reference Voltage"(w1739) -> ()
              n1139 = Add(x=w1739, y=w1734) -> (x+y=w1767:cluster{dbl, dbl})
              n1140 = case shown="True" w1747 {
                frame False {
                  n1141 = stacked-sequence {
                    frame #0 {
                      n1142 = local write "CoordinatesMousePressed"(T5 {"Horizontal"=0, "Vertical"=0} ("Coords when pressed")) -> ()
                      n1143 = local write "Deflection"(T5 {"Horizontal"=0, "Vertical"=0} ("deflaction")) -> ()
                    }
                  }
                }
                frame True {
                  n1144 = local read "CoordinatesMousePressed"() -> (w1792:T5)
                  n1145 = local read "Real Coordinates"() -> (w1791:cluster{"Horizontal":i32, "Vertical":i32})
                  n1146 = Subtract(x=w1791, y=w1792) -> (x-y=w1790:T5)
                  n1147 = local write "Deflection"(w1790) -> ()
                }
              }
              n1148 = Unbundle(w1767) -> (w1744:dbl, w1735:dbl)
              n1149 = case shown="True" w1763 {
                frame False {
                }
                frame True {
                  n1150 = local read "Reference Voltage"() -> (w1773:cluster{dbl, dbl})
                  n1151 = local read "Saved voltage"() -> (w1771:cluster{dbl, dbl})
                  n1152 = Add(x=w1773, y=w1771) -> (x+y=→"Saved voltage":cluster{dbl, dbl})
                  n1153 = local read "Real Coordinates"() -> (w1772:cluster{"Horizontal":i32, "Vertical":i32})
                  n1154 = local write "CoordinatesMousePressed"(w1772) -> ()
                }
              }
              n1155 = Less?(x=w1744, y=w1745) -> (x < y?=w1742:bool)
              n1156 = Greater?(x=w1744, y=w1743) -> (0:w1741:bool)
              n1157 = Greater?(x=w1735, y=w1743) -> (0:w1737:bool)
              n1158 = Less?(x=w1735, y=w1745) -> (x < y?=w1738:bool)
              n1159 = And(x=w1737, y=w1738) -> (x .and. y?=w1736:bool)
              n1160 = And(x=w1742, y=w1741) -> (x .and. y?=w1740:bool)
              n1161 = case shown="False" w1736 {
                tunnel: [w1783 w1787] -> w1746
                tunnel: w1735 -> [w1781 w1787]
                frame False {
                  n1162 = Greater?(x=w1781, y=10.0) -> (0:w1784:bool)
                  n1163 = case shown="True" w1784 {
                    tunnel: [0.0 10.0] -> w1783
                    frame False {
                    }
                    frame True {
                    }
                  }
                }
                frame True {
                }
              }
              n1164 = case shown="False" w1740 {
                tunnel: w1744 -> [w1775 w1780]
                tunnel: [w1776 w1780] -> w1768
                frame False {
                  n1165 = Greater?(x=w1775, y=10.0) -> (0:w1777:bool)
                  n1166 = case shown="True" w1777 {
                    tunnel: [0.0 10.0] -> w1776
                    frame False {
                    }
                    frame True {
                    }
                  }
                }
                frame True {
                }
              }
              n1167 = Bundle(w1768, w1746) -> (w1733:cluster{dbl, dbl})  [unwired: 1 in]
              n1168 = Cluster To Array(cluster=w1733) -> (array=w1764:dbl[])
              n1169 = call-poly <vilib>:"DAQmx Write.vi"("task/channels in"=w1753, "data"=w1764, "error in"=w1752) -> ("task out"=w1766:refnum<k21>, "error out"=w1765:errorcluster)  [unwired: 10 in, 1 out]
              n1170 = call <vilib>:"DAQmx Is Task Done.vi"("task/channels in"=w1766, "error in"=w1765) -> ("task out"=w1749:refnum<k21>, "error out"=w1748:errorcluster)  [unwired: 11 in, 1 out]
            }
          }
          n1171 = event shown="[0] \"Pane\": Mouse Move" {
            selector: _ -> [_ _ _]
            dyn-events: _ -> [_ _ _]
            timeout: _ -> [_ _ _]
            event Mouse Move {
              n1172 = event-data() -> ("Coords"=w1727:T5)  [unwired: 1 in]
              n1173 = local write "Real Coordinates"(w1727) -> ()
            }
            event Mouse Down {
              n1174 = event-data() -> ("Coords"=w1728:T5)  [unwired: 1 in]
              n1175 = local write "CoordinatesMousePressed"(w1728) -> ()
            }
            event "Pause Mouse/Mirror Connection": Value Change {
              n1176 = event-data() -> ()  [unwired: 1 in, 3 out]
            }
          }
          n1177 = local read "Stop"() -> (w1714:bool)
          n1178 = Not(x="Pause Mouse/Mirror Connection") -> (.not. x?=w1715:bool)
          n1179 = Or(x=w1715, y=w1714) -> (x .or. y?=w1717:bool)
        }
        n1180 = call <vilib>:"DAQmx Clear Task.vi"("task in"=w1708, "error in"=w1707) -> ("error out"=w1709:errorcluster)  [unwired: 13 in]
        n1181 = call <vilib>:"Simple Error Handler.vi"("error in (no error)"=w1709) -> ()  [unwired: 4 in, 5 out]
        n1182 = call-poly <vilib>:"Close Input Device.vi"("error in (no error)"=w1705, "device ID"=w1704) -> ("error out"=w1706:errorcluster)  [unwired: 8 in]
        n1183 = call <vilib>:"Simple Error Handler.vi"("error in (no error)"=w1706) -> ()  [unwired: 4 in, 5 out]
      }
    }
    n1184 = node-c288() -> ()  [unwired: 1 in, 1 out]
  }
  n1185 = node-c288(i64 100 ("Period")) -> (w95:T13)  [unwired: 3 in]
  n1186 = timed-loop {
    tunnel: w97 -> [w1797]
    tunnel: [w1796] -> w96
    tunnel: w100 -> [w1799]
    tunnel: [w1798] -> w99
    timing: w95 -> [_]
    timing-out: [_] -> w94
    stop <- w1795 stop-if-true
    n1187 = node-c288() -> ()  [unwired: 1 in, 1 out]
    n1188 = event shown="[1] \"Shutter 2 (A)\": Value Change" {
      selector: _ -> [_ _ _]
      dyn-events: _ -> [_ _ _]
      timeout: _ -> [_ _ _]
      tunnel: w1799 -> [w1803 _ w1840]
      tunnel: [w1802 _ w1840] -> w1798
      tunnel: w1797 -> [_ w1823 w1841]
      tunnel: [_ w1821 w1841] -> w1796
      tunnel: [_ _ w1842] -> w1795
      event "Shutter 1 (B)": Value Change {
        n1189 = event-data() -> ()  [unwired: 1 in, 1 out]
        n1190 = flat-sequence {
          tunnel: [w1809] -> w1806
          tunnel: w1803 -> [w1808]
          tunnel: [w1813] -> w1805
          tunnel: [w1816] -> w1804
          tunnel: w1806 -> [w1811]
          tunnel: w1805 -> [w1820]
          tunnel: w1804 -> [w1818]
          tunnel: [w1817] -> w1802
          frame #0 {
            n1191 = call-poly <vilib>:"DAQmx Write.vi"("task/channels in"=w1808, "data"=FALSE) -> ("task out"=w1809:refnum<k21>)  [unwired: 11 in, 2 out]
            n1192 = Wait (ms)(milliseconds to wait=100) -> ()  [unwired: 1 out]
          }
          frame #1 {
            n1193 = Or(x="Shutter 1 (B)", y=TRUE) -> (x .or. y?=w1813:bool)
            n1194 = call-poly <vilib>:"DAQmx Write.vi"("task/channels in"=w1811, "data"=w1813) -> ("task out"=w1816:refnum<k21>)  [unwired: 11 in, 2 out]
            n1195 = Wait (ms)(milliseconds to wait=100) -> ()  [unwired: 1 out]
          }
          frame #2 {
            n1196 = Not(x=w1820) -> (.not. x?=w1819:bool)
            n1197 = call-poly <vilib>:"DAQmx Write.vi"("task/channels in"=w1818, "data"=w1819) -> ("task out"=w1817:refnum<k21>)  [unwired: 11 in, 2 out]
          }
        }
      }
      event "Shutter 2 (A)": Value Change {
        n1198 = event-data() -> ()  [unwired: 1 in, 1 out]
        n1199 = flat-sequence {
          tunnel: w1823 -> [w1828]
          tunnel: [w1827] -> w1822
          tunnel: [w1832] -> w1825
          tunnel: [w1835] -> w1824
          tunnel: w1822 -> [w1830]
          tunnel: w1825 -> [w1839]
          tunnel: w1824 -> [w1837]
          tunnel: [w1836] -> w1821
          frame #0 {
            n1200 = call-poly <vilib>:"DAQmx Write.vi"("task/channels in"=w1828, "data"=FALSE) -> ("task out"=w1827:refnum<k21>)  [unwired: 11 in, 2 out]
            n1201 = Wait (ms)(milliseconds to wait=100) -> ()  [unwired: 1 out]
          }
          frame #1 {
            n1202 = Or(x="Shutter 2 (A)", y=TRUE) -> (x .or. y?=w1832:bool)
            n1203 = call-poly <vilib>:"DAQmx Write.vi"("task/channels in"=w1830, "data"=w1832) -> ("task out"=w1835:refnum<k21>)  [unwired: 11 in, 2 out]
            n1204 = Wait (ms)(milliseconds to wait=100) -> ()  [unwired: 1 out]
          }
          frame #2 {
            n1205 = Not(x=w1839) -> (.not. x?=w1838:bool)
            n1206 = call-poly <vilib>:"DAQmx Write.vi"("task/channels in"=w1837, "data"=w1838) -> ("task out"=w1836:refnum<k21>)  [unwired: 11 in, 2 out]
          }
        }
      }
      event "Stop": Value Change {
        n1207 = event-data() -> ("NewVal"=w1842:bool)  [unwired: 1 in, 5 out]
      }
    }
    n1208 = node-c288() -> ()  [unwired: 1 in, 1 out]
  }
  n1209 = node-c288(w94) -> ()  [unwired: 1 out]
  n1210 = node-c288(w81) -> ()  [unwired: 1 out]
  n1211 = call <vilib>:"DAQmx Clear Task.vi"("task in"=w96) -> ()  [unwired: 14 in, 1 out]
  n1212 = call <vilib>:"DAQmx Clear Task.vi"("task in"=w99) -> ()  [unwired: 14 in, 1 out]
  n1213 = node-c288(w33) -> ()  [unwired: 1 out]
  n1214 = node-c288(w29) -> ()  [unwired: 1 out]
  n1215 = local write "Tether"(FALSE ("Tether")) -> ()
  n1216 = local read "Path"() -> (w88:path)
  n1217 = node-c288(i64 1 ("Period"), 2 ("Processor")) -> (w93:T13)  [unwired: 2 in]
  n1218 = timed-loop {
    timing: w93 -> [_]
    timing-out: [_] -> w92
    tunnel: w88 -> [w1844]
    stop <- w1843 stop-if-true
    n1219 = node-c288() -> ()  [unwired: 1 in, 1 out]
    n1220 = event shown="[0] Timeout" {
      selector: _ -> [_ _ _ _ _ _ _ _ _ _]
      dyn-events: _ -> [_ _ _ _ _ _ _ _ _ _]
      timeout: _ -> [_ _ _ _ _ _ _ _ _ _]
      tunnel: w1844 -> [_ w1848 _ _ _ _ _ _ _ _]
      tunnel: [_ _ w1868 _ _ _ _ _ _ _] -> w1843
      event Timeout {
        n1221 = event-data() -> ()  [unwired: 1 in, 2 out]
      }
      event "Read Cal": Value Change {
        n1222 = event-data() -> ()  [unwired: 1 in, 6 out]
        n1223 = Path To String(path=w1848) -> (string=w1847:string)
        n1224 = Format Date/Time String(time format string (%c)="%y%m%d") -> (date/time string=w1849:string)  [unwired: 2 in]
        n1225 = Concatenate Strings(w1847, "\\" ("string"), w1849, "\\" ("string"), "current.cal") -> (w1867:string)
        n1226 = String To Path(string=w1867) -> (path=w1866:path)
        n1227 = Open/Create/Replace File(file path (use dialog)=w1866, operation (0:open)=T18."open", access (0:read/write)=enum16{"read/write", "read-only", "write-only"}."read-only") -> (refnum out=w1862:refnum<file>, error out=w1863:errorcluster)  [unwired: 3 in, 1 out]
        n1228 = Deny Access(4:w1863, 7:w1862) -> (0:w1861:errorcluster, 3:w1860:refnum<file>)  [unwired: 1 in]
        n1229 = Read from Binary File(5:0.0, 8:w1861, 9:T19."big-endian, network order" ("byte order (0:big-endian, network order)"), 10:12 ("count"), 11:w1860) -> (0:w1856:errorcluster, 2:w1854:dbl[], 3:w1857:refnum<file>)  [unwired: 1 in, 1 out]
        n1230 = Array To Cluster(array=w1854) -> (cluster=→"Cal values":T26)
        n1231 = Close File(refnum=w1857, error in=w1856) -> ()  [unwired: 2 out]
        n1232 = local write "Read Cal"(FALSE ("Read Cal")) -> ()
      }
      event "Stop": Value Change {
        n1233 = event-data() -> ("NewVal"=w1868:bool)  [unwired: 1 in, 5 out]
      }
      event "Trap position (V)": Value Change {
        # "Need to rotate so X and Y don't get mixed up."
        n1234 = event-data() -> ()  [unwired: 1 in, 6 out]
        n1235 = local read "Mirror task"() -> (w1869:refnum<k21>)
        n1236 = Cluster To Array(cluster="Trap position (V)") -> (array=w1872:dbl[])
        n1237 = Rotate 1D Array(1:w1872, 2:1 ("n")) -> (0:w1870:dbl[])
        n1238 = call-poly <vilib>:"DAQmx Write.vi"("task/channels in"=w1869, "data"=w1870) -> ("task out"=w1875:refnum<k21>, "error out"=w1874:errorcluster)  [unwired: 11 in, 1 out]
        n1239 = call <vilib>:"DAQmx Stop Task.vi"("task/channels in"=w1875, "error in"=w1874) -> ("error out"=w1873:errorcluster)  [unwired: 12 in, 1 out]
        n1240 = call <vilib>:"Simple Error Handler.vi"("error in (no error)"=w1873) -> ()  [unwired: 4 in, 5 out]
      }
      event "Trap delta (nm)": Value Change {
        n1241 = event-data() -> ()  [unwired: 1 in, 6 out]
        n1242 = local read "Pulling direction"() -> (w1877:bool)
        n1243 = local read "Conv Y (nm/V)"() -> (w1878:dbl)
        n1244 = local read "Conv X (nm/V)"() -> (w1879:dbl)
        n1245 = Select(t=w1878, s=w1877, f=w1879) -> (s? t:f=w1880:dbl)
        n1246 = local read "Fixed Y"() -> (w1886:dbl)
        n1247 = Divide(x="Trap delta (nm)", y=w1880) -> (x/y=w1881:dbl)
        n1248 = local read "Fixed X"() -> (w1885:dbl)
        n1249 = Select(t=w1886, s=w1877, f=w1885) -> (s? t:f=w1884:dbl)
        n1250 = Add(x=w1881, y=w1884) -> (x+y=w1882:dbl)
        n1251 = case shown="False" w1877 {
          tunnel: w1882 -> [w1887 w1888]
          frame False {
            n1252 = property on="X" class="DigNum (strict)"("Val(Sgnl)"=w1887) -> ()  [unwired: 2 in, 2 out]
          }
          frame True {
            n1253 = property on="Y" class="DigNum (strict)"("Val(Sgnl)"=w1888) -> ()  [unwired: 2 in, 2 out]
          }
        }
      }
      event "Fish": Value Change {
        n1254 = event-data() -> ()  [unwired: 1 in, 6 out]
        n1255 = local read "Fish"() -> (w1889:bool)
        n1256 = case shown="True" w1889 {
          frame False {
          }
          frame True {
            w1898 = 0.0 ("minimum value")
            w1899 = 10.0 ("maximum value")
            # "Grab offset in pulling\ndirection and add to \ndelta values"
            n1257 = call-poly <vilib>:"DAQmx Create Virtual Channel.vi"("maximum value"=w1899, "minimum value"=w1898, "physical channels"=tag "Dev1/ao0") -> ("task out"=w1903:refnum<k21>, "error out"=w1902:errorcluster)  [unwired: 11 in]
            n1258 = call-poly <vilib>:"DAQmx Create Virtual Channel.vi"("task in"=w1903, "maximum value"=w1899, "minimum value"=w1898, "physical channels"=tag "Dev1/ao1", "error in"=w1902) -> ("task out"=w1897:refnum<k21>, "error out"=w1896:errorcluster)  [unwired: 9 in]
            n1259 = node-c288(i64 1 ("Period")) -> (w1905:T13)  [unwired: 3 in]
            n1260 = timed-loop {
              timing: w1905 -> [_]
              timing-out: [_] -> w1904
              tunnel: w1897 -> [w1973]
              tunnel: w1896 -> [w1972]
              tunnel: [w1971] -> w1892
              tunnel: [w1970] -> w1891
              tunnel: [w1930] -> w1894
              tunnel: [w1931] -> w1890
              i -> [w1956]
              stop <- w1931 stop-if-true
              # "x direction"
              # "y direction"
              # "Send offset in direction\nof not-pulling to DAQ"
              n1261 = node-c288() -> ()  [unwired: 1 in, 1 out]
              n1262 = local read "Pulling direction"() -> (w1935:bool)
              n1263 = local read "Conv Y (nm/V)"() -> (w1937:dbl)
              n1264 = local read "Conv X (nm/V)"() -> (w1936:dbl)
              n1265 = local read "Fixed X"() -> (w1944:dbl)
              n1266 = local read "Fixed Y"() -> (w1943:dbl)
              n1267 = Select(t=w1943, s=w1935, f=w1944) -> (s? t:f=w1945:dbl)
              n1268 = Select(t=w1944, s=w1935, f=w1943) -> (s? t:f=w1942:dbl)
              n1269 = Select(t=w1937, s=w1935, f=w1936) -> (s? t:f=w1932:dbl)
              n1270 = Divide(x="Max fish\ndelta (nm)", y=w1932) -> (x/y=w1934:dbl)
              n1271 = Divide(x="Min fish\ndelta (nm)", y=w1932) -> (x/y=w1933:dbl)
              n1272 = Add(x=w1945, y=w1934) -> (x+y=w1947:dbl)
              n1273 = Subtract(x=w1934, y=w1933) -> (x-y=w1949:dbl)
              n1274 = Divide(x=w1949, y="Fish Speed (ms)") -> (x/y=w1950:dbl)
              n1275 = flat-sequence {
                tunnel: w1935 -> [w1993]
                tunnel: w1942 -> [w1992]
                tunnel: w1973 -> [w1991]
                tunnel: w1972 -> [w1990]
                tunnel: w1950 -> [w1989]
                tunnel: w1947 -> [w1988]
                tunnel: "Fish Speed (ms)" -> [w1983]
                tunnel: [w1987] -> w1969
                tunnel: [w1986] -> w1968
                tunnel: [w1985] -> w1967
                tunnel: [w1984] -> w1966
                tunnel: [w1977] -> w1955
                tunnel: [w1976] -> w1941
                tunnel: [w1975] -> w1938
                tunnel: [w1974] -> w1928
                tunnel: [w2046] -> w1965
                tunnel: w1969 -> [w2046]
                tunnel: [w2045] -> w1964
                tunnel: w1968 -> [w2045]
                tunnel: [w2044] -> w1963
                tunnel: w1967 -> [w2044]
                tunnel: [w2043] -> w1962
                tunnel: w1966 -> [w2043]
                tunnel: w1955 -> [w2042]
                tunnel: [w2042] -> w1954
                tunnel: w1941 -> [w2041]
                tunnel: [w2040] -> w1939
                tunnel: w1938 -> [w2040]
                tunnel: [w2039] -> w1929
                tunnel: w1928 -> [w2039]
                tunnel: w1965 -> [w2058]
                tunnel: w1964 -> [w2057]
                tunnel: w1963 -> [w2056]
                tunnel: w1962 -> [w2055]
                tunnel: w1952 -> [w2054]
                tunnel: [w2053] -> w1971
                tunnel: [w2052] -> w1970
                tunnel: w1954 -> [w2051]
                tunnel: [w2050] -> w1940
                tunnel: w1939 -> [w2049]
                tunnel: [w2048] -> w1927
                tunnel: w1929 -> [w2048]
                frame #0 {
                  n1276 = local read "Mean force (pN)"() -> (w1982:dbl)
                  n1277 = local read "Cutoff force (pN)"() -> (w1981:dbl)
                  n1278 = Less Or Equal?(x=w1982, y=w1981) -> (x <= y?=w1979:bool)
                  n1279 = And(x="Fish", y=w1979) -> (x .and. y?=w1980:bool)
                  n1280 = case shown="True" w1980 {
                    selector: w1980 -> [w1996 _]
                    tunnel: w1993 -> [w1999 w2016]
                    tunnel: w1992 -> [_ w2015]
                    tunnel: w1991 -> [w2001 w2014]
                    tunnel: w1990 -> [w2000 w2013]
                    tunnel: w1989 -> [w1998 w2012]
                    tunnel: w1988 -> [w1997 w2011]
                    tunnel: [w2001 w2010] -> w1987
                    tunnel: [w2000 w2009] -> w1986
                    tunnel: [w1999 w2008] -> w1985
                    tunnel: [w1997 w2007] -> w1975
                    tunnel: [w1998 w2006] -> w1984
                    tunnel: w1983 -> [_ w2005]
                    tunnel: [w1996 w2004] -> w1977
                    tunnel: [FALSE w2003] -> w1976
                    tunnel: [FALSE w2002] -> w1974
                    frame False {
                    }
                    frame True {
                      n1281 = while {
                        tunnel: w2016 -> [w2028]
                        tunnel: w2015 -> [w2027]
                        tunnel: w2014 -> [w2035]
                        tunnel: w2013 -> [w2034]
                        tunnel: w2012 -> [w2026]
                        tunnel: w2011 -> [w2032]
                        tunnel: [w2030] -> w2010
                        tunnel: [w2029] -> w2009
                        tunnel: [w2028] -> w2008
                        tunnel: [w2027] -> w2007
                        tunnel: [w2026] -> w2006
                        tunnel: w2005 -> [w2025]
                        tunnel: [w2018] -> w2004
                        tunnel: [w2018] -> w2003
                        tunnel: [w2017] -> w2002
                        i -> [w2024]
                        stop <- w2021 stop-if-true
                        # "top: x"
                        # "x direction"
                        # "y direction"
                        n1282 = Multiply(x=w2026, y=w2024) -> (x*y=w2033:dbl)
                        n1283 = local read "Cutoff force (pN)"() -> (w2019:dbl)
                        n1284 = local read "Mean force (pN)"() -> (w2020:dbl)
                        n1285 = Subtract(x=w2032, y=w2033) -> (x-y=w2031:dbl)
                        n1286 = Build Array(w2027, w2031) -> (w2038:dbl[])
                        n1287 = Build Array(w2031, w2027) -> (w2037:dbl[])
                        n1288 = Greater Or Equal?(x=w2024, y=w2025) -> (x >= y?=w2018:bool)
                        n1289 = Select(t=w2038, s=w2028, f=w2037) -> (s? t:f=w2036:dbl[])
                        n1290 = Greater?(x=w2020, y=w2019) -> (0:w2017:bool)
                        n1291 = local read "Fish"() -> (w2022:bool)
                        n1292 = Not(x=w2022) -> (.not. x?=w2023:bool)
                        n1293 = call-poly <vilib>:"DAQmx Write.vi"("task/channels in"=w2035, "data"=w2036, "error in"=w2034) -> ("task out"=w2030:refnum<k21>, "error out"=w2029:errorcluster)  [unwired: 10 in, 1 out]
                        n1294 = Compound Arithmetic op=OR(w2018, w2023, w2017) -> (w2021:bool)
                      }
                    }
                  }
                }
                frame #1 {
                  n1295 = case shown="True" w2041 {
                    frame False {
                    }
                    frame True {
                      n1296 = Wait (ms)(milliseconds to wait="Wait (ms)") -> ()  [unwired: 1 out]
                    }
                  }
                }
                frame #2 {
                  n1297 = case shown="True" w2051 {
                    tunnel: w2058 -> [w2061 w2070]
                    tunnel: w2057 -> [w2060 w2069]
                    tunnel: w2056 -> [_ w2068]
                    tunnel: w2055 -> [_ w2067]
                    tunnel: w2054 -> [_ w2066]
                    tunnel: [w2061 w2065] -> w2053
                    tunnel: [w2060 w2064] -> w2052
                    tunnel: [FALSE w2063] -> w2050
                    tunnel: w2049 -> [_ w2062]
                    frame False {
                    }
                    frame True {
                      n1298 = while {
                        tunnel: w2070 -> [w2102]
                        tunnel: w2069 -> [w2101]
                        tunnel: w2068 -> [w2073]
                        tunnel: w2067 -> [w2099]
                        tunnel: w2066 -> [w2098]
                        tunnel: [w2096] -> w2065
                        tunnel: [w2095] -> w2064
                        tunnel: [w2080] -> w2063
                        tunnel: w2062 -> [w2071]
                        i -> [w2087]
                        stop <- w2092 stop-if-true
                        # "y direction"
                        # "If tether formed,\nimmediately change\nto new delta."
                        n1299 = local read "Conv Y (nm/V)"() -> (w2074:dbl)
                        n1300 = local read "Conv X (nm/V)"() -> (w2072:dbl)
                        n1301 = local read "Fixed Y"() -> (w2081:dbl)
                        n1302 = local read "Fixed X"() -> (w2086:dbl)
                        n1303 = Select(t=w2074, s=w2073, f=w2072) -> (s? t:f=w2075:dbl)
                        n1304 = local read "Cutoff force (pN)"() -> (w2088:dbl)
                        n1305 = Divide(x="Delta after tether", y=w2075) -> (x/y=w2076:dbl)
                        n1306 = Multiply(x=w2099, y=w2087) -> (x*y=w2100:dbl)
                        n1307 = local read "Mean force (pN)"() -> (w2089:dbl)
                        n1308 = Add(x=w2098, y=w2100) -> (x+y=w2083:dbl)
                        n1309 = Select(t=w2081, s=w2073, f=w2086) -> (s? t:f=w2085:dbl)
                        n1310 = Greater?(x=w2089, y=w2088) -> (0:w2080:bool)
                        n1311 = Add(x=w2085, y=w2076) -> (x+y=w2084:dbl)
                        n1312 = Select(t=w2084, s=w2080, f=w2083) -> (s? t:f=w2082:dbl)
                        n1313 = local read "Fish Speed (ms)"() -> (w2094:i32)
                        n1314 = Build Array(w2071, w2082) -> (w2097:dbl[])
                        n1315 = Build Array(w2082, w2071) -> (w2078:dbl[])
                        n1316 = Select(t=w2097, s=w2073, f=w2078) -> (s? t:f=w2077:dbl[])
                        n1317 = case shown="True" w2080 {
                          tunnel: w2076 -> [_ _]
                          tunnel: w2077 -> [_ w2104]
                          frame False {
                          }
                          frame True {
                            n1318 = Array To Cluster(array=w2104) -> (cluster=w2103:cluster{"[0]":dbl, "[1]":dbl})
                            n1319 = property on="Trap position (V)" class="Clust (strict)"("Val(Sgnl)"=w2103) -> ()  [unwired: 2 in, 2 out]
                          }
                        }
                        n1320 = local read "Fish"() -> (w2091:bool)
                        n1321 = Greater Or Equal?(x=w2087, y=w2094) -> (x >= y?=w2093:bool)
                        n1322 = Not(x=w2091) -> (.not. x?=w2090:bool)
                        n1323 = call-poly <vilib>:"DAQmx Write.vi"("task/channels in"=w2102, "data"=w2077, "error in"=w2101) -> ("task out"=w2096:refnum<k21>, "error out"=w2095:errorcluster)  [unwired: 10 in, 1 out]
                        n1324 = Compound Arithmetic op=OR(w2093, w2090, w2080) -> (w2092:bool)
                      }
                    }
                  }
                }
              }
              n1325 = Add(x=w1945, y=w1933) -> (x+y=w1952:dbl)
              n1326 = Decrement(x="# attempts") -> (x-1=w1960:dbl)
              n1327 = Greater Or Equal?(x=w1956, y=w1960) -> (x >= y?=w1959:bool)
              n1328 = local read "Mean force (pN)"() -> (w1958:dbl)
              n1329 = Greater?(x=w1958, y="Cutoff force (pN)") -> (0:w1953:bool)
              n1330 = Compound Arithmetic op=OR(w1927, w1940, w1953, w1959) -> (w1931:bool)
              n1331 = Or(x=w1940, y=w1927) -> (x .or. y?=w1930:bool)
              "Tether" <- w1930
              n1332 = case shown="True" w1930 {
                frame False {
                }
                frame True {
                  n1333 = call <vilib>:"Beep.vi"() -> ()  [unwired: 12 in]
                }
              }
              n1334 = node-c288() -> ()  [unwired: 1 in, 1 out]
              "Attempt #" <- w1956
            }
            n1335 = node-c288(w1904) -> ()  [unwired: 1 out]
            n1336 = flat-sequence {
              tunnel: w1894 -> [w1913]
              tunnel: [w1913] -> w1893
              tunnel: w1892 -> [w1910]
              tunnel: w1891 -> [w1909]
              tunnel: w1890 -> [w1906]
              tunnel: w1893 -> [w1915]
              frame #0 {
                w1912 = T24 1 items=["no dialog", "OK message", "continue or stop message", "OK message + warnings", "continue/stop + warnings"] ("type of dialog (OK msg:1)")
                n1337 = call <vilib>:"DAQmx Clear Task.vi"("task in"=w1910, "error in"=w1909) -> ("error out"=w1911:errorcluster)  [unwired: 13 in]
                n1338 = Not(x=w1906) -> (.not. x?=w1907:bool)
                n1339 = local write "Fish"(w1907) -> ()
                n1340 = Wait (ms)(milliseconds to wait=u32 300) -> ()  [unwired: 1 out]
                n1341 = call <vilib>:"Simple Error Handler.vi"("type of dialog (OK msg:1)"=w1912, "error in (no error)"=w1911) -> ()  [unwired: 3 in, 5 out]
              }
              frame #1 {
                n1342 = And(x=w1915, y="Raster after\n tether?") -> (x .and. y?=w1916:bool)
                n1343 = case shown="True" w1916 {
                  selector: w1916 -> [_ w1917]
                  frame False {
                  }
                  frame True {
                    n1344 = stacked-sequence {
                      tunnel: w1917 -> [_ _ _ _ w1926]
                      frame #0 {
                        n1345 = local read "Raster set"() -> (w1921:i32)
                        n1346 = property on="Inject Sample" class="Bool (strict)"("Val(Sgnl)"=FALSE ("Value (Signaling)")) -> ()  [unwired: 2 in, 2 out]
                        n1347 = Replace Array Subset(array=i32[] [0], new element=w1921, index=0) -> (w1918:i32[])
                        n1348 = property on="Scan Parameters" class="Arr (strict)"("Index Values"=w1918) -> ()  [unwired: 2 in, 2 out]
                      }
                      frame #1 {
                        n1349 = Wait (ms)(milliseconds to wait=u32 500) -> ()  [unwired: 1 out]
                      }
                      frame #2 {
                        n1350 = property on="Load param" class="Bool (strict)"("Val(Sgnl)"=TRUE ("Value (Signaling)")) -> ()  [unwired: 2 in, 2 out]
                      }
                      frame #3 {
                        n1351 = Wait (ms)(milliseconds to wait=u32 500) -> ()  [unwired: 1 out]
                      }
                      frame #4 {
                        n1352 = property on="Raster scan" class="Bool (strict)"("Val(Sgnl)"=w1926) -> ()  [unwired: 2 in, 2 out]
                      }
                    }
                  }
                }
              }
            }
          }
        }
      }
      event "Load param": Value Change {
        n1353 = event-data() -> ()  [unwired: 1 in, 6 out]
        n1354 = property on="Scan Parameters" class="Arr (strict)"() -> ("Index Values"=w2120:u32[])  [unwired: 2 in, 2 out]
        n1355 = Index Array(array=w2120, index=0) -> (element=w2117:u32)
        n1356 = Index Array(array="Scan Parameters", index=w2117) -> (element=w2116:T27)
        n1357 = Unbundle(w2116) -> ("Scan range 1"=w2114:dbl, "Step size 1"=w2113:dbl, "Scan speed 1"=w2111:i32, "# scans 2"=w2112:i32)  [unwired: 1 out]
        n1358 = property on="# scans" class="DigNum (strict)"("Val(Sgnl)"=w2112) -> ()  [unwired: 2 in, 2 out]
        n1359 = property on="Scan range (nm)" class="DigNum (strict)"("Val(Sgnl)"=w2114) -> ()  [unwired: 2 in, 2 out]
        n1360 = property on="Step size 1" class="DigNum (strict)"("Val(Sgnl)"=w2113) -> ()  [unwired: 2 in, 2 out]
        n1361 = property on="Scan speed (nm/s)" class="DigNum (strict)"("Val(Sgnl)"=w2111) -> ()  [unwired: 2 in, 2 out]
        n1362 = local write "Load param"(FALSE ("Load param")) -> ()
      }
      event "# scans", "Scan range (nm)", "Step size (nm)", "Scan speed (nm/s)": Value Change {
        n1363 = event-data() -> ()  [unwired: 1 in, 6 out]
        n1364 = local read "Pulling direction"() -> (w2151:bool)
        n1365 = Reciprocal(x="Scan speed (nm/s)") -> (1/x=w2143:dbl)
        n1366 = local read "Conv Y (nm/V)"() -> (w2149:dbl)
        n1367 = local read "Conv X (nm/V)"() -> (w2150:dbl)
        n1368 = Multiply(x="Step size (nm)", y=w2143) -> (x*y=w2141:dbl)
        n1369 = Divide(x="Scan range (nm)", y="Step size (nm)") -> (x/y=w2148:dbl)
        n1370 = Absolute Value(x=w2148) -> (abs(x)=w2147:dbl)
        n1371 = Multiply(x=w2141, y=1000.0) -> (x*y=w2128:dbl)
        n1372 = Select(t=w2149, s=w2151, f=w2150) -> (s? t:f=w2139:dbl)
        n1373 = Multiply(x="# scans", y=2) -> (x*y=w2127:i32)
        n1374 = To Unsigned Quad Integer(1:w2147) -> (0:w2137:u64)
        "Scan steps (mirror)" <- w2137
        n1375 = Divide(x="Scan range (nm)", y=w2139) -> (x/y=→"Scan range (V)":dbl)
        n1376 = Multiply(x=w2137, y=w2128) -> (x*y=w2136:dbl)
        n1377 = Divide(x="Step size (nm)", y=w2139) -> (x/y=→"Scan increment (V)":dbl)
        n1378 = Round Toward +Infinity(x=w2128) -> (ceil(x): smallest int >= x=w2125:dbl)
        "Time per step (ms)" <- w2125
        n1379 = local read "Data update period (s/set)"() -> (w2131:dbl)
        n1380 = Multiply(x=w2127, y=w2136) -> (x*y=w2134:dbl)
        n1381 = Divide(x=w2134, y=1000.0) -> (x/y=w2132:dbl)
        "Total raster time (s)" <- w2132
        n1382 = local read "Data update period (s/set)"() -> (w2123:dbl)
        n1383 = Divide(x=w2132, y=w2131) -> (x/y=w2130:dbl)
        n1384 = Round Toward -Infinity(1:w2130) -> (0:→"N sets to be saved":dbl)
        n1385 = Multiply(x=w2123, y=1000.0) -> (x*y=w2121:dbl)
        n1386 = Less?(x=w2125, y=w2121) -> (x < y?=w2124:bool)
        n1387 = case shown="True" w2124 {
          selector: w2124 -> [_ w2152]
          frame False {
          }
          frame True {
            n1388 = call "Display Message to User"("Enable"=w2152) -> ()  [unwired: 9 in, 2 out]
          }
        }
      }
      event "Pulling direction": Value Change {
        n1389 = event-data() -> ()  [unwired: 1 in, 6 out]
        n1390 = local read "Pulling direction"() -> (w2158:bool)
        n1391 = local read "Conv Y (nm/V)"() -> (w2160:dbl)
        n1392 = local read "Conv X (nm/V)"() -> (w2159:dbl)
        n1393 = local read "Scan range (nm)"() -> (w2157:dbl)
        n1394 = Select(t=w2160, s=w2158, f=w2159) -> (s? t:f=w2154:dbl)
        n1395 = local read "Step size (nm)"() -> (w2155:dbl)
        n1396 = case shown="False" w2158 {
          frame False {
            n1397 = local read "Fixed Y"() -> (w2163:dbl)
            n1398 = local read "Trap delta (nm)"() -> (w2168:dbl)
            n1399 = local read "Conv X (nm/V)"() -> (w2167:dbl)
            n1400 = local read "Fixed X"() -> (w2165:dbl)
            n1401 = Divide(x=w2168, y=w2167) -> (x/y=w2166:dbl)
            n1402 = Add(x=w2166, y=w2165) -> (x+y=w2164:dbl)
            n1403 = Build Array(w2164, w2163) -> (w2162:dbl[])
            n1404 = Array To Cluster(array=w2162) -> (cluster=w2161:cluster{"[0]":dbl, "[1]":dbl})
            n1405 = property on="Trap position (V)" class="Clust (strict)"("Val(Sgnl)"=w2161) -> ()  [unwired: 2 in, 2 out]
          }
          frame True {
            n1406 = local read "Trap delta (nm)"() -> (w2176:dbl)
            n1407 = local read "Conv Y (nm/V)"() -> (w2175:dbl)
            n1408 = local read "Fixed X"() -> (w2171:dbl)
            n1409 = local read "Fixed Y"() -> (w2173:dbl)
            n1410 = Divide(x=w2176, y=w2175) -> (x/y=w2174:dbl)
            n1411 = Add(x=w2174, y=w2173) -> (x+y=w2172:dbl)
            n1412 = Build Array(w2171, w2172) -> (w2170:dbl[])
            n1413 = Array To Cluster(array=w2170) -> (cluster=w2169:cluster{"[0]":dbl, "[1]":dbl})
            n1414 = property on="Trap position (V)" class="Clust (strict)"("Val(Sgnl)"=w2169) -> ()  [unwired: 2 in, 2 out]
          }
        }
        n1415 = Divide(x=w2157, y=w2154) -> (x/y=w2156:dbl)
        n1416 = Divide(x=w2155, y=w2154) -> (x/y=w2153:dbl)
        n1417 = local write "Scan range (V)"(w2156) -> ()
        n1418 = local write "Scan increment (V)"(w2153) -> ()
      }
      event "Averaging Number": Value Change {
        n1419 = event-data() -> ()  [unwired: 1 in, 6 out]
        n1420 = local read "# Samples/channel (in)"() -> (w2180:i32)
        n1421 = local read "Averaging Number"() -> (w2178:i32)
        n1422 = Quotient & Remainder(x=w2180, y=w2178) -> (floor(x/y)=w2179:i32)  [unwired: 1 out]
        n1423 = Multiply(x=w2179, y=w2178) -> (x*y=w2177:i32)
        n1424 = local write "# Samples/channel (in)"(w2177) -> ()
      }
    }
    n1425 = node-c288() -> ()  [unwired: 1 in, 1 out]
  }
  n1426 = VISA Close(VISA resource name=w27) -> (error out=w105:errorcluster)  [unwired: 1 in]
  n1427 = call <vilib>:"Simple Error Handler.vi"("error in (no error)"=w105) -> ()  [unwired: 4 in, 5 out]
  n1428 = disable-structure shown="Enabled" {
    frame Disabled {
      n1429 = node-c288(2 ("Processor")) -> (w2186:T13)  [unwired: 3 in]
      n1430 = timed-loop "Pump Control" {
        timing: w2186 -> [_]
        timing-out: [_] -> w2185
        tunnel: refnum<visa-resource-name> "COM6" ("VISA resource name") -> [w2188]
        stop <- w2187 stop-if-true
        n1431 = node-c288() -> ()  [unwired: 1 in, 1 out]
        n1432 = event shown="[4] \"Inject Pump 1\": Value Change" {
          selector: _ -> [_ _ _ _ _ _ _ _ _]
          dyn-events: _ -> [_ _ _ _ _ _ _ _ _]
          timeout: _ -> [_ _ _ _ _ _ _ _ _]
          tunnel: w2188 -> [w2196 w2292 _ w2368 w2496 w2639 w2684 w2742 w2801]
          tunnel: [_ _ w2367 _ _ _ _ _ _] -> w2187
          event "Flush Pump 1": Value Change {
            w2197 = "\r"
            n1433 = event-data() -> ()  [unwired: 1 in, 5 out]
            n1434 = call-poly "VISA Configure Serial Port"("VISA resource name"=w2196) -> ("VISA resource name out"=w2210:refnum<visa-resource-name>, "error out"=w2211:errorcluster)  [unwired: 13 in]
            n1435 = local read "Write Wait"() -> (w2189:i32)
            n1436 = Concatenate Strings("enter pump1", w2197) -> (w2198:string)
            n1437 = flat-sequence {
              tunnel: w2211 -> [w2230]
              tunnel: w2210 -> [w2232]
              tunnel: [w2231] -> w2227
              tunnel: [w2229] -> w2226
              tunnel: w2198 -> [w2228]
              tunnel: w2227 -> [w2235]
              tunnel: [w2235] -> w2225
              tunnel: w2226 -> [w2234]
              tunnel: [w2234] -> w2224
              tunnel: w2189 -> [w2233]
              tunnel: [w2240] -> w2223
              tunnel: w2203 -> [w2239]
              tunnel: [w2236] -> w2222
              tunnel: w2225 -> [w2238]
              tunnel: w2224 -> [w2237]
              tunnel: w2223 -> [w2243]
              tunnel: [w2243] -> w2221
              tunnel: [w2242] -> w2220
              tunnel: w2222 -> [w2242]
              tunnel: w2189 -> [w2241]
              tunnel: w2221 -> [w2248]
              tunnel: [w2247] -> w2219
              tunnel: w2206 -> [w2246]
              tunnel: w2220 -> [w2245]
              tunnel: [w2244] -> w2218
              tunnel: w2219 -> [w2251]
              tunnel: [w2251] -> w2217
              tunnel: [w2250] -> w2216
              tunnel: w2218 -> [w2250]
              tunnel: w2189 -> [w2249]
              tunnel: w2217 -> [w2256]
              tunnel: [w2255] -> w2215
              tunnel: w2209 -> [w2254]
              tunnel: w2216 -> [w2253]
              tunnel: [w2252] -> w2214
              tunnel: [w2259] -> w2213
              tunnel: w2215 -> [w2259]
              tunnel: [w2258] -> w2212
              tunnel: w2214 -> [w2258]
              tunnel: w2189 -> [w2257]
              tunnel: w2213 -> [w2264]
              tunnel: w2212 -> [w2261]
              tunnel: [w2263] -> w2192
              tunnel: [w2262] -> w2190
              tunnel: [w2269] -> w2193
              tunnel: w2192 -> [w2269]
              tunnel: [w2268] -> w2191
              tunnel: w2190 -> [w2268]
              tunnel: w2189 -> [w2267]
              tunnel: w2193 -> [w2271]
              tunnel: w2191 -> [w2270]
              frame #0 {
                n1438 = VISA Write(VISA resource name=w2232, write buffer=w2228, error in (no error)=w2230) -> (VISA resource name out=w2231:refnum<visa-resource-name>, error out=w2229:errorcluster)  [unwired: 1 out]
              }
              frame #1 {
                n1439 = Wait (ms)(milliseconds to wait=w2233) -> ()  [unwired: 1 out]
              }
              frame #2 {
                n1440 = VISA Write(VISA resource name=w2238, write buffer=w2239, error in (no error)=w2237) -> (VISA resource name out=w2240:refnum<visa-resource-name>, error out=w2236:errorcluster)  [unwired: 1 out]
              }
              frame #3 {
                n1441 = Wait (ms)(milliseconds to wait=w2241) -> ()  [unwired: 1 out]
              }
              frame #4 {
                n1442 = VISA Write(VISA resource name=w2248, write buffer=w2246, error in (no error)=w2245) -> (VISA resource name out=w2247:refnum<visa-resource-name>, error out=w2244:errorcluster)  [unwired: 1 out]
              }
              frame #5 {
                n1443 = Wait (ms)(milliseconds to wait=w2249) -> ()  [unwired: 1 out]
              }
              frame #6 {
                n1444 = VISA Write(VISA resource name=w2256, write buffer=w2254, error in (no error)=w2253) -> (VISA resource name out=w2255:refnum<visa-resource-name>, error out=w2252:errorcluster)  [unwired: 1 out]
              }
              frame #7 {
                n1445 = Wait (ms)(milliseconds to wait=w2257) -> ()  [unwired: 1 out]
              }
              frame #8 {
                n1446 = Concatenate Strings("start ", "\r") -> (w2260:string)
                n1447 = VISA Write(VISA resource name=w2264, write buffer=w2260, error in (no error)=w2261) -> (VISA resource name out=w2263:refnum<visa-resource-name>, error out=w2262:errorcluster)  [unwired: 1 out]
              }
              frame #9 {
                n1448 = Wait (ms)(milliseconds to wait=w2267) -> ()  [unwired: 1 out]
              }
              frame #10 {
                n1449 = local write "Flush Pump 1"(FALSE ("Flush Pump 1")) -> ()
                n1450 = Concatenate Strings("enter main ", "\r") -> (w2275:string)
                n1451 = VISA Write(VISA resource name=w2271, write buffer=w2275, error in (no error)=w2270) -> (VISA resource name out=w2274:refnum<visa-resource-name>, error out=w2273:errorcluster)  [unwired: 1 out]
                n1452 = VISA Close(VISA resource name=w2274, error in (no error)=w2273) -> ()  [unwired: 1 out]
              }
            }
            n1453 = Concatenate Strings("set units 4 ", w2197) -> (w2203:string)
            n1454 = Multiply(x="Flush\nRate (ul/min)", y=60) -> (x*y=w2201:dbl)
            n1455 = Number To Decimal String(number=w2201) -> (decimal integer string=w2204:string)  [unwired: 1 in]
            n1456 = Concatenate Strings("set rate ", w2204, w2197) -> (w2206:string)
            n1457 = Number To Decimal String(number="Flush\nVolume (ul)") -> (decimal integer string=w2208:string)  [unwired: 1 in]
            n1458 = Concatenate Strings("set volume ", w2208, w2197) -> (w2209:string)
          }
          event "Flush Pump 2": Value Change {
            w2283 = "\r"
            n1459 = event-data() -> ()  [unwired: 1 in, 5 out]
            n1460 = call-poly "VISA Configure Serial Port"("VISA resource name"=w2292) -> ("VISA resource name out"=w2303:refnum<visa-resource-name>, "error out"=w2304:errorcluster)  [unwired: 13 in]
            n1461 = local read "Write Wait"() -> (w2278:i32)
            n1462 = Concatenate Strings("enter pump2", w2283) -> (w2284:string)
            n1463 = flat-sequence {
              tunnel: w2304 -> [w2319]
              tunnel: w2303 -> [w2321]
              tunnel: [w2320] -> w2289
              tunnel: [w2318] -> w2287
              tunnel: w2284 -> [w2317]
              tunnel: w2289 -> [w2324]
              tunnel: [w2324] -> w2288
              tunnel: w2287 -> [w2323]
              tunnel: [w2323] -> w2286
              tunnel: w2278 -> [w2322]
              tunnel: [w2329] -> w2316
              tunnel: w2296 -> [w2328]
              tunnel: [w2325] -> w2315
              tunnel: w2288 -> [w2327]
              tunnel: w2286 -> [w2326]
              tunnel: w2316 -> [w2332]
              tunnel: [w2332] -> w2314
              tunnel: [w2331] -> w2313
              tunnel: w2315 -> [w2331]
              tunnel: w2278 -> [w2330]
              tunnel: w2314 -> [w2337]
              tunnel: [w2336] -> w2312
              tunnel: w2299 -> [w2335]
              tunnel: w2313 -> [w2334]
              tunnel: [w2333] -> w2311
              tunnel: w2312 -> [w2340]
              tunnel: [w2340] -> w2310
              tunnel: [w2339] -> w2309
              tunnel: w2311 -> [w2339]
              tunnel: w2278 -> [w2338]
              tunnel: w2310 -> [w2345]
              tunnel: [w2344] -> w2308
              tunnel: w2302 -> [w2343]
              tunnel: w2309 -> [w2342]
              tunnel: [w2341] -> w2307
              tunnel: [w2348] -> w2306
              tunnel: w2308 -> [w2348]
              tunnel: [w2347] -> w2305
              tunnel: w2307 -> [w2347]
              tunnel: w2278 -> [w2346]
              tunnel: w2306 -> [w2355]
              tunnel: w2305 -> [w2354]
              tunnel: [w2350] -> w2282
              tunnel: [w2349] -> w2280
              tunnel: w2282 -> [w2358]
              tunnel: [w2358] -> w2281
              tunnel: w2280 -> [w2357]
              tunnel: [w2357] -> w2279
              tunnel: w2278 -> [w2356]
              tunnel: w2281 -> [w2362]
              tunnel: w2279 -> [w2361]
              frame #0 {
                n1464 = VISA Write(VISA resource name=w2321, write buffer=w2317, error in (no error)=w2319) -> (VISA resource name out=w2320:refnum<visa-resource-name>, error out=w2318:errorcluster)  [unwired: 1 out]
              }
              frame #1 {
                n1465 = Wait (ms)(milliseconds to wait=w2322) -> ()  [unwired: 1 out]
              }
              frame #2 {
                n1466 = VISA Write(VISA resource name=w2327, write buffer=w2328, error in (no error)=w2326) -> (VISA resource name out=w2329:refnum<visa-resource-name>, error out=w2325:errorcluster)  [unwired: 1 out]
              }
              frame #3 {
                n1467 = Wait (ms)(milliseconds to wait=w2330) -> ()  [unwired: 1 out]
              }
              frame #4 {
                n1468 = VISA Write(VISA resource name=w2337, write buffer=w2335, error in (no error)=w2334) -> (VISA resource name out=w2336:refnum<visa-resource-name>, error out=w2333:errorcluster)  [unwired: 1 out]
              }
              frame #5 {
                n1469 = Wait (ms)(milliseconds to wait=w2338) -> ()  [unwired: 1 out]
              }
              frame #6 {
                n1470 = VISA Write(VISA resource name=w2345, write buffer=w2343, error in (no error)=w2342) -> (VISA resource name out=w2344:refnum<visa-resource-name>, error out=w2341:errorcluster)  [unwired: 1 out]
              }
              frame #7 {
                n1471 = Wait (ms)(milliseconds to wait=w2346) -> ()  [unwired: 1 out]
              }
              frame #8 {
                n1472 = Concatenate Strings("start ", "\r") -> (w2353:string)
                n1473 = VISA Write(VISA resource name=w2355, write buffer=w2353, error in (no error)=w2354) -> (VISA resource name out=w2350:refnum<visa-resource-name>, error out=w2349:errorcluster)  [unwired: 1 out]
              }
              frame #9 {
                n1474 = Wait (ms)(milliseconds to wait=w2356) -> ()  [unwired: 1 out]
              }
              frame #10 {
                n1475 = local write "Flush Pump 2"(FALSE ("Flush Pump 1")) -> ()
                n1476 = Concatenate Strings("enter main ", "\r") -> (w2363:string)
                n1477 = VISA Write(VISA resource name=w2362, write buffer=w2363, error in (no error)=w2361) -> (VISA resource name out=w2360:refnum<visa-resource-name>, error out=w2359:errorcluster)  [unwired: 1 out]
                n1478 = VISA Close(VISA resource name=w2360, error in (no error)=w2359) -> ()  [unwired: 1 out]
              }
            }
            n1479 = Concatenate Strings("set units 4 ", w2283) -> (w2296:string)
            n1480 = Multiply(x="Flush \nRate (ul/min)  2", y=60) -> (x*y=w2294:dbl)
            n1481 = Number To Decimal String(number=w2294) -> (decimal integer string=w2297:string)  [unwired: 1 in]
            n1482 = Concatenate Strings("set rate ", w2297, w2283) -> (w2299:string)
            n1483 = Number To Decimal String(number="Flush\nVolume (ul)  2") -> (decimal integer string=w2301:string)  [unwired: 1 in]
            n1484 = Concatenate Strings("set volume ", w2301, w2283) -> (w2302:string)
          }
          event "Stop": Value Change {
            n1485 = event-data() -> ()  [unwired: 1 in, 5 out]
            n1486 = local read "Stop"() -> (w2367:bool)
          }
          event "Inject Pump 2": Value Change {
            n1487 = event-data() -> ()  [unwired: 1 in, 5 out]
            n1488 = case shown="True" "Inject Pump 2" {
              tunnel: w2368 -> [w2371 w2413]
              frame False {
                n1489 = local read "Write Wait"() -> (w2370:i32)
                n1490 = call-poly "VISA Configure Serial Port"("VISA resource name"=w2371) -> ("VISA resource name out"=w2375:refnum<visa-resource-name>, "error out"=w2376:errorcluster)  [unwired: 13 in]
                n1491 = Concatenate Strings("enter pump2", "\r") -> (w2373:string)
                n1492 = flat-sequence {
                  tunnel: w2376 -> [w2387]
                  tunnel: w2375 -> [w2389]
                  tunnel: [w2388] -> w2384
                  tunnel: [w2386] -> w2383
                  tunnel: w2373 -> [w2385]
                  tunnel: w2384 -> [w2392]
                  tunnel: w2383 -> [w2391]
                  tunnel: [w2392] -> w2382
                  tunnel: [w2391] -> w2381
                  tunnel: w2370 -> [w2390]
                  tunnel: [w2396] -> w2380
                  tunnel: [w2395] -> w2379
                  tunnel: w2382 -> [w2394]
                  tunnel: w2381 -> [w2393]
                  tunnel: w2380 -> [w2402]
                  tunnel: [w2402] -> w2378
                  tunnel: w2379 -> [w2401]
                  tunnel: [w2401] -> w2377
                  tunnel: w2370 -> [w2400]
                  tunnel: w2378 -> [w2406]
                  tunnel: w2377 -> [w2405]
                  frame #0 {
                    n1493 = VISA Write(VISA resource name=w2389, write buffer=w2385, error in (no error)=w2387) -> (VISA resource name out=w2388:refnum<visa-resource-name>, error out=w2386:errorcluster)  [unwired: 1 out]
                  }
                  frame #1 {
                    n1494 = Wait (ms)(milliseconds to wait=w2390) -> ()  [unwired: 1 out]
                  }
                  frame #2 {
                    n1495 = Concatenate Strings("stop ", "\r") -> (w2399:string)
                    n1496 = VISA Write(VISA resource name=w2394, write buffer=w2399, error in (no error)=w2393) -> (VISA resource name out=w2396:refnum<visa-resource-name>, error out=w2395:errorcluster)  [unwired: 1 out]
                  }
                  frame #3 {
                    n1497 = Wait (ms)(milliseconds to wait=w2400) -> ()  [unwired: 1 out]
                  }
                  frame #4 {
                    n1498 = Concatenate Strings("enter main ", "\r") -> (w2407:string)
                    n1499 = VISA Write(VISA resource name=w2406, write buffer=w2407, error in (no error)=w2405) -> (VISA resource name out=w2404:refnum<visa-resource-name>, error out=w2403:errorcluster)  [unwired: 1 out]
                    n1500 = VISA Close(VISA resource name=w2404, error in (no error)=w2403) -> ()  [unwired: 1 out]
                  }
                }
              }
              frame True {
                w2426 = "\r"
                n1501 = call-poly "VISA Configure Serial Port"("VISA resource name"=w2413) -> ("VISA resource name out"=w2415:refnum<visa-resource-name>, "error out"=w2414:errorcluster)  [unwired: 13 in]
                n1502 = local read "Write Wait"() -> (w2410:i32)
                n1503 = Concatenate Strings("enter pump2", w2426) -> (w2425:string)
                n1504 = flat-sequence {
                  tunnel: w2414 -> [w2449]
                  tunnel: w2415 -> [w2451]
                  tunnel: [w2450] -> w2446
                  tunnel: [w2448] -> w2445
                  tunnel: w2425 -> [w2447]
                  tunnel: w2446 -> [w2454]
                  tunnel: [w2454] -> w2444
                  tunnel: w2445 -> [w2453]
                  tunnel: [w2453] -> w2443
                  tunnel: w2410 -> [w2452]
                  tunnel: [w2459] -> w2442
                  tunnel: w2422 -> [w2458]
                  tunnel: [w2455] -> w2441
                  tunnel: w2444 -> [w2457]
                  tunnel: w2443 -> [w2456]
                  tunnel: w2442 -> [w2462]
                  tunnel: [w2462] -> w2440
                  tunnel: [w2461] -> w2439
                  tunnel: w2441 -> [w2461]
                  tunnel: w2410 -> [w2460]
                  tunnel: w2440 -> [w2467]
                  tunnel: [w2466] -> w2438
                  tunnel: w2419 -> [w2465]
                  tunnel: w2439 -> [w2464]
                  tunnel: [w2463] -> w2437
                  tunnel: w2438 -> [w2470]
                  tunnel: [w2470] -> w2436
                  tunnel: [w2469] -> w2435
                  tunnel: w2437 -> [w2469]
                  tunnel: w2410 -> [w2468]
                  tunnel: w2436 -> [w2475]
                  tunnel: [w2474] -> w2434
                  tunnel: w2416 -> [w2473]
                  tunnel: w2435 -> [w2472]
                  tunnel: [w2471] -> w2433
                  tunnel: [w2478] -> w2432
                  tunnel: w2434 -> [w2478]
                  tunnel: [w2477] -> w2431
                  tunnel: w2433 -> [w2477]
                  tunnel: w2410 -> [w2476]
                  tunnel: w2432 -> [w2485]
                  tunnel: w2431 -> [w2484]
                  tunnel: [w2480] -> w2430
                  tunnel: [w2479] -> w2429
                  tunnel: w2430 -> [w2488]
                  tunnel: [w2488] -> w2428
                  tunnel: w2429 -> [w2487]
                  tunnel: [w2487] -> w2427
                  tunnel: w2410 -> [w2486]
                  tunnel: w2428 -> [w2492]
                  tunnel: w2427 -> [w2491]
                  frame #0 {
                    n1505 = VISA Write(VISA resource name=w2451, write buffer=w2447, error in (no error)=w2449) -> (VISA resource name out=w2450:refnum<visa-resource-name>, error out=w2448:errorcluster)  [unwired: 1 out]
                  }
                  frame #1 {
                    n1506 = Wait (ms)(milliseconds to wait=w2452) -> ()  [unwired: 1 out]
                  }
                  frame #2 {
                    n1507 = VISA Write(VISA resource name=w2457, write buffer=w2458, error in (no error)=w2456) -> (VISA resource name out=w2459:refnum<visa-resource-name>, error out=w2455:errorcluster)  [unwired: 1 out]
                  }
                  frame #3 {
                    n1508 = Wait (ms)(milliseconds to wait=w2460) -> ()  [unwired: 1 out]
                  }
                  frame #4 {
                    n1509 = VISA Write(VISA resource name=w2467, write buffer=w2465, error in (no error)=w2464) -> (VISA resource name out=w2466:refnum<visa-resource-name>, error out=w2463:errorcluster)  [unwired: 1 out]
                  }
                  frame #5 {
                    n1510 = Wait (ms)(milliseconds to wait=w2468) -> ()  [unwired: 1 out]
                  }
                  frame #6 {
                    n1511 = VISA Write(VISA resource name=w2475, write buffer=w2473, error in (no error)=w2472) -> (VISA resource name out=w2474:refnum<visa-resource-name>, error out=w2471:errorcluster)  [unwired: 1 out]
                  }
                  frame #7 {
                    n1512 = Wait (ms)(milliseconds to wait=w2476) -> ()  [unwired: 1 out]
                  }
                  frame #8 {
                    n1513 = Concatenate Strings("start ", "\r") -> (w2483:string)
                    n1514 = VISA Write(VISA resource name=w2485, write buffer=w2483, error in (no error)=w2484) -> (VISA resource name out=w2480:refnum<visa-resource-name>, error out=w2479:errorcluster)  [unwired: 1 out]
                  }
                  frame #9 {
                    n1515 = Wait (ms)(milliseconds to wait=w2486) -> ()  [unwired: 1 out]
                  }
                  frame #10 {
                    n1516 = Concatenate Strings("enter main ", "\r") -> (w2493:string)
                    n1517 = VISA Write(VISA resource name=w2492, write buffer=w2493, error in (no error)=w2491) -> (VISA resource name out=w2490:refnum<visa-resource-name>, error out=w2489:errorcluster)  [unwired: 1 out]
                    n1518 = VISA Close(VISA resource name=w2490, error in (no error)=w2489) -> ()  [unwired: 1 out]
                  }
                }
                n1519 = local read "Normal \nRate (ul/hr)  2"() -> (w2411:dbl)
                n1520 = Concatenate Strings("set units 4 ", w2426) -> (w2422:string)
                n1521 = local read "Normal \nVolume (ul) 2"() -> (w2412:dbl)
                n1522 = Number To Decimal String(number=w2411) -> (decimal integer string=w2421:string)  [unwired: 1 in]
                n1523 = Concatenate Strings("set rate ", w2421, w2426) -> (w2419:string)
                n1524 = Number To Decimal String(number=w2412) -> (decimal integer string=w2417:string)  [unwired: 1 in]
                n1525 = Concatenate Strings("set volume ", w2417, w2426) -> (w2416:string)
              }
            }
          }
          event "Inject Pump 1": Value Change {
            n1526 = event-data() -> ()  [unwired: 1 in, 5 out]
            n1527 = case shown="True" "Inject Pump 1" {
              tunnel: w2496 -> [w2499 w2541]
              frame False {
                n1528 = local read "Write Wait"() -> (w2498:i32)
                n1529 = call-poly "VISA Configure Serial Port"("VISA resource name"=w2499) -> ("VISA resource name out"=w2503:refnum<visa-resource-name>, "error out"=w2504:errorcluster)  [unwired: 13 in]
                n1530 = Concatenate Strings("enter pump1", "\r") -> (w2501:string)
                n1531 = flat-sequence {
                  tunnel: w2504 -> [w2515]
                  tunnel: w2503 -> [w2517]
                  tunnel: [w2516] -> w2512
                  tunnel: [w2514] -> w2511
                  tunnel: w2501 -> [w2513]
                  tunnel: w2512 -> [w2520]
                  tunnel: w2511 -> [w2519]
                  tunnel: [w2520] -> w2510
                  tunnel: [w2519] -> w2509
                  tunnel: w2498 -> [w2518]
                  tunnel: [w2524] -> w2508
                  tunnel: [w2523] -> w2507
                  tunnel: w2510 -> [w2522]
                  tunnel: w2509 -> [w2521]
                  tunnel: w2508 -> [w2530]
                  tunnel: [w2530] -> w2506
                  tunnel: w2507 -> [w2529]
                  tunnel: [w2529] -> w2505
                  tunnel: w2498 -> [w2528]
                  tunnel: w2506 -> [w2534]
                  tunnel: w2505 -> [w2533]
                  frame #0 {
                    n1532 = VISA Write(VISA resource name=w2517, write buffer=w2513, error in (no error)=w2515) -> (VISA resource name out=w2516:refnum<visa-resource-name>, error out=w2514:errorcluster)  [unwired: 1 out]
                  }
                  frame #1 {
                    n1533 = Wait (ms)(milliseconds to wait=w2518) -> ()  [unwired: 1 out]
                  }
                  frame #2 {
                    n1534 = Concatenate Strings("stop ", "\r") -> (w2527:string)
                    n1535 = VISA Write(VISA resource name=w2522, write buffer=w2527, error in (no error)=w2521) -> (VISA resource name out=w2524:refnum<visa-resource-name>, error out=w2523:errorcluster)  [unwired: 1 out]
                  }
                  frame #3 {
                    n1536 = Wait (ms)(milliseconds to wait=w2528) -> ()  [unwired: 1 out]
                  }
                  frame #4 {
                    n1537 = Concatenate Strings("enter main ", "\r") -> (w2535:string)
                    n1538 = VISA Write(VISA resource name=w2534, write buffer=w2535, error in (no error)=w2533) -> (VISA resource name out=w2532:refnum<visa-resource-name>, error out=w2531:errorcluster)  [unwired: 1 out]
                    n1539 = VISA Close(VISA resource name=w2532, error in (no error)=w2531) -> ()  [unwired: 1 out]
                  }
                }
              }
              frame True {
                w2554 = "\r"
                n1540 = call-poly "VISA Configure Serial Port"("VISA resource name"=w2541) -> ("VISA resource name out"=w2543:refnum<visa-resource-name>, "error out"=w2542:errorcluster)  [unwired: 13 in]
                n1541 = local read "Write Wait"() -> (w2538:i32)
                n1542 = flat-sequence {
                  tunnel: w2542 -> [w2577]
                  tunnel: w2543 -> [w2579]
                  tunnel: [w2578] -> w2574
                  tunnel: [w2576] -> w2573
                  tunnel: w2553 -> [w2575]
                  tunnel: w2574 -> [w2582]
                  tunnel: [w2582] -> w2572
                  tunnel: w2573 -> [w2581]
                  tunnel: [w2581] -> w2571
                  tunnel: w2538 -> [w2580]
                  tunnel: [w2587] -> w2570
                  tunnel: w2550 -> [w2586]
                  tunnel: [w2583] -> w2569
                  tunnel: w2572 -> [w2585]
                  tunnel: w2571 -> [w2584]
                  tunnel: w2570 -> [w2590]
                  tunnel: [w2590] -> w2568
                  tunnel: [w2589] -> w2567
                  tunnel: w2569 -> [w2589]
                  tunnel: w2538 -> [w2588]
                  tunnel: w2568 -> [w2595]
                  tunnel: [w2594] -> w2566
                  tunnel: w2547 -> [w2593]
                  tunnel: w2567 -> [w2592]
                  tunnel: [w2591] -> w2565
                  tunnel: w2566 -> [w2598]
                  tunnel: [w2598] -> w2564
                  tunnel: [w2597] -> w2563
                  tunnel: w2565 -> [w2597]
                  tunnel: w2538 -> [w2596]
                  tunnel: w2564 -> [w2603]
                  tunnel: [w2602] -> w2562
                  tunnel: w2544 -> [w2601]
                  tunnel: w2563 -> [w2600]
                  tunnel: [w2599] -> w2561
                  tunnel: [w2606] -> w2560
                  tunnel: w2562 -> [w2606]
                  tunnel: [w2605] -> w2559
                  tunnel: w2561 -> [w2605]
                  tunnel: w2538 -> [w2604]
                  tunnel: w2560 -> [w2613]
                  tunnel: w2559 -> [w2612]
                  tunnel: [w2608] -> w2558
                  tunnel: [w2607] -> w2557
                  tunnel: w2558 -> [w2616]
                  tunnel: [w2616] -> w2556
                  tunnel: w2557 -> [w2615]
                  tunnel: [w2615] -> w2555
                  tunnel: w2538 -> [w2614]
                  tunnel: w2556 -> [w2620]
                  tunnel: w2555 -> [w2619]
                  frame #0 {
                    n1543 = VISA Write(VISA resource name=w2579, write buffer=w2575, error in (no error)=w2577) -> (VISA resource name out=w2578:refnum<visa-resource-name>, error out=w2576:errorcluster)  [unwired: 1 out]
                  }
                  frame #1 {
                    n1544 = Wait (ms)(milliseconds to wait=w2580) -> ()  [unwired: 1 out]
                  }
                  frame #2 {
                    n1545 = VISA Write(VISA resource name=w2585, write buffer=w2586, error in (no error)=w2584) -> (VISA resource name out=w2587:refnum<visa-resource-name>, error out=w2583:errorcluster)  [unwired: 1 out]
                  }
                  frame #3 {
                    n1546 = Wait (ms)(milliseconds to wait=w2588) -> ()  [unwired: 1 out]
                  }
                  frame #4 {
                    n1547 = VISA Write(VISA resource name=w2595, write buffer=w2593, error in (no error)=w2592) -> (VISA resource name out=w2594:refnum<visa-resource-name>, error out=w2591:errorcluster)  [unwired: 1 out]
                  }
                  frame #5 {
                    n1548 = Wait (ms)(milliseconds to wait=w2596) -> ()  [unwired: 1 out]
                  }
                  frame #6 {
                    n1549 = VISA Write(VISA resource name=w2603, write buffer=w2601, error in (no error)=w2600) -> (VISA resource name out=w2602:refnum<visa-resource-name>, error out=w2599:errorcluster)  [unwired: 1 out]
                  }
                  frame #7 {
                    n1550 = Wait (ms)(milliseconds to wait=w2604) -> ()  [unwired: 1 out]
                  }
                  frame #8 {
                    n1551 = Concatenate Strings("start ", "\r") -> (w2611:string)
                    n1552 = VISA Write(VISA resource name=w2613, write buffer=w2611, error in (no error)=w2612) -> (VISA resource name out=w2608:refnum<visa-resource-name>, error out=w2607:errorcluster)  [unwired: 1 out]
                  }
                  frame #9 {
                    n1553 = Wait (ms)(milliseconds to wait=w2614) -> ()  [unwired: 1 out]
                  }
                  frame #10 {
                    n1554 = Concatenate Strings("enter main ", "\r") -> (w2621:string)
                    n1555 = VISA Write(VISA resource name=w2620, write buffer=w2621, error in (no error)=w2619) -> (VISA resource name out=w2618:refnum<visa-resource-name>, error out=w2617:errorcluster)  [unwired: 1 out]
                    n1556 = VISA Close(VISA resource name=w2618, error in (no error)=w2617) -> ()  [unwired: 1 out]
                  }
                }
                n1557 = Concatenate Strings("enter pump1", w2554) -> (w2553:string)
                n1558 = local read "Normal \nRate (ul/hr)"() -> (w2539:dbl)
                n1559 = Concatenate Strings("set units 4 ", w2554) -> (w2550:string)
                n1560 = local read "Normal \nVolume (ul)"() -> (w2540:dbl)
                n1561 = Number To Decimal String(number=w2539) -> (decimal integer string=w2549:string)  [unwired: 1 in]
                n1562 = Concatenate Strings("set rate ", w2549, w2554) -> (w2547:string)
                n1563 = Number To Decimal String(number=w2540) -> (decimal integer string=w2545:string)  [unwired: 1 in]
                n1564 = Concatenate Strings("set volume ", w2545, w2554) -> (w2544:string)
              }
            }
          }
          event "Normal \nVolume (ul)": Value Change {
            n1565 = event-data() -> ()  [unwired: 1 in, 5 out]
            n1566 = call-poly "VISA Configure Serial Port"("VISA resource name"=w2639) -> ("VISA resource name out"=w2641:refnum<visa-resource-name>, "error out"=w2640:errorcluster)  [unwired: 13 in]
            n1567 = local read "Write Wait"() -> (w2624:i32)
            n1568 = Concatenate Strings("enter pump1", "\r") -> (w2643:string)
            n1569 = flat-sequence {
              tunnel: w2640 -> [w2653]
              tunnel: w2641 -> [w2655]
              tunnel: [w2654] -> w2633
              tunnel: [w2652] -> w2632
              tunnel: w2643 -> [w2651]
              tunnel: w2633 -> [w2658]
              tunnel: [w2658] -> w2631
              tunnel: w2632 -> [w2657]
              tunnel: [w2657] -> w2629
              tunnel: w2624 -> [w2656]
              tunnel: w2631 -> [w2662]
              tunnel: [w2663] -> w2630
              tunnel: w2629 -> [w2661]
              tunnel: [w2660] -> w2628
              tunnel: w2625 -> [w2659]
              tunnel: w2630 -> [w2666]
              tunnel: w2628 -> [w2665]
              tunnel: [w2666] -> w2650
              tunnel: [w2665] -> w2649
              tunnel: w2624 -> [w2664]
              tunnel: [w2671] -> w2648
              tunnel: [w2670] -> w2647
              tunnel: w2650 -> [w2669]
              tunnel: w2649 -> [w2668]
              tunnel: w2634 -> [w2667]
              tunnel: w2648 -> [w2674]
              tunnel: [w2674] -> w2646
              tunnel: w2647 -> [w2673]
              tunnel: [w2673] -> w2645
              tunnel: w2624 -> [w2672]
              tunnel: w2646 -> [w2678]
              tunnel: w2645 -> [w2677]
              frame #0 {
                n1570 = VISA Write(VISA resource name=w2655, write buffer=w2651, error in (no error)=w2653) -> (VISA resource name out=w2654:refnum<visa-resource-name>, error out=w2652:errorcluster)  [unwired: 1 out]
              }
              frame #1 {
                n1571 = Wait (ms)(milliseconds to wait=w2656) -> ()  [unwired: 1 out]
              }
              frame #2 {
                n1572 = VISA Write(VISA resource name=w2662, write buffer=w2659, error in (no error)=w2661) -> (VISA resource name out=w2663:refnum<visa-resource-name>, error out=w2660:errorcluster)  [unwired: 1 out]
              }
              frame #3 {
                n1573 = Wait (ms)(milliseconds to wait=w2664) -> ()  [unwired: 1 out]
              }
              frame #4 {
                n1574 = VISA Write(VISA resource name=w2669, write buffer=w2667, error in (no error)=w2668) -> (VISA resource name out=w2671:refnum<visa-resource-name>, error out=w2670:errorcluster)  [unwired: 1 out]
              }
              frame #5 {
                n1575 = Wait (ms)(milliseconds to wait=w2672) -> ()  [unwired: 1 out]
              }
              frame #6 {
                n1576 = Concatenate Strings("enter main ", "\r") -> (w2679:string)
                n1577 = VISA Write(VISA resource name=w2678, write buffer=w2679, error in (no error)=w2677) -> (VISA resource name out=w2676:refnum<visa-resource-name>, error out=w2675:errorcluster)  [unwired: 1 out]
                n1578 = VISA Close(VISA resource name=w2676, error in (no error)=w2675) -> ()  [unwired: 1 out]
              }
            }
            n1579 = Concatenate Strings("set units 4", "\r") -> (w2625:string)
            n1580 = Number To Decimal String(number="Normal \nVolume (ul)") -> (decimal integer string=w2636:string)  [unwired: 1 in]
            n1581 = Concatenate Strings("set volume", w2636, "\r") -> (w2634:string)
          }
          event "Normal \nRate (ul/hr)": Value Change {
            n1582 = event-data() -> ()  [unwired: 1 in, 5 out]
            n1583 = call-poly "VISA Configure Serial Port"("VISA resource name"=w2684) -> ("VISA resource name out"=w2692:refnum<visa-resource-name>, "error out"=w2691:errorcluster)  [unwired: 13 in]
            n1584 = local read "Write Wait"() -> (w2682:i32)
            n1585 = Concatenate Strings("enter pump1", "\r") -> (w2694:string)
            n1586 = flat-sequence {
              tunnel: w2691 -> [w2711]
              tunnel: w2692 -> [w2713]
              tunnel: [w2712] -> w2707
              tunnel: [w2710] -> w2706
              tunnel: w2694 -> [w2709]
              tunnel: w2707 -> [w2716]
              tunnel: [w2716] -> w2705
              tunnel: w2706 -> [w2715]
              tunnel: [w2715] -> w2704
              tunnel: w2682 -> [w2714]
              tunnel: w2705 -> [w2720]
              tunnel: [w2721] -> w2703
              tunnel: w2704 -> [w2719]
              tunnel: [w2718] -> w2702
              tunnel: w2685 -> [w2717]
              tunnel: w2703 -> [w2724]
              tunnel: w2702 -> [w2723]
              tunnel: [w2724] -> w2701
              tunnel: [w2723] -> w2700
              tunnel: w2682 -> [w2722]
              tunnel: [w2729] -> w2699
              tunnel: [w2728] -> w2698
              tunnel: w2701 -> [w2727]
              tunnel: w2700 -> [w2726]
              tunnel: w2688 -> [w2725]
              tunnel: w2699 -> [w2732]
              tunnel: [w2732] -> w2697
              tunnel: w2698 -> [w2731]
              tunnel: [w2731] -> w2696
              tunnel: w2682 -> [w2730]
              tunnel: w2697 -> [w2736]
              tunnel: w2696 -> [w2735]
              frame #0 {
                n1587 = VISA Write(VISA resource name=w2713, write buffer=w2709, error in (no error)=w2711) -> (VISA resource name out=w2712:refnum<visa-resource-name>, error out=w2710:errorcluster)  [unwired: 1 out]
              }
              frame #1 {
                n1588 = Wait (ms)(milliseconds to wait=w2714) -> ()  [unwired: 1 out]
              }
              frame #2 {
                n1589 = VISA Write(VISA resource name=w2720, write buffer=w2717, error in (no error)=w2719) -> (VISA resource name out=w2721:refnum<visa-resource-name>, error out=w2718:errorcluster)  [unwired: 1 out]
              }
              frame #3 {
                n1590 = Wait (ms)(milliseconds to wait=w2722) -> ()  [unwired: 1 out]
              }
              frame #4 {
                n1591 = VISA Write(VISA resource name=w2727, write buffer=w2725, error in (no error)=w2726) -> (VISA resource name out=w2729:refnum<visa-resource-name>, error out=w2728:errorcluster)  [unwired: 1 out]
              }
              frame #5 {
                n1592 = Wait (ms)(milliseconds to wait=w2730) -> ()  [unwired: 1 out]
              }
              frame #6 {
                n1593 = Concatenate Strings("enter main ", "\r") -> (w2737:string)
                n1594 = VISA Write(VISA resource name=w2736, write buffer=w2737, error in (no error)=w2735) -> (VISA resource name out=w2734:refnum<visa-resource-name>, error out=w2733:errorcluster)  [unwired: 1 out]
                n1595 = VISA Close(VISA resource name=w2734, error in (no error)=w2733) -> ()  [unwired: 1 out]
              }
            }
            n1596 = Concatenate Strings("set units 4", "\r") -> (w2685:string)
            n1597 = Number To Decimal String(number="Normal \nRate (ul/hr)") -> (decimal integer string=w2683:string)  [unwired: 1 in]
            n1598 = Concatenate Strings("set rate", w2683, "\r") -> (w2688:string)
          }
          event "Normal \nRate (ul/hr)  2": Value Change {
            n1599 = event-data() -> ()  [unwired: 1 in, 5 out]
            n1600 = call-poly "VISA Configure Serial Port"("VISA resource name"=w2742) -> ("VISA resource name out"=w2750:refnum<visa-resource-name>, "error out"=w2749:errorcluster)  [unwired: 13 in]
            n1601 = local read "Write Wait"() -> (w2740:i32)
            n1602 = Concatenate Strings("enter pump2", "\r") -> (w2752:string)
            n1603 = flat-sequence {
              tunnel: w2749 -> [w2769]
              tunnel: w2750 -> [w2771]
              tunnel: [w2770] -> w2765
              tunnel: [w2768] -> w2764
              tunnel: w2752 -> [w2767]
              tunnel: w2765 -> [w2774]
              tunnel: [w2774] -> w2763
              tunnel: w2764 -> [w2773]
              tunnel: [w2773] -> w2762
              tunnel: w2740 -> [w2772]
              tunnel: w2763 -> [w2778]
              tunnel: [w2779] -> w2761
              tunnel: w2762 -> [w2777]
              tunnel: [w2776] -> w2760
              tunnel: w2743 -> [w2775]
              tunnel: w2761 -> [w2782]
              tunnel: w2760 -> [w2781]
              tunnel: [w2782] -> w2759
              tunnel: [w2781] -> w2758
              tunnel: w2740 -> [w2780]
              tunnel: [w2787] -> w2757
              tunnel: [w2786] -> w2756
              tunnel: w2759 -> [w2785]
              tunnel: w2758 -> [w2784]
              tunnel: w2746 -> [w2783]
              tunnel: w2757 -> [w2790]
              tunnel: [w2790] -> w2755
              tunnel: w2756 -> [w2789]
              tunnel: [w2789] -> w2754
              tunnel: w2740 -> [w2788]
              tunnel: w2755 -> [w2794]
              tunnel: w2754 -> [w2793]
              frame #0 {
                n1604 = VISA Write(VISA resource name=w2771, write buffer=w2767, error in (no error)=w2769) -> (VISA resource name out=w2770:refnum<visa-resource-name>, error out=w2768:errorcluster)  [unwired: 1 out]
              }
              frame #1 {
                n1605 = Wait (ms)(milliseconds to wait=w2772) -> ()  [unwired: 1 out]
              }
              frame #2 {
                n1606 = VISA Write(VISA resource name=w2778, write buffer=w2775, error in (no error)=w2777) -> (VISA resource name out=w2779:refnum<visa-resource-name>, error out=w2776:errorcluster)  [unwired: 1 out]
              }
              frame #3 {
                n1607 = Wait (ms)(milliseconds to wait=w2780) -> ()  [unwired: 1 out]
              }
              frame #4 {
                n1608 = VISA Write(VISA resource name=w2785, write buffer=w2783, error in (no error)=w2784) -> (VISA resource name out=w2787:refnum<visa-resource-name>, error out=w2786:errorcluster)  [unwired: 1 out]
              }
              frame #5 {
                n1609 = Wait (ms)(milliseconds to wait=w2788) -> ()  [unwired: 1 out]
              }
              frame #6 {
                n1610 = Concatenate Strings("enter main ", "\r") -> (w2795:string)
                n1611 = VISA Write(VISA resource name=w2794, write buffer=w2795, error in (no error)=w2793) -> (VISA resource name out=w2792:refnum<visa-resource-name>, error out=w2791:errorcluster)  [unwired: 1 out]
                n1612 = VISA Close(VISA resource name=w2792, error in (no error)=w2791) -> ()  [unwired: 1 out]
              }
            }
            n1613 = Concatenate Strings("set units 4", "\r") -> (w2743:string)
            n1614 = Number To Decimal String(number="Normal \nRate (ul/hr)  2") -> (decimal integer string=w2741:string)  [unwired: 1 in]
            n1615 = Concatenate Strings("set rate", w2741, "\r") -> (w2746:string)
          }
          event "Normal \nVolume (ul) 2": Value Change {
            n1616 = event-data() -> ()  [unwired: 1 in, 5 out]
            n1617 = call-poly "VISA Configure Serial Port"("VISA resource name"=w2801) -> ("VISA resource name out"=w2805:refnum<visa-resource-name>, "error out"=w2806:errorcluster)  [unwired: 13 in]
            n1618 = local read "Write Wait"() -> (w2798:i32)
            n1619 = Concatenate Strings("enter pump2", "\r") -> (w2803:string)
            n1620 = flat-sequence {
              tunnel: w2806 -> [w2827]
              tunnel: w2805 -> [w2829]
              tunnel: [w2828] -> w2824
              tunnel: [w2826] -> w2823
              tunnel: w2803 -> [w2825]
              tunnel: w2824 -> [w2832]
              tunnel: [w2832] -> w2822
              tunnel: w2823 -> [w2831]
              tunnel: [w2831] -> w2821
              tunnel: w2798 -> [w2830]
              tunnel: w2822 -> [w2836]
              tunnel: [w2837] -> w2820
              tunnel: w2821 -> [w2835]
              tunnel: [w2834] -> w2819
              tunnel: w2812 -> [w2833]
              tunnel: w2820 -> [w2840]
              tunnel: w2819 -> [w2839]
              tunnel: [w2840] -> w2818
              tunnel: [w2839] -> w2817
              tunnel: w2798 -> [w2838]
              tunnel: [w2845] -> w2816
              tunnel: [w2844] -> w2815
              tunnel: w2818 -> [w2843]
              tunnel: w2817 -> [w2842]
              tunnel: w2809 -> [w2841]
              tunnel: w2816 -> [w2848]
              tunnel: [w2848] -> w2814
              tunnel: w2815 -> [w2847]
              tunnel: [w2847] -> w2813
              tunnel: w2798 -> [w2846]
              tunnel: w2814 -> [w2852]
              tunnel: w2813 -> [w2851]
              frame #0 {
                n1621 = VISA Write(VISA resource name=w2829, write buffer=w2825, error in (no error)=w2827) -> (VISA resource name out=w2828:refnum<visa-resource-name>, error out=w2826:errorcluster)  [unwired: 1 out]
              }
              frame #1 {
                n1622 = Wait (ms)(milliseconds to wait=w2830) -> ()  [unwired: 1 out]
              }
              frame #2 {
                n1623 = VISA Write(VISA resource name=w2836, write buffer=w2833, error in (no error)=w2835) -> (VISA resource name out=w2837:refnum<visa-resource-name>, error out=w2834:errorcluster)  [unwired: 1 out]
              }
              frame #3 {
                n1624 = Wait (ms)(milliseconds to wait=w2838) -> ()  [unwired: 1 out]
              }
              frame #4 {
                n1625 = VISA Write(VISA resource name=w2843, write buffer=w2841, error in (no error)=w2842) -> (VISA resource name out=w2845:refnum<visa-resource-name>, error out=w2844:errorcluster)  [unwired: 1 out]
              }
              frame #5 {
                n1626 = Wait (ms)(milliseconds to wait=w2846) -> ()  [unwired: 1 out]
              }
              frame #6 {
                n1627 = Concatenate Strings("enter main ", "\r") -> (w2853:string)
                n1628 = VISA Write(VISA resource name=w2852, write buffer=w2853, error in (no error)=w2851) -> (VISA resource name out=w2850:refnum<visa-resource-name>, error out=w2849:errorcluster)  [unwired: 1 out]
                n1629 = VISA Close(VISA resource name=w2850, error in (no error)=w2849) -> ()  [unwired: 1 out]
              }
            }
            n1630 = Concatenate Strings("set units 4", "\r") -> (w2812:string)
            n1631 = Number To Decimal String(number="Normal \nVolume (ul) 2") -> (decimal integer string=w2799:string)  [unwired: 1 in]
            n1632 = Concatenate Strings("set volume", w2799, "\r") -> (w2809:string)
          }
        }
        n1633 = node-c288() -> ()  [unwired: 1 in, 1 out]
      }
      n1634 = node-c288(w2185) -> ()  [unwired: 1 out]
    }
    frame Enabled {
      n1635 = node-c288(2 ("Processor")) -> (w2865:T13)  [unwired: 3 in]
      n1636 = timed-loop "Pump Control" {
        timing: w2865 -> [_]
        timing-out: [_] -> w2864
        tunnel: refnum<visa-resource-name> "COM4" ("VISA resource name") -> [w2867]
        stop <- w2866 stop-if-true
        n1637 = node-c288() -> ()  [unwired: 1 in, 1 out]
        n1638 = event shown="[2] \"Inject Sample\": Value Change" {
          selector: _ -> [_ _ _ _ _]
          dyn-events: _ -> [_ _ _ _ _]
          timeout: _ -> [_ _ _ _ _]
          tunnel: w2867 -> [w2873 _ w2947 w2974 w2979]
          tunnel: [_ w2945 _ _ _] -> w2866
          event "Flush Sample": Value Change {
            n1639 = event-data() -> ()  [unwired: 1 in, 5 out]
            n1640 = local read "Write Wait"() -> (w2887:i32)
            n1641 = flat-sequence {
              tunnel: [w2911] -> w2907
              tunnel: [w2910] -> w2906
              tunnel: "CLD" -> [w2909]
              tunnel: w2873 -> [w2908]
              tunnel: w2907 -> [w2914]
              tunnel: [w2914] -> w2905
              tunnel: w2906 -> [w2913]
              tunnel: [w2913] -> w2904
              tunnel: w2887 -> [w2912]
              tunnel: [w2919] -> w2903
              tunnel: [w2916] -> w2902
              tunnel: w2905 -> [w2918]
              tunnel: w2904 -> [w2917]
              tunnel: "MODVOL" -> [w2915]
              tunnel: w2903 -> [w2922]
              tunnel: [w2922] -> w2901
              tunnel: [w2921] -> w2900
              tunnel: w2902 -> [w2921]
              tunnel: w2887 -> [w2920]
              tunnel: w2901 -> [w2927]
              tunnel: [w2926] -> w2899
              tunnel: w2889 -> [w2925]
              tunnel: w2900 -> [w2924]
              tunnel: [w2923] -> w2898
              tunnel: w2899 -> [w2930]
              tunnel: [w2930] -> w2897
              tunnel: [w2929] -> w2896
              tunnel: w2898 -> [w2929]
              tunnel: w2887 -> [w2928]
              tunnel: w2897 -> [w2935]
              tunnel: [w2934] -> w2895
              tunnel: w2891 -> [w2933]
              tunnel: w2896 -> [w2932]
              tunnel: [w2931] -> w2894
              tunnel: [w2938] -> w2892
              tunnel: w2895 -> [w2938]
              tunnel: [w2937] -> w2893
              tunnel: w2894 -> [w2937]
              tunnel: w2887 -> [w2936]
              tunnel: w2893 -> [w2943]
              tunnel: w2892 -> [w2944]
              tunnel: [w2942] -> w2882
              tunnel: "RUN " -> [w2941]
              frame #0 {
                n1642 = call "Write to pump 2.vi"("String to write"=w2909, "VISA resource name"=w2908) -> ("error out"=w2910:errorcluster, "VISA resource name out"=w2911:refnum<visa-resource-name>)  [unwired: 8 in]
              }
              frame #1 {
                n1643 = Wait (ms)(milliseconds to wait=w2912) -> ()  [unwired: 1 out]
              }
              frame #2 {
                n1644 = call "Write to pump 2.vi"("error in (no error)"=w2917, "String to write"=w2915, "VISA resource name"=w2918) -> ("error out"=w2916:errorcluster, "VISA resource name out"=w2919:refnum<visa-resource-name>)  [unwired: 7 in]
              }
              frame #3 {
                n1645 = Wait (ms)(milliseconds to wait=w2920) -> ()  [unwired: 1 out]
              }
              frame #4 {
                n1646 = call "Write to pump 2.vi"("error in (no error)"=w2924, "String to write"=w2925, "VISA resource name"=w2927) -> ("error out"=w2923:errorcluster, "VISA resource name out"=w2926:refnum<visa-resource-name>)  [unwired: 7 in]
              }
              frame #5 {
                n1647 = Wait (ms)(milliseconds to wait=w2928) -> ()  [unwired: 1 out]
              }
              frame #6 {
                n1648 = call "Write to pump 2.vi"("error in (no error)"=w2932, "String to write"=w2933, "VISA resource name"=w2935) -> ("error out"=w2931:errorcluster, "VISA resource name out"=w2934:refnum<visa-resource-name>)  [unwired: 7 in]
              }
              frame #7 {
                n1649 = Wait (ms)(milliseconds to wait=w2936) -> ()  [unwired: 1 out]
              }
              frame #8 {
                w2940 = TRUE ("Inject Pump 3")
                n1650 = Tick Count (ms)() -> (millisecond timer value=→"Flush Sample Start Time":u32)
                n1651 = call "Write to pump 2.vi"("error in (no error)"=w2943, "String to write"=w2941, "VISA resource name"=w2944) -> ("error out"=w2942:errorcluster)  [unwired: 7 in, 1 out]
                n1652 = local write "Inject Sample"(w2940) -> ()
                "Flushing Sample" <- w2940
              }
            }
            n1653 = Number To Fractional String(number="Flush \nRate (ul/min)  3") -> (F-format string=w2875:string)  [unwired: 3 in]
            n1654 = String Subset(string=w2875, length (rest)=6 ("length (rest)")) -> (substring=w2874:string)  [unwired: 1 in]
            n1655 = Concatenate Strings("RAT", w2874, "UM") -> (w2889:string)
            n1656 = Divide(x="Flush\nVolume (ul)  3", y=1000.0) -> (x/y=w2880:dbl)
            n1657 = Number To Fractional String(number=w2880) -> (F-format string=w2879:string)  [unwired: 3 in]
            n1658 = Divide(x="Flush\nVolume (ul)  3", y="Flush \nRate (ul/min)  3") -> (x/y=w2870:dbl)
            n1659 = Multiply(x=w2870, y=60.0) -> (x*y=→"Sample flush time (s)":dbl)
            n1660 = String Subset(string=w2879, length (rest)=6 ("length (rest)")) -> (substring=w2878:string)  [unwired: 1 in]
            n1661 = Concatenate Strings("TGT", w2878) -> (w2891:string)
            "error out" <- w2882
          }
          event "Stop": Value Change {
            n1662 = event-data() -> ()  [unwired: 1 in, 5 out]
            n1663 = local read "Stop"() -> (w2945:bool)
          }
          event "Inject Sample": Value Change {
            n1664 = event-data() -> ()  [unwired: 1 in, 5 out]
            n1665 = case shown="True" "Inject Sample" {
              tunnel: w2947 -> [w2949 w2950]
              frame False {
                n1666 = call "Write to pump 2.vi"("String to write"="STP", "VISA resource name"=w2949) -> ()  [unwired: 8 in, 2 out]
              }
              frame True {
                n1667 = local read "Normal \nRate (ul/hr)  3"() -> (w2951:dbl)
                n1668 = Number To Fractional String(number=w2951) -> (F-format string=w2954:string)  [unwired: 3 in]
                n1669 = String Subset(string=w2954, length (rest)=6 ("length (rest)")) -> (substring=w2952:string)  [unwired: 1 in]
                n1670 = flat-sequence {
                  tunnel: "RUN " -> [w2966]
                  tunnel: [w2968] -> _
                  tunnel: [w2967] -> _
                  tunnel: w2950 -> [w2965]
                  frame #0 {
                    n1671 = call "Write to pump 2.vi"("String to write"=w2966, "VISA resource name"=w2965) -> ("error out"=w2967:errorcluster, "VISA resource name out"=w2968:refnum<visa-resource-name>)  [unwired: 8 in]
                  }
                }
                n1672 = Concatenate Strings("RAT", w2952, "UH" ("string")) -> ()  [unwired: 1 out]
                n1673 = local read "Normal \nVolume (ul) 3"() -> (w2960:dbl)
                n1674 = Divide(x=w2960, y=1000.0) -> (x/y=w2955:dbl)
                n1675 = Number To Fractional String(number=w2955) -> (F-format string=w2958:string)  [unwired: 3 in]
                n1676 = String Subset(string=w2958, length (rest)=6 ("length (rest)")) -> (substring=w2956:string)  [unwired: 1 in]
                n1677 = Concatenate Strings("TGT", w2956) -> ()  [unwired: 1 out]
              }
            }
          }
          event "Normal \nRate (ul/hr)  3": Value Change {
            n1678 = event-data() -> ()  [unwired: 1 in, 5 out]
            n1679 = Number To Fractional String(number="Normal \nRate (ul/hr)  3") -> (F-format string=w2972:string)  [unwired: 3 in]
            n1680 = String Subset(string=w2972, length (rest)=6 ("length (rest)")) -> (substring=w2970:string)  [unwired: 1 in]
            n1681 = Concatenate Strings("RAT", w2970, "UH") -> (w2973:string)
            n1682 = call "Write to pump 2.vi"("String to write"=w2973, "VISA resource name"=w2974) -> ()  [unwired: 8 in, 2 out]
          }
          event "Clear Volume": Value Change {
            n1683 = event-data() -> ()  [unwired: 1 in, 5 out]
            n1684 = Divide(x="Normal \nVolume (ul) 3", y=1000.0) -> (x/y=w2992:dbl)
            n1685 = Number To Fractional String(number=w2992) -> (F-format string=w2995:string)  [unwired: 3 in]
            n1686 = String Subset(string=w2995, length (rest)=6 ("length (rest)")) -> (substring=w2993:string)  [unwired: 1 in]
            n1687 = flat-sequence {
              tunnel: [w3002] -> w2990
              tunnel: [w3001] -> w2989
              tunnel: w2979 -> [w3000]
              tunnel: w2978 -> [w2999]
              tunnel: [w3004] -> w2987
              tunnel: [w3003] -> w2988
              tunnel: w2984 -> [w3005]
              tunnel: w2990 -> [w3004]
              tunnel: w2989 -> [w3003]
              tunnel: w2988 -> [w3009]
              tunnel: w2987 -> [w3010]
              tunnel: [w3008] -> _
              tunnel: [w3007] -> _
              tunnel: w2977 -> [w3006]
              frame #0 {
                n1688 = call "Write to pump 2.vi"("String to write"=w2999, "VISA resource name"=w3000) -> ("error out"=w3001:errorcluster, "VISA resource name out"=w3002:refnum<visa-resource-name>)  [unwired: 8 in]
              }
              frame #1 {
                n1689 = Wait (ms)(milliseconds to wait=w3005) -> ()  [unwired: 1 out]
              }
              frame #2 {
                n1690 = call "Write to pump 2.vi"("error in (no error)"=w3009, "String to write"=w3006, "VISA resource name"=w3010) -> ("error out"=w3007:errorcluster, "VISA resource name out"=w3008:refnum<visa-resource-name>)  [unwired: 7 in]
              }
            }
            n1691 = local read "Write Wait"() -> (w2984:i32)
            n1692 = Concatenate Strings("TGT", w2993) -> (w2978:string)
            n1693 = local read "Normal \nRate (ul/hr)  3"() -> (w2980:dbl)
            n1694 = local write "Clear Volume"(FALSE ("Clear Volume")) -> ()
            n1695 = Number To Fractional String(number=w2980) -> (F-format string=w2983:string)  [unwired: 3 in]
            n1696 = String Subset(string=w2983, length (rest)=6 ("length (rest)")) -> (substring=w2981:string)  [unwired: 1 in]
            n1697 = Concatenate Strings("RAT", w2981, "UH" ("string")) -> (w2977:string)
          }
        }
        n1698 = node-c288() -> ()  [unwired: 1 in, 1 out]
      }
      n1699 = node-c288(w2864) -> ()  [unwired: 1 out]
    }
  }
  n1700 = node-c288() -> (w90:T13)  [unwired: 4 in]
  n1701 = timed-loop {
    timing: w90 -> [_]
    timing-out: [_] -> w89
    stop <- w3017 stop-if-true
    n1702 = node-c288() -> ()  [unwired: 1 in, 1 out]
    n1703 = event shown="[1] \"Stop\": Value Change" {
      selector: _ -> [_ _]
      dyn-events: _ -> [_ _]
      timeout: _ -> [_ _]
      tunnel: [_ "Stop"] -> w3017
      event Timeout {
        n1704 = event-data() -> ()  [unwired: 1 in, 2 out]
      }
      event "Stop": Value Change {
        w3018 = FALSE ("Force Feedback")
        n1705 = event-data() -> ()  [unwired: 1 in, 4 out]
        n1706 = property on="Cancel dwell" class="Bool (strict)"("Val(Sgnl)"=TRUE ("Value (Signaling)")) -> ()  [unwired: 2 in, 2 out]
        n1707 = local write "Force Feedback 1"(w3018) -> ()
        n1708 = local write "Force Feedback 2"(w3018) -> ()
      }
    }
    n1709 = node-c288() -> ()  [unwired: 1 in, 1 out]
  }
  n1710 = case shown="True" w80 {
    tunnel: w85 -> [_ w3025]
    tunnel: w84 -> [_ w3024]
    tunnel: w83 -> [_ w3023]
    frame False {
    }
    frame True {
      w3027 = T24 3 items=["no dialog", "OK message", "continue or stop message", "OK message + warnings", "continue/stop + warnings"] ("type of dialog (OK msg:1)")
      w3026 = T24 3 items=["no dialog", "OK message", "continue or stop message", "OK message + warnings", "continue/stop + warnings"] ("type of dialog (OK msg:1)")
      n1711 = call <vilib>:"DAQmx Clear Task.vi"("task in"=w3025, "error in"=w3023) -> ("error out"=w3028:errorcluster)  [unwired: 13 in]
      n1712 = call <vilib>:"DAQmx Clear Task.vi"("task in"=w3024) -> ("error out"=w3029:errorcluster)  [unwired: 14 in]
      n1713 = call <vilib>:"Simple Error Handler.vi"("type of dialog (OK msg:1)"=w3027, "error in (no error)"=w3028) -> ()  [unwired: 3 in, 5 out]
      n1714 = call <vilib>:"Simple Error Handler.vi"("type of dialog (OK msg:1)"=w3026, "error in (no error)"=w3029) -> ()  [unwired: 3 in, 5 out]
    }
  }
  n1715 = case shown="\"Raster scan\"" "?" {
    frame "Force Feedback", Default {
    }
    frame "Raster scan" {
    }
  }
  n1716 = node-c288(w89) -> ()  [unwired: 1 out]
  n1717 = node-c288(w92) -> ()  [unwired: 1 out]
  n1718 = local write "Pause Mouse/Mirror Connection"(FALSE ("Pause Mouse/Mirror Connection")) -> ()
  n1719 = local write "Stop"(FALSE ("Stop all")) -> ()
  "CoordinatesMousePressed" <- T5 {"Horizontal"=0, "Vertical"=0} ("Coords when pressed")
  "Deflection" <- T5 {"Horizontal"=0, "Vertical"=0} ("Coords when pressed")
